vi "Modules - Communications.vi"() -> ()   [LabVIEW 2019]
uses:
  Controls/Communications - State.ctl
  Controls/eFGV States.ctl
  Controls/Communications - Data Structure.ctl
  Controls/FTDI - Communication.ctl
  Controls/Global - Channel.vi
  Controls/Global - Done.vi
  Controls/Global - Unit.vi
  Controls/Global - IP Address.vi
  Controls/Global - Device.vi
  Controls/Global - Handle.vi
  Controls/Global - Comport.vi
  Controls/Global - Hold.vi
  Controls/Global - Rendezvous.vi
  Controls/UDP - Command.ctl
  Controls/Global - ADC.vi
  Controls/Global - PID.vi
  Controls/Communication - Write Data.ctl
  Controls/Global - System.vi
  Controls/Global - Test.vi
panel:
  out "Device":string[](array[string])
  out "IP":string[](array[string])
  out "Stop":bool=TRUE
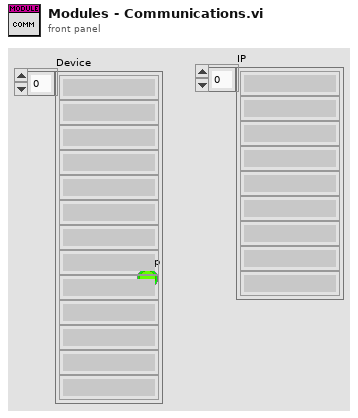
[diagram p1: front panel]
types:
  T1 = typedef "Communications - State.ctl" = enum16{"Init", "Idle", "Command", "Get IP Address", "Release Rendezvous", "Feedback", "Close"}
  T2 = typedef "FTDI - Communication.ctl" = cluster{"IP":string, "CMD":T3, "Port":string, "Datalog?":bool, "Float":dbl}
  T3 = typedef "UDP - Command.ctl" = enum16{"Stop", "Jog Up", "Jog Down", "Ramp Up", "Ramp Down", "PID Target", "PID Ramp", "Disp Run", "Read Ch Data", "Zero Channel", "Zero Disp", "Read Sensor", "Write Sensor", "Read ADC", "Write ADC", "Read PID", "Write PID", "Read Test", "Write Test", "Read System", "Write System", "Read Datalog", "Read Datalog Sensor"}
  T4 = typedef "eFGV States.ctl" = enum16{"Init", "Read", "Write", "Exit"}
  T5 = typedef "Communications - Data Structure.ctl" = cluster{"UDP CMD":T2, "UDP ref":refnum<event-registration>, "Unit?":bool, "Read Unit":bool[], "Trig?":bool, "UDP Info":cluster{"IP Address":string, "port":string, "UDP ref":refnum<k16>}[], "UDP Conn ref":refnum<k16>, "DataLogger":bool[], "VISA Ref":refnum<event-registration>, "Float":sgl, "Data":T6}
  T6 = typedef "Communication - Write Data.ctl" = cluster{"Test":cluster{"Target Load":sgl, "Target Disp":sgl, "Rate":sgl, "Speed":sgl}, "Sensor":cluster{"Name":string[], "Unit":string[], "Decimal Point":u8[], "Ch Log":u8[], "H Alarm":u8[], "L Alarm":u8[], "H Limit":sgl[], "L Limit":sgl[], "Filter":u8[], "Gain":u8[], "Calib Type":u32[]}, "PID":cluster{"SP":sgl, "PV":sgl, "kP":sgl, "kI":sgl, "kD":sgl, "FF":sgl, "Err Band":sgl, "Max":i32, "Min":i32, "Ts":u32, "Out":i32, "Mode":u8}, "ADC":cluster{"Active Ch":u8[], "Filter Type":u8, "Post Filter":u8[], "Gain":u8[], "FS":u16, "IntOC":u8, "IntFC":u8, "SysOC":u8, "Cofficient":dbl[], "K":dbl[], "Max":i32}, "System":cluster{"Out Type":u8, "Inverse":u8, "Monitor":u8, "Reserve":u8, "ACC Time":u32, "Pulse Rev":u32, "Stroke":u32, "Auto Off":u32, "Gear Ratio":sgl, "Pitch":sgl, "Max Speed":u32, "Jog Speed":u32, "Disp Coff":sgl, "Max Load":u32}, "Index":enum16{"Ch1", "Ch2", "Ch3", "Ch4", "Ch5", "Ch6", "Ch7", "Ch8", "Ch9", "Ch10", "Ch11", "Ch12", "Ch13", "Ch14", "Ch15", "Ch16"}, "Datalog":enum16{"Ch1-Ch16", "Ch17-Ch32", "Ch32-Ch48", "Ch49-Ch64", "Empty"}}
  T7 = cluster{"IP Address":string, "port":string, "UDP ref":refnum<k16>}[]
  T8 = cluster{"IP Address":string, "port":string, "UDP ref":refnum<k16>}
  T9 = typedef "UDP - Status.ctl" = u16
  T10 = typedef "UDP - Event.ctl" = u16
  T11 = cluster{"Test":cluster{"Target Load":sgl, "Target Disp":sgl, "Rate":sgl, "Speed":sgl}, "Sensor":cluster{"Name":string[], "Unit":string[], "Decimal Point":u8[], "Ch Log":u8[], "H Alarm":u8[], "L Alarm":u8[], "H Limit":sgl[], "L Limit":sgl[], "Filter":u8[], "Gain":u8[], "Calib Type":u32[]}, "PID":cluster{"SP":sgl, "PV":sgl, "kP":sgl, "kI":sgl, "kD":sgl, "FF":sgl, "Err Band":sgl, "Max":i32, "Min":i32, "Ts":u32, "Out":i32, "Mode":u8}, "ADC":cluster{"Active Ch":u8[], "Filter Type":u8, "Post Filter":u8[], "Gain":u8[], "FS":u16, "IntOC":u8, "IntFC":u8, "SysOC":u8, "Cofficient":dbl[], "K":dbl[], "Max":i32}, "Status":T9, "Event":T10, "System":cluster{"Out Type":u8, "Inverse":u8, "Monitor":u8, "Reserve":u8, "ACC Time":u32, "Pulse Rev":u32, "Stroke":u32, "Auto Off":u32, "Gear Ratio":sgl, "Pitch":sgl, "Max Speed":u32, "Jog Speed":u32, "Disp Coff":sgl, "Max Load":u32}, "Channels":cluster{"Ch1":sgl, "Ch2":sgl, "Ch3":sgl, "Ch4":sgl, "Ch5":sgl, "Ch6":sgl, "Ch7":sgl, "Ch8":sgl, "Ch9":sgl, "Ch10":sgl, "Ch11":sgl, "Ch12":sgl, "Ch13":sgl, "Ch14":sgl, "Ch15":sgl, "Ch16":sgl}}
  T12 = cluster{"Ch1":sgl, "Ch2":sgl, "Ch3":sgl, "Ch4":sgl, "Ch5":sgl, "Ch6":sgl, "Ch7":sgl, "Ch8":sgl, "Ch9":sgl, "Ch10":sgl, "Ch11":sgl, "Ch12":sgl, "Ch13":sgl, "Ch14":sgl, "Ch15":sgl, "Ch16":sgl}
  T13 = cluster{"Channels":cluster{"Ch1":sgl, "Ch2":sgl, "Ch3":sgl, "Ch4":sgl, "Ch5":sgl, "Ch6":sgl, "Ch7":sgl, "Ch8":sgl, "Ch9":sgl, "Ch10":sgl, "Ch11":sgl, "Ch12":sgl, "Ch13":sgl, "Ch14":sgl, "Ch15":sgl, "Ch16":sgl}, "Event":T10, "Status":T9}[]
  T14 = cluster{"Channels":cluster{"Ch1":sgl, "Ch2":sgl, "Ch3":sgl, "Ch4":sgl, "Ch5":sgl, "Ch6":sgl, "Ch7":sgl, "Ch8":sgl, "Ch9":sgl, "Ch10":sgl, "Ch11":sgl, "Ch12":sgl, "Ch13":sgl, "Ch14":sgl, "Ch15":sgl, "Ch16":sgl}, "Event":T10, "Status":T9}
  T15 = cluster{"Name":string[], "Unit":string[], "Decimal Point":u8[], "Ch Log":u8[], "H Alarm":u8[], "L Alarm":u8[], "H Limit":sgl[], "L Limit":sgl[], "Filter":u8[], "Gain":u8[], "Calib Type":u32[]}
  T16 = cluster{"Name":string[], "Unit":string[], "Decimal Point":u8[], "Ch Log":u8[], "H Alarm":u8[], "L Alarm":u8[], "H Limit":sgl[], "L Limit":sgl[], "Filter":u8[], "Gain":u8[], "Calib Type":u32[]}[]
  T17 = cluster{"Active Ch":u8[], "Filter Type":u8, "Post Filter":u8[], "Gain":u8[], "FS":u16, "IntOC":u8, "IntFC":u8, "SysOC":u8, "Cofficient":dbl[], "K":dbl[], "Max":i32}
  T18 = cluster{"Active Ch":u8[], "Filter Type":u8, "Post Filter":u8[], "Gain":u8[], "FS":u16, "IntOC":u8, "IntFC":u8, "SysOC":u8, "Cofficient":dbl[], "K":dbl[], "Max":i32}[]
  T19 = cluster{"SP":sgl, "PV":sgl, "kP":sgl, "kI":sgl, "kD":sgl, "FF":sgl, "Err Band":sgl, "Max":i32, "Min":i32, "Ts":u32, "Out":i32, "Mode":u8}
  T20 = cluster{"SP":sgl, "PV":sgl, "kP":sgl, "kI":sgl, "kD":sgl, "FF":sgl, "Err Band":sgl, "Max":i32, "Min":i32, "Ts":u32, "Out":i32, "Mode":u8}[]
  T21 = cluster{"Out Type":u8, "Inverse":u8, "Monitor":u8, "Reserve":u8, "ACC Time":u32, "Pulse Rev":u32, "Stroke":u32, "Auto Off":u32, "Gear Ratio":sgl, "Pitch":sgl, "Max Speed":u32, "Jog Speed":u32, "Disp Coff":sgl, "Max Load":u32}
  T22 = cluster{"Out Type":u8, "Inverse":u8, "Monitor":u8, "Reserve":u8, "ACC Time":u32, "Pulse Rev":u32, "Stroke":u32, "Auto Off":u32, "Gear Ratio":sgl, "Pitch":sgl, "Max Speed":u32, "Jog Speed":u32, "Disp Coff":sgl, "Max Load":u32}[]
  T23 = cluster{"Target Load":sgl, "Target Disp":sgl, "Rate":sgl, "Speed":sgl}
  T24 = cluster{"Target Load":sgl, "Target Disp":sgl, "Rate":sgl, "Speed":sgl}[]
  T25 = typedef "Rendezvous RefNum" = refnum<k1>
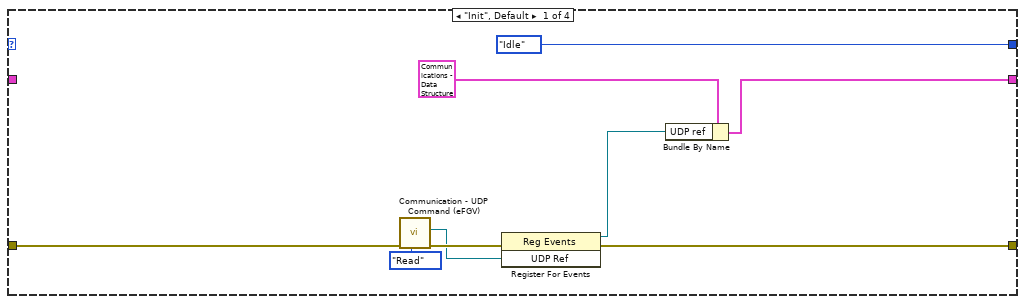
[diagram p2: hidden frame]
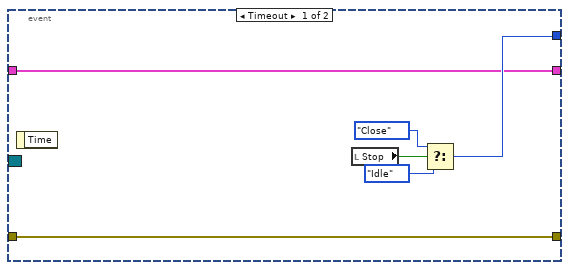
[diagram p3: hidden frame]
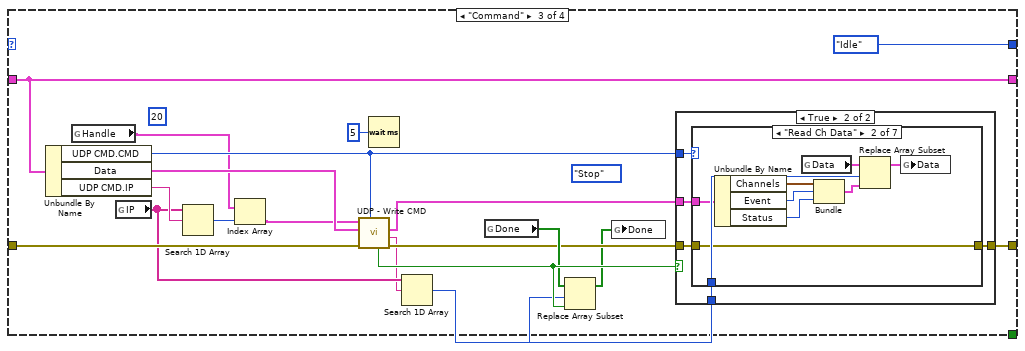
[diagram p4: hidden frame]
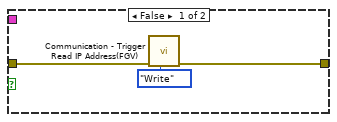
[diagram p5: hidden frame]
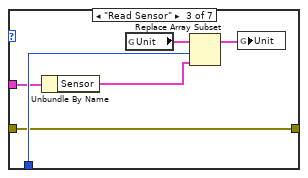
[diagram p7: hidden frame]
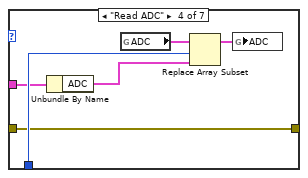
[diagram p8: hidden frame]
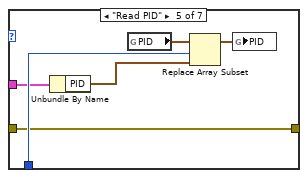
[diagram p9: hidden frame]
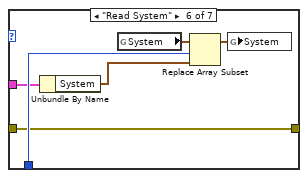
[diagram p10: hidden frame]
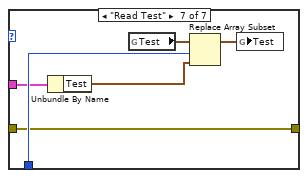
[diagram p11: hidden frame]
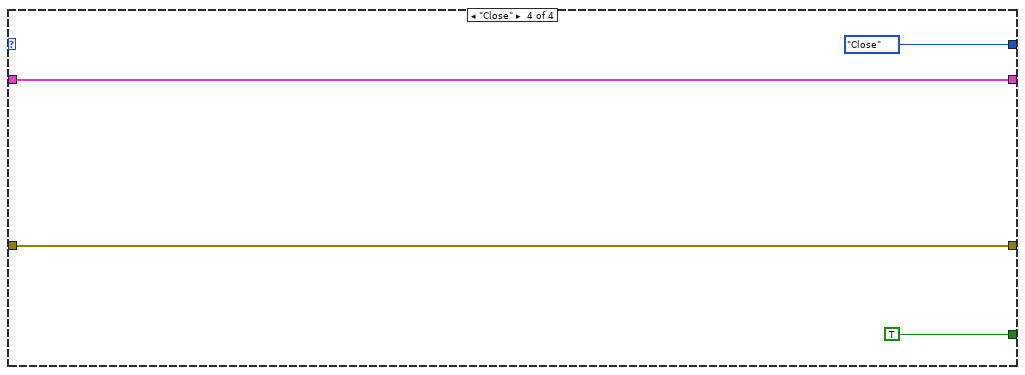
[diagram p12: hidden frame]
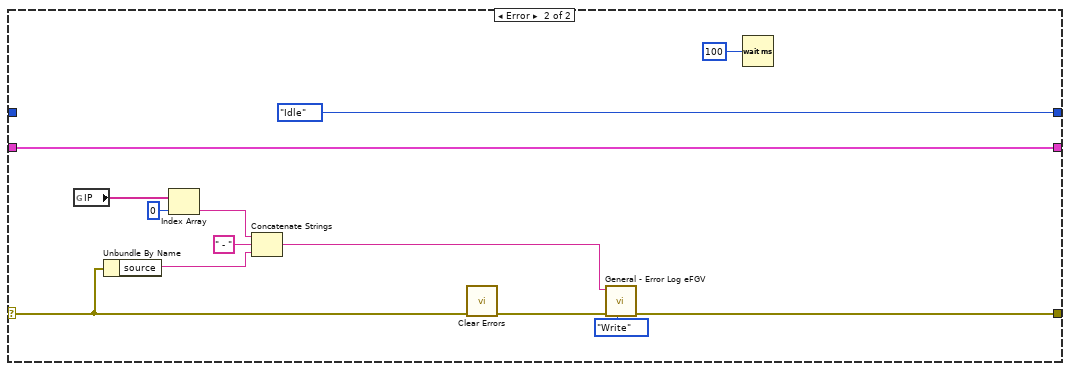
[diagram p13: hidden frame]
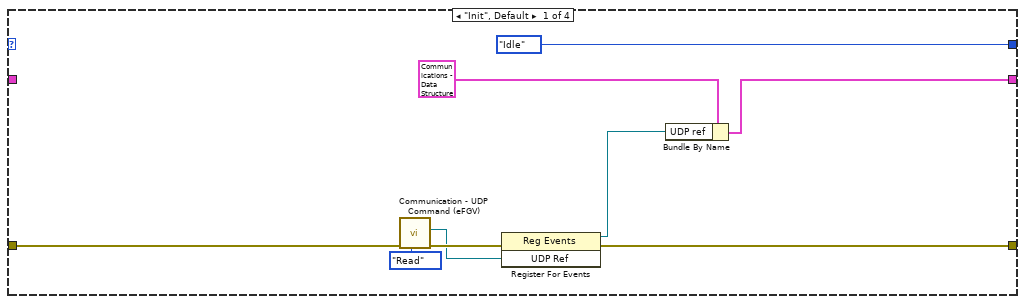
[diagram p14: hidden frame]
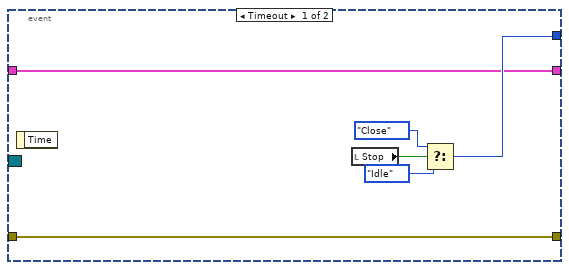
[diagram p15: hidden frame]
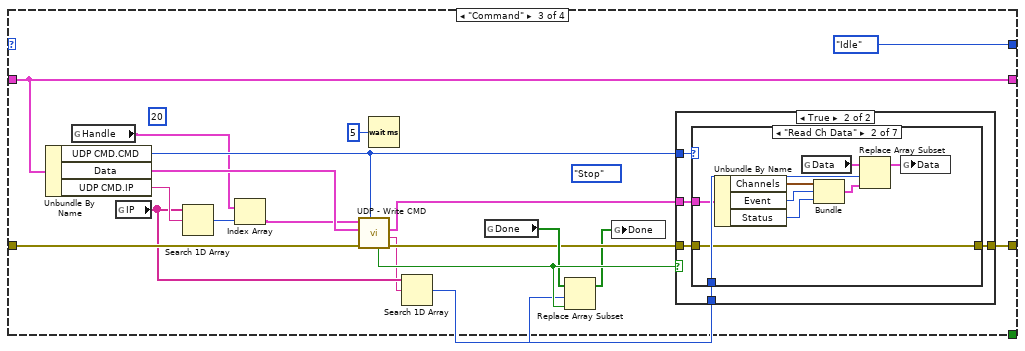
[diagram p16: hidden frame]
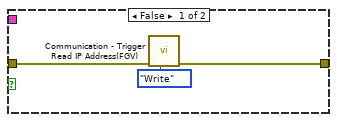
[diagram p17: hidden frame]
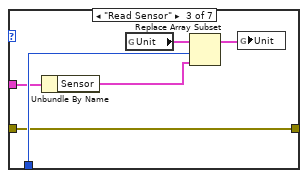
[diagram p19: hidden frame]
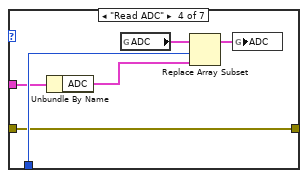
[diagram p20: hidden frame]
diagram:
  (unwired) Communications_-_State."Init"
  (unwired) Communications_-_State."Init"
  (unwired) Communications_-_State."Init"
  (unwired) Communications_-_State."Init"
  (unwired) Communications_-_State."Init"
  (unwired) Communications_-_State."Init"
  (unwired) Communications_-_State."Init"
  (unwired) Communications_-_State."Init"
  (unwired) Communications_-_State."Init"
  (unwired) Communications_-_State."Init"
  (unwired) Communications_-_State."Init"
  (unwired) Communications_-_State."Init"
  (unwired) Communications_-_State."Init"
  (unwired) Communications_-_State."Init"
  (unwired) Communications_-_State."Init"
  (unwired) Communications_-_State."Init"
  (unwired) Communications_-_State."Init"
  (unwired) Communications_-_State."Init"
  (unwired) Communications_-_State."Init"
  (unwired) Communications_-_State."Init"
  (unwired) Communications_-_State."Init"
  (unwired) Communications_-_State."Init"
  (unwired) Communications_-_State."Init"
  (unwired) Communications_-_State."Init"
  (unwired) Communications_-_State."Init"
  (unwired) Communications_-_State."Init"
  (unwired) Communications_-_State."Init"
  (unwired) Communications_-_State."Init"
  (unwired) Communications_-_State."Init"
  (unwired) Communications_-_State."Init"
  (unwired) Communications_-_State."Init"
  (unwired) Communications_-_State."Init"
  (unwired) T2 {"IP"="", "CMD"=enum."Stop", "Port"="", "Datalog?"=FALSE, "Float"=0.0}
  (unwired) Communications_-_State."Init"
  n1 = while {
    shift-right: [w73] -> _
    shift-left: errorcluster {"status"=FALSE, "code"=0, "source"=""} ("error IO") -> [w74]
    shift-right: [w71] -> _
    shift-left: Communications_-_State."Init" -> [w72]
    shift-right: [w69] -> _
    shift-left: _ -> [w68]
    stop <- w70 stop-if-true
    # "Command Processing Loop"
    n2 = case shown="No Error" w74 {
      selector: w74 -> [w80 w198]
      tunnel: [w81 w191] -> w73
      tunnel: w72 -> [w79 _]
      tunnel: [w78 Communications_-_State."Idle"] -> w71
      tunnel: [w77 _] -> w70
      tunnel: [w76 w200] -> w69
      tunnel: w68 -> [w75 w200]
      frame No Error {
        n3 = case shown="\"Idle\"" w79 {
          tunnel: [w84 w98 w132 w188] -> w81
          tunnel: w80 -> [w89 w97 w135 w188]
          tunnel: [Communications_-_State."Idle" w92 Communications_-_State."Idle" Communications_-_State."Close"] -> w78
          tunnel: [_ _ _ TRUE] -> w77
          tunnel: [w86 w96 w134 w185] -> w76
          tunnel: w75 -> [_ w95 w134 w185]
          frame "Init", Default {
            n4 = call "Communication - UDP Command (eFGV).vi"("Action"=eFGV_States."Read", "error in"=w89) -> ("error out"=w85:errorcluster, "UDP Ref"=w83:refnum<user-event>)  [unwired: 7 in, 1 out]
            n5 = register-events(error in=w85, w83) -> (reference out=w82:refnum<event-registration>, error out=w84:errorcluster)  [unwired: 1 in]
            n6 = Bundle By Name(cluster=T5 {"UDP CMD"={"IP"="", "CMD"=enum."Stop", "Port"="", "Datalog?"=FALSE, "Float"=0.0}, "UDP ref"=refnum, "Unit?"=FALSE, "Read Unit"=[], "Trig?"=FALSE, "UDP Info"=[], "UDP Conn ref"=refnum, "DataLogger"=[], "VISA Ref"=refnum, "Float"=0.0, "Data"={"Test"={"Target Load"=0.0, "Target Disp"=0.0, "Rate"=0.0, "Speed"=0.0}, "Sensor"={"Name"=[], "Unit"=[], "Decimal Point"=[], "Ch Log"=[], "H Alarm"=[], "L Alarm"=[], "H Limit"=[], "L Limit"=[], "Filter"=[], "Gain"=[], "Calib Type"=[]}, "PID"={"SP"=0.0, "PV"=0.0, "kP"=0.0, "kI"=0.0, "kD"=0.0, "FF"=0.0, "Err Band"=0.0, "Max"=0, "Min"=0, "Ts"=0, "Out"=0, "Mode"=0}, "ADC"={"Active Ch"=[], "Filter Type"=0, "Post Filter"=[], "Gain"=[], "FS"=0, "IntOC"=0, "IntFC"=0, "SysOC"=0, "Cofficient"=[], "K"=[], "Max"=0}, "System"={"Out Type"=0, "Inverse"=0, "Monitor"=0, "Reserve"=0, "ACC Time"=0, "Pulse Rev"=0, "Stroke"=0, "Auto Off"=0, "Gear Ratio"=0.0, "Pitch"=0.0, "Max Speed"=0, "Jog Speed"=0, "Disp Coff"=0.0, "Max Load"=0}, "Index"=enum."Ch1", "Datalog"=enum."Empty"}}, "UDP ref"=w82) -> (w86:T5)
          }
          frame "Idle" {
            n7 = Unbundle By Name(w95) -> ("UDP ref"=w99:refnum<event-registration>)
            n8 = event shown="[1] <FDTI ref>: User Event" {
              selector: w99 -> [_ _]
              dyn-events: _ -> [_ _]
              timeout: _ -> [_ _]
              tunnel: [w105 w107] -> w93
              tunnel: [w102 _] -> w98
              tunnel: w97 -> [w102 _]
              tunnel: [w100 w117] -> w96
              tunnel: w95 -> [w100 w116]
              event Timeout {
                n9 = event-data() -> ()  [unwired: 1 in, 1 out]
                n10 = local read "Stop"() -> (w104:bool)
                n11 = Select(t=Communications_-_State."Close", s=w104, f=Communications_-_State."Idle") -> (s? t:f=w105:T1)
              }
              event User Event {
                n12 = event-data() -> ("IP"=w110:string, "CMD"=w115:T3, "Data"=w114:T6)  [unwired: 1 in]
                n13 = global read "Global - IP Address.vi" "IP"() -> (w113:string[])
                n14 = Index Array(array=w113, index=28) -> (element=w111:string)
                n15 = Equal?(x=w111, y=w110) -> (x = y?=w109:bool)
                n16 = Bundle By Name(cluster=w116, "UDP CMD.IP"=w110, "UDP CMD.CMD"=w115, "Data"=w114) -> (w117:T5)
                n17 = Select(t=Communications_-_State."Command" ("f"), s=w109, f=Communications_-_State."Idle") -> (s? t:f=w107:T1)
              }
            }
            n18 = global read "Global - Hold.vi" "Hold"() -> (w94:bool)
            n19 = Select(t=Communications_-_State."Idle", s=w94, f=w93) -> (s? t:f=w92:T1)
          }
          frame "Command" {
            (unwired) UDP_-_Command."Stop" ("Enum")
            (unwired) 20
            n20 = Unbundle By Name(w134) -> ("UDP CMD.CMD"=w131:T3, "Data"=w133:T6, "UDP CMD.IP"=w128:string)
            n21 = global read "Global - Handle.vi" "Handle"() -> (w123:T7)
            n22 = global read "Global - IP Address.vi" "IP"() -> (w121:string[])
            n23 = Search 1D Array(1D array=w121, element=w128) -> (index of element=w119:i32)  [unwired: 1 in]
            n24 = Index Array(array=w123, index=w119) -> (element=w127:T8)
            n25 = call "UDP - Write CMD.vi"("CMD"=w131, "error in"=w135, "Data"=w133, "UDP Info"=w127) -> ("error out"=w125:errorcluster, "IP Address"=w120:string, "Data Out"=w130:T11, "Success"=w129:bool)  [unwired: 2 in, 2 out]
            n26 = Wait (ms)(milliseconds to wait=u32 5) -> ()  [unwired: 1 out]
            n27 = Search 1D Array(1D array=w121, element=w120) -> (index of element=w118:i32)  [unwired: 1 in]
            n28 = global read "Global - Done.vi" "Done"() -> (w126:bool[])
            n29 = Replace Array Subset(array=w126, new element=w129, index=w118) -> (w124:bool[])
            n30 = global write "Global - Done.vi" "Done"(w124) -> ()
            n31 = case shown="True" w129 {
              tunnel: w125 -> [w137 w143]
              tunnel: [w138 w142] -> w132
              tunnel: w131 -> [_ w144]
              tunnel: w130 -> [_ w141]
              tunnel: w118 -> [_ w140]
              frame False {
                n32 = call "Communication - Trigger Read IP Address(FGV).vi"("Action"=eFGV_States."Write", "error in"=w137) -> ("error out"=w138:errorcluster)  [unwired: 7 in, 2 out]
              }
              frame True {
                n33 = case shown="\"Read Ch Data\"" w144 {
                  tunnel: w143 -> [w145 w152 w159 w165 w171 w177 w183]
                  tunnel: [w145 w152 w159 w165 w171 w177 w183] -> w142
                  tunnel: w141 -> [_ w150 w156 w164 w170 w176 w182]
                  tunnel: w140 -> [_ w154 w160 w166 w172 w178 w184]
                  frame "Stop", Default {
                  }
                  frame "Read Ch Data" {
                    n34 = Unbundle By Name(w150) -> ("Channels"=w149:T12, "Event"=w148:T10, "Status"=w147:T9)
                    n35 = global read "Global - Channel.vi" "Data"() -> (w153:T13)
                    n36 = Bundle("Channels"=w149, "Event"=w148, "Status"=w147) -> (w146:T14)  [unwired: 1 in]
                    n37 = Replace Array Subset(array=w153, new element=w146, index=w154) -> (w151:T13)
                    n38 = global write "Global - Channel.vi" "Data"(w151) -> ()
                  }
                  frame "Read Sensor" {
                    n39 = Unbundle By Name(w156) -> ("Sensor"=w155:T15)
                    n40 = global read "Global - Unit.vi" "Unit"() -> (w157:T16)
                    n41 = Replace Array Subset(array=w157, new element=w155, index=w160) -> (w158:T16)
                    n42 = global write "Global - Unit.vi" "Unit"(w158) -> ()
                  }
                  frame "Read ADC" {
                    n43 = Unbundle By Name(w164) -> ("ADC"=w161:T17)
                    n44 = global read "Global - ADC.vi" "ADC"() -> (w163:T18)
                    n45 = Replace Array Subset(array=w163, new element=w161, index=w166) -> (w162:T18)
                    n46 = global write "Global - ADC.vi" "ADC"(w162) -> ()
                  }
                  frame "Read PID" {
                    n47 = Unbundle By Name(w170) -> ("PID"=w167:T19)
                    n48 = global read "Global - PID.vi" "PID"() -> (w169:T20)
                    n49 = Replace Array Subset(array=w169, new element=w167, index=w172) -> (w168:T20)
                    n50 = global write "Global - PID.vi" "PID"(w168) -> ()
                  }
                  frame "Read System" {
                    n51 = Unbundle By Name(w176) -> ("System"=w174:T21)
                    n52 = global read "Global - System.vi" "System"() -> (w175:T22)
                    n53 = Replace Array Subset(array=w175, new element=w174, index=w178) -> (w173:T22)
                    n54 = global write "Global - System.vi" "System"(w173) -> ()
                  }
                  frame "Read Test" {
                    n55 = Unbundle By Name(w182) -> ("Test"=w179:T23)
                    n56 = global read "Global - Test.vi" "Test"() -> (w180:T24)
                    n57 = Replace Array Subset(array=w180, new element=w179, index=w184) -> (w181:T24)
                    n58 = global write "Global - Test.vi" "Test"(w181) -> ()
                  }
                }
              }
            }
          }
          frame "Close" {
          }
        }
      }
      frame Error {
        n59 = global read "Global - IP Address.vi" "IP"() -> (w197:string[])
        n60 = Unbundle By Name(w198) -> ("source"=w193:string)
        n61 = Index Array(array=w197, index=0) -> (element=w195:string)
        n62 = Concatenate Strings(w195, " - " ("string"), w193) -> (w189:string)
        n63 = call <vilib>:"Clear Errors.vi"("error in (no error)"=w198) -> ("error out"=w192:errorcluster)  [unwired: 5 in, 1 out]
        n64 = call "General - Error Log eFGV.vi"("eFGV States"=eFGV_States."Write", "error in (no error)"=w192, "Error In"=w189) -> ("error out"=w191:errorcluster)  [unwired: 6 in, 2 out]
        n65 = Wait (ms)(milliseconds to wait=u32 100) -> ()  [unwired: 1 out]
      }
    }
  }
  n66 = while {
    shift-right: [w207] -> _
    shift-left: errorcluster {"status"=FALSE, "code"=0, "source"=""} ("error IO") -> [w208]
    shift-right: [w205] -> _
    shift-left: Communications_-_State."Init" -> [w206]
    shift-right: [w203] -> _
    shift-left: _ -> [w202]
    stop <- w204 stop-if-true
    # "Command Processing Loop"
    n67 = case shown="No Error" w208 {
      selector: w208 -> [w214 w332]
      tunnel: [w215 w325] -> w207
      tunnel: w206 -> [w213 _]
      tunnel: [w212 Communications_-_State."Idle"] -> w205
      tunnel: [w211 _] -> w204
      tunnel: [w210 w334] -> w203
      tunnel: w202 -> [w209 w334]
      frame No Error {
        n68 = case shown="\"Idle\"" w213 {
          tunnel: [w218 w232 w266 w322] -> w215
          tunnel: w214 -> [w223 w231 w269 w322]
          tunnel: [Communications_-_State."Idle" w226 Communications_-_State."Idle" Communications_-_State."Close"] -> w212
          tunnel: [_ _ _ TRUE] -> w211
          tunnel: [w220 w230 w268 w319] -> w210
          tunnel: w209 -> [_ w229 w268 w319]
          frame "Init", Default {
            n69 = call "Communication - UDP Command (eFGV).vi"("Action"=eFGV_States."Read", "error in"=w223) -> ("error out"=w219:errorcluster, "UDP Ref"=w217:refnum<user-event>)  [unwired: 7 in, 1 out]
            n70 = register-events(error in=w219, w217) -> (reference out=w216:refnum<event-registration>, error out=w218:errorcluster)  [unwired: 1 in]
            n71 = Bundle By Name(cluster=T5 {"UDP CMD"={"IP"="", "CMD"=enum."Stop", "Port"="", "Datalog?"=FALSE, "Float"=0.0}, "UDP ref"=refnum, "Unit?"=FALSE, "Read Unit"=[], "Trig?"=FALSE, "UDP Info"=[], "UDP Conn ref"=refnum, "DataLogger"=[], "VISA Ref"=refnum, "Float"=0.0, "Data"={"Test"={"Target Load"=0.0, "Target Disp"=0.0, "Rate"=0.0, "Speed"=0.0}, "Sensor"={"Name"=[], "Unit"=[], "Decimal Point"=[], "Ch Log"=[], "H Alarm"=[], "L Alarm"=[], "H Limit"=[], "L Limit"=[], "Filter"=[], "Gain"=[], "Calib Type"=[]}, "PID"={"SP"=0.0, "PV"=0.0, "kP"=0.0, "kI"=0.0, "kD"=0.0, "FF"=0.0, "Err Band"=0.0, "Max"=0, "Min"=0, "Ts"=0, "Out"=0, "Mode"=0}, "ADC"={"Active Ch"=[], "Filter Type"=0, "Post Filter"=[], "Gain"=[], "FS"=0, "IntOC"=0, "IntFC"=0, "SysOC"=0, "Cofficient"=[], "K"=[], "Max"=0}, "System"={"Out Type"=0, "Inverse"=0, "Monitor"=0, "Reserve"=0, "ACC Time"=0, "Pulse Rev"=0, "Stroke"=0, "Auto Off"=0, "Gear Ratio"=0.0, "Pitch"=0.0, "Max Speed"=0, "Jog Speed"=0, "Disp Coff"=0.0, "Max Load"=0}, "Index"=enum."Ch1", "Datalog"=enum."Empty"}}, "UDP ref"=w216) -> (w220:T5)
          }
          frame "Idle" {
            n72 = Unbundle By Name(w229) -> ("UDP ref"=w233:refnum<event-registration>)
            n73 = event shown="[1] <FDTI ref>: User Event" {
              selector: w233 -> [_ _]
              dyn-events: _ -> [_ _]
              timeout: _ -> [_ _]
              tunnel: [w239 w241] -> w227
              tunnel: [w236 _] -> w232
              tunnel: w231 -> [w236 _]
              tunnel: [w234 w251] -> w230
              tunnel: w229 -> [w234 w250]
              event Timeout {
                n74 = event-data() -> ()  [unwired: 1 in, 1 out]
                n75 = local read "Stop"() -> (w238:bool)
                n76 = Select(t=Communications_-_State."Close", s=w238, f=Communications_-_State."Idle") -> (s? t:f=w239:T1)
              }
              event User Event {
                n77 = event-data() -> ("IP"=w244:string, "CMD"=w249:T3, "Data"=w248:T6)  [unwired: 1 in]
                n78 = global read "Global - IP Address.vi" "IP"() -> (w247:string[])
                n79 = Index Array(array=w247, index=30) -> (element=w245:string)
                n80 = Equal?(x=w245, y=w244) -> (x = y?=w243:bool)
                n81 = Bundle By Name(cluster=w250, "UDP CMD.IP"=w244, "UDP CMD.CMD"=w249, "Data"=w248) -> (w251:T5)
                n82 = Select(t=Communications_-_State."Command" ("f"), s=w243, f=Communications_-_State."Idle") -> (s? t:f=w241:T1)
              }
            }
            n83 = global read "Global - Hold.vi" "Hold"() -> (w228:bool)
            n84 = Select(t=Communications_-_State."Idle", s=w228, f=w227) -> (s? t:f=w226:T1)
          }
          frame "Command" {
            (unwired) UDP_-_Command."Stop" ("Enum")
            (unwired) 20
            n85 = Unbundle By Name(w268) -> ("UDP CMD.CMD"=w265:T3, "Data"=w267:T6, "UDP CMD.IP"=w262:string)
            n86 = global read "Global - Handle.vi" "Handle"() -> (w257:T7)
            n87 = global read "Global - IP Address.vi" "IP"() -> (w255:string[])
            n88 = Search 1D Array(1D array=w255, element=w262) -> (index of element=w253:i32)  [unwired: 1 in]
            n89 = Index Array(array=w257, index=w253) -> (element=w261:T8)
            n90 = call "UDP - Write CMD.vi"("CMD"=w265, "error in"=w269, "Data"=w267, "UDP Info"=w261) -> ("error out"=w259:errorcluster, "IP Address"=w254:string, "Data Out"=w264:T11, "Success"=w263:bool)  [unwired: 2 in, 2 out]
            n91 = Wait (ms)(milliseconds to wait=u32 5) -> ()  [unwired: 1 out]
            n92 = Search 1D Array(1D array=w255, element=w254) -> (index of element=w252:i32)  [unwired: 1 in]
            n93 = global read "Global - Done.vi" "Done"() -> (w260:bool[])
            n94 = Replace Array Subset(array=w260, new element=w263, index=w252) -> (w258:bool[])
            n95 = global write "Global - Done.vi" "Done"(w258) -> ()
            n96 = case shown="True" w263 {
              tunnel: w259 -> [w271 w277]
              tunnel: [w272 w276] -> w266
              tunnel: w265 -> [_ w278]
              tunnel: w264 -> [_ w275]
              tunnel: w252 -> [_ w274]
              frame False {
                n97 = call "Communication - Trigger Read IP Address(FGV).vi"("Action"=eFGV_States."Write", "error in"=w271) -> ("error out"=w272:errorcluster)  [unwired: 7 in, 2 out]
              }
              frame True {
                n98 = case shown="\"Read Ch Data\"" w278 {
                  tunnel: w277 -> [w279 w286 w293 w299 w305 w311 w317]
                  tunnel: [w279 w286 w293 w299 w305 w311 w317] -> w276
                  tunnel: w275 -> [_ w284 w290 w298 w304 w310 w316]
                  tunnel: w274 -> [_ w288 w294 w300 w306 w312 w318]
                  frame "Stop", Default {
                  }
                  frame "Read Ch Data" {
                    n99 = Unbundle By Name(w284) -> ("Channels"=w283:T12, "Event"=w282:T10, "Status"=w281:T9)
                    n100 = global read "Global - Channel.vi" "Data"() -> (w287:T13)
                    n101 = Bundle("Channels"=w283, "Event"=w282, "Status"=w281) -> (w280:T14)  [unwired: 1 in]
                    n102 = Replace Array Subset(array=w287, new element=w280, index=w288) -> (w285:T13)
                    n103 = global write "Global - Channel.vi" "Data"(w285) -> ()
                  }
                  frame "Read Sensor" {
                    n104 = Unbundle By Name(w290) -> ("Sensor"=w289:T15)
                    n105 = global read "Global - Unit.vi" "Unit"() -> (w291:T16)
                    n106 = Replace Array Subset(array=w291, new element=w289, index=w294) -> (w292:T16)
                    n107 = global write "Global - Unit.vi" "Unit"(w292) -> ()
                  }
                  frame "Read ADC" {
                    n108 = Unbundle By Name(w298) -> ("ADC"=w295:T17)
                    n109 = global read "Global - ADC.vi" "ADC"() -> (w297:T18)
                    n110 = Replace Array Subset(array=w297, new element=w295, index=w300) -> (w296:T18)
                    n111 = global write "Global - ADC.vi" "ADC"(w296) -> ()
                  }
                  frame "Read PID" {
                    n112 = Unbundle By Name(w304) -> ("PID"=w301:T19)
                    n113 = global read "Global - PID.vi" "PID"() -> (w303:T20)
                    n114 = Replace Array Subset(array=w303, new element=w301, index=w306) -> (w302:T20)
                    n115 = global write "Global - PID.vi" "PID"(w302) -> ()
                  }
                  frame "Read System" {
                    n116 = Unbundle By Name(w310) -> ("System"=w308:T21)
                    n117 = global read "Global - System.vi" "System"() -> (w309:T22)
                    n118 = Replace Array Subset(array=w309, new element=w308, index=w312) -> (w307:T22)
                    n119 = global write "Global - System.vi" "System"(w307) -> ()
                  }
                  frame "Read Test" {
                    n120 = Unbundle By Name(w316) -> ("Test"=w313:T23)
                    n121 = global read "Global - Test.vi" "Test"() -> (w314:T24)
                    n122 = Replace Array Subset(array=w314, new element=w313, index=w318) -> (w315:T24)
                    n123 = global write "Global - Test.vi" "Test"(w315) -> ()
                  }
                }
              }
            }
          }
          frame "Close" {
          }
        }
      }
      frame Error {
        n124 = global read "Global - IP Address.vi" "IP"() -> (w331:string[])
        n125 = Unbundle By Name(w332) -> ("source"=w327:string)
        n126 = Index Array(array=w331, index=0) -> (element=w329:string)
        n127 = Concatenate Strings(w329, " - " ("string"), w327) -> (w323:string)
        n128 = call <vilib>:"Clear Errors.vi"("error in (no error)"=w332) -> ("error out"=w326:errorcluster)  [unwired: 5 in, 1 out]
        n129 = call "General - Error Log eFGV.vi"("eFGV States"=eFGV_States."Write", "error in (no error)"=w326, "Error In"=w323) -> ("error out"=w325:errorcluster)  [unwired: 6 in, 2 out]
        n130 = Wait (ms)(milliseconds to wait=u32 100) -> ()  [unwired: 1 out]
      }
    }
  }
  n131 = while {
    shift-right: [w341] -> _
    shift-left: errorcluster {"status"=FALSE, "code"=0, "source"=""} ("error IO") -> [w342]
    shift-right: [w339] -> _
    shift-left: Communications_-_State."Init" -> [w340]
    shift-right: [w337] -> _
    shift-left: _ -> [w336]
    stop <- w338 stop-if-true
    # "Command Processing Loop"
    n132 = case shown="No Error" w342 {
      selector: w342 -> [w348 w466]
      tunnel: [w349 w459] -> w341
      tunnel: w340 -> [w347 _]
      tunnel: [w346 Communications_-_State."Idle"] -> w339
      tunnel: [w345 _] -> w338
      tunnel: [w344 w468] -> w337
      tunnel: w336 -> [w343 w468]
      frame No Error {
        n133 = case shown="\"Idle\"" w347 {
          tunnel: [w352 w366 w400 w456] -> w349
          tunnel: w348 -> [w357 w365 w403 w456]
          tunnel: [Communications_-_State."Idle" w360 Communications_-_State."Idle" Communications_-_State."Close"] -> w346
          tunnel: [_ _ _ TRUE] -> w345
          tunnel: [w354 w364 w402 w453] -> w344
          tunnel: w343 -> [_ w363 w402 w453]
          frame "Init", Default {
            n134 = call "Communication - UDP Command (eFGV).vi"("Action"=eFGV_States."Read", "error in"=w357) -> ("error out"=w353:errorcluster, "UDP Ref"=w351:refnum<user-event>)  [unwired: 7 in, 1 out]
            n135 = register-events(error in=w353, w351) -> (reference out=w350:refnum<event-registration>, error out=w352:errorcluster)  [unwired: 1 in]
            n136 = Bundle By Name(cluster=T5 {"UDP CMD"={"IP"="", "CMD"=enum."Stop", "Port"="", "Datalog?"=FALSE, "Float"=0.0}, "UDP ref"=refnum, "Unit?"=FALSE, "Read Unit"=[], "Trig?"=FALSE, "UDP Info"=[], "UDP Conn ref"=refnum, "DataLogger"=[], "VISA Ref"=refnum, "Float"=0.0, "Data"={"Test"={"Target Load"=0.0, "Target Disp"=0.0, "Rate"=0.0, "Speed"=0.0}, "Sensor"={"Name"=[], "Unit"=[], "Decimal Point"=[], "Ch Log"=[], "H Alarm"=[], "L Alarm"=[], "H Limit"=[], "L Limit"=[], "Filter"=[], "Gain"=[], "Calib Type"=[]}, "PID"={"SP"=0.0, "PV"=0.0, "kP"=0.0, "kI"=0.0, "kD"=0.0, "FF"=0.0, "Err Band"=0.0, "Max"=0, "Min"=0, "Ts"=0, "Out"=0, "Mode"=0}, "ADC"={"Active Ch"=[], "Filter Type"=0, "Post Filter"=[], "Gain"=[], "FS"=0, "IntOC"=0, "IntFC"=0, "SysOC"=0, "Cofficient"=[], "K"=[], "Max"=0}, "System"={"Out Type"=0, "Inverse"=0, "Monitor"=0, "Reserve"=0, "ACC Time"=0, "Pulse Rev"=0, "Stroke"=0, "Auto Off"=0, "Gear Ratio"=0.0, "Pitch"=0.0, "Max Speed"=0, "Jog Speed"=0, "Disp Coff"=0.0, "Max Load"=0}, "Index"=enum."Ch1", "Datalog"=enum."Empty"}}, "UDP ref"=w350) -> (w354:T5)
          }
          frame "Idle" {
            n137 = Unbundle By Name(w363) -> ("UDP ref"=w367:refnum<event-registration>)
            n138 = event shown="[1] <FDTI ref>: User Event" {
              selector: w367 -> [_ _]
              dyn-events: _ -> [_ _]
              timeout: _ -> [_ _]
              tunnel: [w373 w375] -> w361
              tunnel: [w370 _] -> w366
              tunnel: w365 -> [w370 _]
              tunnel: [w368 w385] -> w364
              tunnel: w363 -> [w368 w384]
              event Timeout {
                n139 = event-data() -> ()  [unwired: 1 in, 1 out]
                n140 = local read "Stop"() -> (w372:bool)
                n141 = Select(t=Communications_-_State."Close", s=w372, f=Communications_-_State."Idle") -> (s? t:f=w373:T1)
              }
              event User Event {
                n142 = event-data() -> ("IP"=w378:string, "CMD"=w383:T3, "Data"=w382:T6)  [unwired: 1 in]
                n143 = global read "Global - IP Address.vi" "IP"() -> (w381:string[])
                n144 = Index Array(array=w381, index=24) -> (element=w379:string)
                n145 = Equal?(x=w379, y=w378) -> (x = y?=w377:bool)
                n146 = Bundle By Name(cluster=w384, "UDP CMD.IP"=w378, "UDP CMD.CMD"=w383, "Data"=w382) -> (w385:T5)
                n147 = Select(t=Communications_-_State."Command" ("f"), s=w377, f=Communications_-_State."Idle") -> (s? t:f=w375:T1)
              }
            }
            n148 = global read "Global - Hold.vi" "Hold"() -> (w362:bool)
            n149 = Select(t=Communications_-_State."Idle", s=w362, f=w361) -> (s? t:f=w360:T1)
          }
          frame "Command" {
            (unwired) UDP_-_Command."Stop" ("Enum")
            (unwired) 20
            n150 = Unbundle By Name(w402) -> ("UDP CMD.CMD"=w399:T3, "Data"=w401:T6, "UDP CMD.IP"=w396:string)
            n151 = global read "Global - Handle.vi" "Handle"() -> (w391:T7)
            n152 = global read "Global - IP Address.vi" "IP"() -> (w389:string[])
            n153 = Search 1D Array(1D array=w389, element=w396) -> (index of element=w387:i32)  [unwired: 1 in]
            n154 = Index Array(array=w391, index=w387) -> (element=w395:T8)
            n155 = call "UDP - Write CMD.vi"("CMD"=w399, "error in"=w403, "Data"=w401, "UDP Info"=w395) -> ("error out"=w393:errorcluster, "IP Address"=w388:string, "Data Out"=w398:T11, "Success"=w397:bool)  [unwired: 2 in, 2 out]
            n156 = Wait (ms)(milliseconds to wait=u32 5) -> ()  [unwired: 1 out]
            n157 = Search 1D Array(1D array=w389, element=w388) -> (index of element=w386:i32)  [unwired: 1 in]
            n158 = global read "Global - Done.vi" "Done"() -> (w394:bool[])
            n159 = Replace Array Subset(array=w394, new element=w397, index=w386) -> (w392:bool[])
            n160 = global write "Global - Done.vi" "Done"(w392) -> ()
            n161 = case shown="True" w397 {
              tunnel: w393 -> [w405 w411]
              tunnel: [w406 w410] -> w400
              tunnel: w399 -> [_ w412]
              tunnel: w398 -> [_ w409]
              tunnel: w386 -> [_ w408]
              frame False {
                n162 = call "Communication - Trigger Read IP Address(FGV).vi"("Action"=eFGV_States."Write", "error in"=w405) -> ("error out"=w406:errorcluster)  [unwired: 7 in, 2 out]
              }
              frame True {
                n163 = case shown="\"Read Ch Data\"" w412 {
                  tunnel: w411 -> [w413 w420 w427 w433 w439 w445 w451]
                  tunnel: [w413 w420 w427 w433 w439 w445 w451] -> w410
                  tunnel: w409 -> [_ w418 w424 w432 w438 w444 w450]
                  tunnel: w408 -> [_ w422 w428 w434 w440 w446 w452]
                  frame "Stop", Default {
                  }
                  frame "Read Ch Data" {
                    n164 = Unbundle By Name(w418) -> ("Channels"=w417:T12, "Event"=w416:T10, "Status"=w415:T9)
                    n165 = global read "Global - Channel.vi" "Data"() -> (w421:T13)
                    n166 = Bundle("Channels"=w417, "Event"=w416, "Status"=w415) -> (w414:T14)  [unwired: 1 in]
                    n167 = Replace Array Subset(array=w421, new element=w414, index=w422) -> (w419:T13)
                    n168 = global write "Global - Channel.vi" "Data"(w419) -> ()
                  }
                  frame "Read Sensor" {
                    n169 = Unbundle By Name(w424) -> ("Sensor"=w423:T15)
                    n170 = global read "Global - Unit.vi" "Unit"() -> (w425:T16)
                    n171 = Replace Array Subset(array=w425, new element=w423, index=w428) -> (w426:T16)
                    n172 = global write "Global - Unit.vi" "Unit"(w426) -> ()
                  }
                  frame "Read ADC" {
                    n173 = Unbundle By Name(w432) -> ("ADC"=w429:T17)
                    n174 = global read "Global - ADC.vi" "ADC"() -> (w431:T18)
                    n175 = Replace Array Subset(array=w431, new element=w429, index=w434) -> (w430:T18)
                    n176 = global write "Global - ADC.vi" "ADC"(w430) -> ()
                  }
                  frame "Read PID" {
                    n177 = Unbundle By Name(w438) -> ("PID"=w435:T19)
                    n178 = global read "Global - PID.vi" "PID"() -> (w437:T20)
                    n179 = Replace Array Subset(array=w437, new element=w435, index=w440) -> (w436:T20)
                    n180 = global write "Global - PID.vi" "PID"(w436) -> ()
                  }
                  frame "Read System" {
                    n181 = Unbundle By Name(w444) -> ("System"=w442:T21)
                    n182 = global read "Global - System.vi" "System"() -> (w443:T22)
                    n183 = Replace Array Subset(array=w443, new element=w442, index=w446) -> (w441:T22)
                    n184 = global write "Global - System.vi" "System"(w441) -> ()
                  }
                  frame "Read Test" {
                    n185 = Unbundle By Name(w450) -> ("Test"=w447:T23)
                    n186 = global read "Global - Test.vi" "Test"() -> (w448:T24)
                    n187 = Replace Array Subset(array=w448, new element=w447, index=w452) -> (w449:T24)
                    n188 = global write "Global - Test.vi" "Test"(w449) -> ()
                  }
                }
              }
            }
          }
          frame "Close" {
          }
        }
      }
      frame Error {
        n189 = global read "Global - IP Address.vi" "IP"() -> (w465:string[])
        n190 = Unbundle By Name(w466) -> ("source"=w461:string)
        n191 = Index Array(array=w465, index=0) -> (element=w463:string)
        n192 = Concatenate Strings(w463, " - " ("string"), w461) -> (w457:string)
        n193 = call <vilib>:"Clear Errors.vi"("error in (no error)"=w466) -> ("error out"=w460:errorcluster)  [unwired: 5 in, 1 out]
        n194 = call "General - Error Log eFGV.vi"("eFGV States"=eFGV_States."Write", "error in (no error)"=w460, "Error In"=w457) -> ("error out"=w459:errorcluster)  [unwired: 6 in, 2 out]
        n195 = Wait (ms)(milliseconds to wait=u32 100) -> ()  [unwired: 1 out]
      }
    }
  }
  n196 = while {
    shift-right: [w475] -> _
    shift-left: errorcluster {"status"=FALSE, "code"=0, "source"=""} ("error IO") -> [w476]
    shift-right: [w473] -> _
    shift-left: Communications_-_State."Init" -> [w474]
    shift-right: [w471] -> _
    shift-left: _ -> [w470]
    stop <- w472 stop-if-true
    # "Command Processing Loop"
    n197 = case shown="No Error" w476 {
      selector: w476 -> [w482 w600]
      tunnel: [w483 w593] -> w475
      tunnel: w474 -> [w481 _]
      tunnel: [w480 Communications_-_State."Idle"] -> w473
      tunnel: [w479 _] -> w472
      tunnel: [w478 w602] -> w471
      tunnel: w470 -> [w477 w602]
      frame No Error {
        n198 = case shown="\"Idle\"" w481 {
          tunnel: [w486 w500 w534 w590] -> w483
          tunnel: w482 -> [w491 w499 w537 w590]
          tunnel: [Communications_-_State."Idle" w494 Communications_-_State."Idle" Communications_-_State."Close"] -> w480
          tunnel: [_ _ _ TRUE] -> w479
          tunnel: [w488 w498 w536 w587] -> w478
          tunnel: w477 -> [_ w497 w536 w587]
          frame "Init", Default {
            n199 = call "Communication - UDP Command (eFGV).vi"("Action"=eFGV_States."Read", "error in"=w491) -> ("error out"=w487:errorcluster, "UDP Ref"=w485:refnum<user-event>)  [unwired: 7 in, 1 out]
            n200 = register-events(error in=w487, w485) -> (reference out=w484:refnum<event-registration>, error out=w486:errorcluster)  [unwired: 1 in]
            n201 = Bundle By Name(cluster=T5 {"UDP CMD"={"IP"="", "CMD"=enum."Stop", "Port"="", "Datalog?"=FALSE, "Float"=0.0}, "UDP ref"=refnum, "Unit?"=FALSE, "Read Unit"=[], "Trig?"=FALSE, "UDP Info"=[], "UDP Conn ref"=refnum, "DataLogger"=[], "VISA Ref"=refnum, "Float"=0.0, "Data"={"Test"={"Target Load"=0.0, "Target Disp"=0.0, "Rate"=0.0, "Speed"=0.0}, "Sensor"={"Name"=[], "Unit"=[], "Decimal Point"=[], "Ch Log"=[], "H Alarm"=[], "L Alarm"=[], "H Limit"=[], "L Limit"=[], "Filter"=[], "Gain"=[], "Calib Type"=[]}, "PID"={"SP"=0.0, "PV"=0.0, "kP"=0.0, "kI"=0.0, "kD"=0.0, "FF"=0.0, "Err Band"=0.0, "Max"=0, "Min"=0, "Ts"=0, "Out"=0, "Mode"=0}, "ADC"={"Active Ch"=[], "Filter Type"=0, "Post Filter"=[], "Gain"=[], "FS"=0, "IntOC"=0, "IntFC"=0, "SysOC"=0, "Cofficient"=[], "K"=[], "Max"=0}, "System"={"Out Type"=0, "Inverse"=0, "Monitor"=0, "Reserve"=0, "ACC Time"=0, "Pulse Rev"=0, "Stroke"=0, "Auto Off"=0, "Gear Ratio"=0.0, "Pitch"=0.0, "Max Speed"=0, "Jog Speed"=0, "Disp Coff"=0.0, "Max Load"=0}, "Index"=enum."Ch1", "Datalog"=enum."Empty"}}, "UDP ref"=w484) -> (w488:T5)
          }
          frame "Idle" {
            n202 = Unbundle By Name(w497) -> ("UDP ref"=w501:refnum<event-registration>)
            n203 = event shown="[1] <FDTI ref>: User Event" {
              selector: w501 -> [_ _]
              dyn-events: _ -> [_ _]
              timeout: _ -> [_ _]
              tunnel: [w507 w509] -> w495
              tunnel: [w504 _] -> w500
              tunnel: w499 -> [w504 _]
              tunnel: [w502 w519] -> w498
              tunnel: w497 -> [w502 w518]
              event Timeout {
                n204 = event-data() -> ()  [unwired: 1 in, 1 out]
                n205 = local read "Stop"() -> (w506:bool)
                n206 = Select(t=Communications_-_State."Close", s=w506, f=Communications_-_State."Idle") -> (s? t:f=w507:T1)
              }
              event User Event {
                n207 = event-data() -> ("IP"=w512:string, "CMD"=w517:T3, "Data"=w516:T6)  [unwired: 1 in]
                n208 = global read "Global - IP Address.vi" "IP"() -> (w515:string[])
                n209 = Index Array(array=w515, index=26) -> (element=w513:string)
                n210 = Equal?(x=w513, y=w512) -> (x = y?=w511:bool)
                n211 = Bundle By Name(cluster=w518, "UDP CMD.IP"=w512, "UDP CMD.CMD"=w517, "Data"=w516) -> (w519:T5)
                n212 = Select(t=Communications_-_State."Command" ("f"), s=w511, f=Communications_-_State."Idle") -> (s? t:f=w509:T1)
              }
            }
            n213 = global read "Global - Hold.vi" "Hold"() -> (w496:bool)
            n214 = Select(t=Communications_-_State."Idle", s=w496, f=w495) -> (s? t:f=w494:T1)
          }
          frame "Command" {
            (unwired) UDP_-_Command."Stop" ("Enum")
            (unwired) 20
            n215 = Unbundle By Name(w536) -> ("UDP CMD.CMD"=w533:T3, "Data"=w535:T6, "UDP CMD.IP"=w530:string)
            n216 = global read "Global - Handle.vi" "Handle"() -> (w525:T7)
            n217 = global read "Global - IP Address.vi" "IP"() -> (w523:string[])
            n218 = Search 1D Array(1D array=w523, element=w530) -> (index of element=w521:i32)  [unwired: 1 in]
            n219 = Index Array(array=w525, index=w521) -> (element=w529:T8)
            n220 = call "UDP - Write CMD.vi"("CMD"=w533, "error in"=w537, "Data"=w535, "UDP Info"=w529) -> ("error out"=w527:errorcluster, "IP Address"=w522:string, "Data Out"=w532:T11, "Success"=w531:bool)  [unwired: 2 in, 2 out]
            n221 = Wait (ms)(milliseconds to wait=u32 5) -> ()  [unwired: 1 out]
            n222 = Search 1D Array(1D array=w523, element=w522) -> (index of element=w520:i32)  [unwired: 1 in]
            n223 = global read "Global - Done.vi" "Done"() -> (w528:bool[])
            n224 = Replace Array Subset(array=w528, new element=w531, index=w520) -> (w526:bool[])
            n225 = global write "Global - Done.vi" "Done"(w526) -> ()
            n226 = case shown="True" w531 {
              tunnel: w527 -> [w539 w545]
              tunnel: [w540 w544] -> w534
              tunnel: w533 -> [_ w546]
              tunnel: w532 -> [_ w543]
              tunnel: w520 -> [_ w542]
              frame False {
                n227 = call "Communication - Trigger Read IP Address(FGV).vi"("Action"=eFGV_States."Write", "error in"=w539) -> ("error out"=w540:errorcluster)  [unwired: 7 in, 2 out]
              }
              frame True {
                n228 = case shown="\"Read Ch Data\"" w546 {
                  tunnel: w545 -> [w547 w554 w561 w567 w573 w579 w585]
                  tunnel: [w547 w554 w561 w567 w573 w579 w585] -> w544
                  tunnel: w543 -> [_ w552 w558 w566 w572 w578 w584]
                  tunnel: w542 -> [_ w556 w562 w568 w574 w580 w586]
                  frame "Stop", Default {
                  }
                  frame "Read Ch Data" {
                    n229 = Unbundle By Name(w552) -> ("Channels"=w551:T12, "Event"=w550:T10, "Status"=w549:T9)
                    n230 = global read "Global - Channel.vi" "Data"() -> (w555:T13)
                    n231 = Bundle("Channels"=w551, "Event"=w550, "Status"=w549) -> (w548:T14)  [unwired: 1 in]
                    n232 = Replace Array Subset(array=w555, new element=w548, index=w556) -> (w553:T13)
                    n233 = global write "Global - Channel.vi" "Data"(w553) -> ()
                  }
                  frame "Read Sensor" {
                    n234 = Unbundle By Name(w558) -> ("Sensor"=w557:T15)
                    n235 = global read "Global - Unit.vi" "Unit"() -> (w559:T16)
                    n236 = Replace Array Subset(array=w559, new element=w557, index=w562) -> (w560:T16)
                    n237 = global write "Global - Unit.vi" "Unit"(w560) -> ()
                  }
                  frame "Read ADC" {
                    n238 = Unbundle By Name(w566) -> ("ADC"=w563:T17)
                    n239 = global read "Global - ADC.vi" "ADC"() -> (w565:T18)
                    n240 = Replace Array Subset(array=w565, new element=w563, index=w568) -> (w564:T18)
                    n241 = global write "Global - ADC.vi" "ADC"(w564) -> ()
                  }
                  frame "Read PID" {
                    n242 = Unbundle By Name(w572) -> ("PID"=w569:T19)
                    n243 = global read "Global - PID.vi" "PID"() -> (w571:T20)
                    n244 = Replace Array Subset(array=w571, new element=w569, index=w574) -> (w570:T20)
                    n245 = global write "Global - PID.vi" "PID"(w570) -> ()
                  }
                  frame "Read System" {
                    n246 = Unbundle By Name(w578) -> ("System"=w576:T21)
                    n247 = global read "Global - System.vi" "System"() -> (w577:T22)
                    n248 = Replace Array Subset(array=w577, new element=w576, index=w580) -> (w575:T22)
                    n249 = global write "Global - System.vi" "System"(w575) -> ()
                  }
                  frame "Read Test" {
                    n250 = Unbundle By Name(w584) -> ("Test"=w581:T23)
                    n251 = global read "Global - Test.vi" "Test"() -> (w582:T24)
                    n252 = Replace Array Subset(array=w582, new element=w581, index=w586) -> (w583:T24)
                    n253 = global write "Global - Test.vi" "Test"(w583) -> ()
                  }
                }
              }
            }
          }
          frame "Close" {
          }
        }
      }
      frame Error {
        n254 = global read "Global - IP Address.vi" "IP"() -> (w599:string[])
        n255 = Unbundle By Name(w600) -> ("source"=w595:string)
        n256 = Index Array(array=w599, index=0) -> (element=w597:string)
        n257 = Concatenate Strings(w597, " - " ("string"), w595) -> (w591:string)
        n258 = call <vilib>:"Clear Errors.vi"("error in (no error)"=w600) -> ("error out"=w594:errorcluster)  [unwired: 5 in, 1 out]
        n259 = call "General - Error Log eFGV.vi"("eFGV States"=eFGV_States."Write", "error in (no error)"=w594, "Error In"=w591) -> ("error out"=w593:errorcluster)  [unwired: 6 in, 2 out]
        n260 = Wait (ms)(milliseconds to wait=u32 100) -> ()  [unwired: 1 out]
      }
    }
  }
  n261 = while {
    shift-right: [w609] -> _
    shift-left: errorcluster {"status"=FALSE, "code"=0, "source"=""} ("error IO") -> [w610]
    shift-right: [w607] -> _
    shift-left: Communications_-_State."Init" -> [w608]
    shift-right: [w605] -> _
    shift-left: _ -> [w604]
    stop <- w606 stop-if-true
    # "Command Processing Loop"
    n262 = case shown="No Error" w610 {
      selector: w610 -> [w616 w734]
      tunnel: [w617 w727] -> w609
      tunnel: w608 -> [w615 _]
      tunnel: [w614 Communications_-_State."Idle"] -> w607
      tunnel: [w613 _] -> w606
      tunnel: [w612 w736] -> w605
      tunnel: w604 -> [w611 w736]
      frame No Error {
        n263 = case shown="\"Idle\"" w615 {
          tunnel: [w620 w634 w668 w724] -> w617
          tunnel: w616 -> [w625 w633 w671 w724]
          tunnel: [Communications_-_State."Idle" w628 Communications_-_State."Idle" Communications_-_State."Close"] -> w614
          tunnel: [_ _ _ TRUE] -> w613
          tunnel: [w622 w632 w670 w721] -> w612
          tunnel: w611 -> [_ w631 w670 w721]
          frame "Init", Default {
            n264 = call "Communication - UDP Command (eFGV).vi"("Action"=eFGV_States."Read", "error in"=w625) -> ("error out"=w621:errorcluster, "UDP Ref"=w619:refnum<user-event>)  [unwired: 7 in, 1 out]
            n265 = register-events(error in=w621, w619) -> (reference out=w618:refnum<event-registration>, error out=w620:errorcluster)  [unwired: 1 in]
            n266 = Bundle By Name(cluster=T5 {"UDP CMD"={"IP"="", "CMD"=enum."Stop", "Port"="", "Datalog?"=FALSE, "Float"=0.0}, "UDP ref"=refnum, "Unit?"=FALSE, "Read Unit"=[], "Trig?"=FALSE, "UDP Info"=[], "UDP Conn ref"=refnum, "DataLogger"=[], "VISA Ref"=refnum, "Float"=0.0, "Data"={"Test"={"Target Load"=0.0, "Target Disp"=0.0, "Rate"=0.0, "Speed"=0.0}, "Sensor"={"Name"=[], "Unit"=[], "Decimal Point"=[], "Ch Log"=[], "H Alarm"=[], "L Alarm"=[], "H Limit"=[], "L Limit"=[], "Filter"=[], "Gain"=[], "Calib Type"=[]}, "PID"={"SP"=0.0, "PV"=0.0, "kP"=0.0, "kI"=0.0, "kD"=0.0, "FF"=0.0, "Err Band"=0.0, "Max"=0, "Min"=0, "Ts"=0, "Out"=0, "Mode"=0}, "ADC"={"Active Ch"=[], "Filter Type"=0, "Post Filter"=[], "Gain"=[], "FS"=0, "IntOC"=0, "IntFC"=0, "SysOC"=0, "Cofficient"=[], "K"=[], "Max"=0}, "System"={"Out Type"=0, "Inverse"=0, "Monitor"=0, "Reserve"=0, "ACC Time"=0, "Pulse Rev"=0, "Stroke"=0, "Auto Off"=0, "Gear Ratio"=0.0, "Pitch"=0.0, "Max Speed"=0, "Jog Speed"=0, "Disp Coff"=0.0, "Max Load"=0}, "Index"=enum."Ch1", "Datalog"=enum."Empty"}}, "UDP ref"=w618) -> (w622:T5)
          }
          frame "Idle" {
            n267 = Unbundle By Name(w631) -> ("UDP ref"=w635:refnum<event-registration>)
            n268 = event shown="[1] <FDTI ref>: User Event" {
              selector: w635 -> [_ _]
              dyn-events: _ -> [_ _]
              timeout: _ -> [_ _]
              tunnel: [w641 w643] -> w629
              tunnel: [w638 _] -> w634
              tunnel: w633 -> [w638 _]
              tunnel: [w636 w653] -> w632
              tunnel: w631 -> [w636 w652]
              event Timeout {
                n269 = event-data() -> ()  [unwired: 1 in, 1 out]
                n270 = local read "Stop"() -> (w640:bool)
                n271 = Select(t=Communications_-_State."Close", s=w640, f=Communications_-_State."Idle") -> (s? t:f=w641:T1)
              }
              event User Event {
                n272 = event-data() -> ("IP"=w646:string, "CMD"=w651:T3, "Data"=w650:T6)  [unwired: 1 in]
                n273 = global read "Global - IP Address.vi" "IP"() -> (w649:string[])
                n274 = Index Array(array=w649, index=12) -> (element=w647:string)
                n275 = Equal?(x=w647, y=w646) -> (x = y?=w645:bool)
                n276 = Bundle By Name(cluster=w652, "UDP CMD.IP"=w646, "UDP CMD.CMD"=w651, "Data"=w650) -> (w653:T5)
                n277 = Select(t=Communications_-_State."Command" ("f"), s=w645, f=Communications_-_State."Idle") -> (s? t:f=w643:T1)
              }
            }
            n278 = global read "Global - Hold.vi" "Hold"() -> (w630:bool)
            n279 = Select(t=Communications_-_State."Idle", s=w630, f=w629) -> (s? t:f=w628:T1)
          }
          frame "Command" {
            (unwired) UDP_-_Command."Stop" ("Enum")
            (unwired) 20
            n280 = Unbundle By Name(w670) -> ("UDP CMD.CMD"=w667:T3, "Data"=w669:T6, "UDP CMD.IP"=w664:string)
            n281 = global read "Global - Handle.vi" "Handle"() -> (w659:T7)
            n282 = global read "Global - IP Address.vi" "IP"() -> (w657:string[])
            n283 = Search 1D Array(1D array=w657, element=w664) -> (index of element=w655:i32)  [unwired: 1 in]
            n284 = Index Array(array=w659, index=w655) -> (element=w663:T8)
            n285 = call "UDP - Write CMD.vi"("CMD"=w667, "error in"=w671, "Data"=w669, "UDP Info"=w663) -> ("error out"=w661:errorcluster, "IP Address"=w656:string, "Data Out"=w666:T11, "Success"=w665:bool)  [unwired: 2 in, 2 out]
            n286 = Wait (ms)(milliseconds to wait=u32 5) -> ()  [unwired: 1 out]
            n287 = Search 1D Array(1D array=w657, element=w656) -> (index of element=w654:i32)  [unwired: 1 in]
            n288 = global read "Global - Done.vi" "Done"() -> (w662:bool[])
            n289 = Replace Array Subset(array=w662, new element=w665, index=w654) -> (w660:bool[])
            n290 = global write "Global - Done.vi" "Done"(w660) -> ()
            n291 = case shown="True" w665 {
              tunnel: w661 -> [w673 w679]
              tunnel: [w674 w678] -> w668
              tunnel: w667 -> [_ w680]
              tunnel: w666 -> [_ w677]
              tunnel: w654 -> [_ w676]
              frame False {
                n292 = call "Communication - Trigger Read IP Address(FGV).vi"("Action"=eFGV_States."Write", "error in"=w673) -> ("error out"=w674:errorcluster)  [unwired: 7 in, 2 out]
              }
              frame True {
                n293 = case shown="\"Read Ch Data\"" w680 {
                  tunnel: w679 -> [w681 w688 w695 w701 w707 w713 w719]
                  tunnel: [w681 w688 w695 w701 w707 w713 w719] -> w678
                  tunnel: w677 -> [_ w686 w692 w700 w706 w712 w718]
                  tunnel: w676 -> [_ w690 w696 w702 w708 w714 w720]
                  frame "Stop", Default {
                  }
                  frame "Read Ch Data" {
                    n294 = Unbundle By Name(w686) -> ("Channels"=w685:T12, "Event"=w684:T10, "Status"=w683:T9)
                    n295 = global read "Global - Channel.vi" "Data"() -> (w689:T13)
                    n296 = Bundle("Channels"=w685, "Event"=w684, "Status"=w683) -> (w682:T14)  [unwired: 1 in]
                    n297 = Replace Array Subset(array=w689, new element=w682, index=w690) -> (w687:T13)
                    n298 = global write "Global - Channel.vi" "Data"(w687) -> ()
                  }
                  frame "Read Sensor" {
                    n299 = Unbundle By Name(w692) -> ("Sensor"=w691:T15)
                    n300 = global read "Global - Unit.vi" "Unit"() -> (w693:T16)
                    n301 = Replace Array Subset(array=w693, new element=w691, index=w696) -> (w694:T16)
                    n302 = global write "Global - Unit.vi" "Unit"(w694) -> ()
                  }
                  frame "Read ADC" {
                    n303 = Unbundle By Name(w700) -> ("ADC"=w697:T17)
                    n304 = global read "Global - ADC.vi" "ADC"() -> (w699:T18)
                    n305 = Replace Array Subset(array=w699, new element=w697, index=w702) -> (w698:T18)
                    n306 = global write "Global - ADC.vi" "ADC"(w698) -> ()
                  }
                  frame "Read PID" {
                    n307 = Unbundle By Name(w706) -> ("PID"=w703:T19)
                    n308 = global read "Global - PID.vi" "PID"() -> (w705:T20)
                    n309 = Replace Array Subset(array=w705, new element=w703, index=w708) -> (w704:T20)
                    n310 = global write "Global - PID.vi" "PID"(w704) -> ()
                  }
                  frame "Read System" {
                    n311 = Unbundle By Name(w712) -> ("System"=w710:T21)
                    n312 = global read "Global - System.vi" "System"() -> (w711:T22)
                    n313 = Replace Array Subset(array=w711, new element=w710, index=w714) -> (w709:T22)
                    n314 = global write "Global - System.vi" "System"(w709) -> ()
                  }
                  frame "Read Test" {
                    n315 = Unbundle By Name(w718) -> ("Test"=w715:T23)
                    n316 = global read "Global - Test.vi" "Test"() -> (w716:T24)
                    n317 = Replace Array Subset(array=w716, new element=w715, index=w720) -> (w717:T24)
                    n318 = global write "Global - Test.vi" "Test"(w717) -> ()
                  }
                }
              }
            }
          }
          frame "Close" {
          }
        }
      }
      frame Error {
        n319 = global read "Global - IP Address.vi" "IP"() -> (w733:string[])
        n320 = Unbundle By Name(w734) -> ("source"=w729:string)
        n321 = Index Array(array=w733, index=0) -> (element=w731:string)
        n322 = Concatenate Strings(w731, " - " ("string"), w729) -> (w725:string)
        n323 = call <vilib>:"Clear Errors.vi"("error in (no error)"=w734) -> ("error out"=w728:errorcluster)  [unwired: 5 in, 1 out]
        n324 = call "General - Error Log eFGV.vi"("eFGV States"=eFGV_States."Write", "error in (no error)"=w728, "Error In"=w725) -> ("error out"=w727:errorcluster)  [unwired: 6 in, 2 out]
        n325 = Wait (ms)(milliseconds to wait=u32 100) -> ()  [unwired: 1 out]
      }
    }
  }
  n326 = while {
    shift-right: [w743] -> _
    shift-left: errorcluster {"status"=FALSE, "code"=0, "source"=""} ("error IO") -> [w744]
    shift-right: [w741] -> _
    shift-left: Communications_-_State."Init" -> [w742]
    shift-right: [w739] -> _
    shift-left: _ -> [w738]
    stop <- w740 stop-if-true
    # "Command Processing Loop"
    n327 = case shown="No Error" w744 {
      selector: w744 -> [w750 w868]
      tunnel: [w751 w861] -> w743
      tunnel: w742 -> [w749 _]
      tunnel: [w748 Communications_-_State."Idle"] -> w741
      tunnel: [w747 _] -> w740
      tunnel: [w746 w870] -> w739
      tunnel: w738 -> [w745 w870]
      frame No Error {
        n328 = case shown="\"Idle\"" w749 {
          tunnel: [w754 w768 w802 w858] -> w751
          tunnel: w750 -> [w759 w767 w805 w858]
          tunnel: [Communications_-_State."Idle" w762 Communications_-_State."Idle" Communications_-_State."Close"] -> w748
          tunnel: [_ _ _ TRUE] -> w747
          tunnel: [w756 w766 w804 w855] -> w746
          tunnel: w745 -> [_ w765 w804 w855]
          frame "Init", Default {
            n329 = call "Communication - UDP Command (eFGV).vi"("Action"=eFGV_States."Read", "error in"=w759) -> ("error out"=w755:errorcluster, "UDP Ref"=w753:refnum<user-event>)  [unwired: 7 in, 1 out]
            n330 = register-events(error in=w755, w753) -> (reference out=w752:refnum<event-registration>, error out=w754:errorcluster)  [unwired: 1 in]
            n331 = Bundle By Name(cluster=T5 {"UDP CMD"={"IP"="", "CMD"=enum."Stop", "Port"="", "Datalog?"=FALSE, "Float"=0.0}, "UDP ref"=refnum, "Unit?"=FALSE, "Read Unit"=[], "Trig?"=FALSE, "UDP Info"=[], "UDP Conn ref"=refnum, "DataLogger"=[], "VISA Ref"=refnum, "Float"=0.0, "Data"={"Test"={"Target Load"=0.0, "Target Disp"=0.0, "Rate"=0.0, "Speed"=0.0}, "Sensor"={"Name"=[], "Unit"=[], "Decimal Point"=[], "Ch Log"=[], "H Alarm"=[], "L Alarm"=[], "H Limit"=[], "L Limit"=[], "Filter"=[], "Gain"=[], "Calib Type"=[]}, "PID"={"SP"=0.0, "PV"=0.0, "kP"=0.0, "kI"=0.0, "kD"=0.0, "FF"=0.0, "Err Band"=0.0, "Max"=0, "Min"=0, "Ts"=0, "Out"=0, "Mode"=0}, "ADC"={"Active Ch"=[], "Filter Type"=0, "Post Filter"=[], "Gain"=[], "FS"=0, "IntOC"=0, "IntFC"=0, "SysOC"=0, "Cofficient"=[], "K"=[], "Max"=0}, "System"={"Out Type"=0, "Inverse"=0, "Monitor"=0, "Reserve"=0, "ACC Time"=0, "Pulse Rev"=0, "Stroke"=0, "Auto Off"=0, "Gear Ratio"=0.0, "Pitch"=0.0, "Max Speed"=0, "Jog Speed"=0, "Disp Coff"=0.0, "Max Load"=0}, "Index"=enum."Ch1", "Datalog"=enum."Empty"}}, "UDP ref"=w752) -> (w756:T5)
          }
          frame "Idle" {
            n332 = Unbundle By Name(w765) -> ("UDP ref"=w769:refnum<event-registration>)
            n333 = event shown="[1] <FDTI ref>: User Event" {
              selector: w769 -> [_ _]
              dyn-events: _ -> [_ _]
              timeout: _ -> [_ _]
              tunnel: [w775 w777] -> w763
              tunnel: [w772 _] -> w768
              tunnel: w767 -> [w772 _]
              tunnel: [w770 w787] -> w766
              tunnel: w765 -> [w770 w786]
              event Timeout {
                n334 = event-data() -> ()  [unwired: 1 in, 1 out]
                n335 = local read "Stop"() -> (w774:bool)
                n336 = Select(t=Communications_-_State."Close", s=w774, f=Communications_-_State."Idle") -> (s? t:f=w775:T1)
              }
              event User Event {
                n337 = event-data() -> ("IP"=w780:string, "CMD"=w785:T3, "Data"=w784:T6)  [unwired: 1 in]
                n338 = global read "Global - IP Address.vi" "IP"() -> (w783:string[])
                n339 = Index Array(array=w783, index=14) -> (element=w781:string)
                n340 = Equal?(x=w781, y=w780) -> (x = y?=w779:bool)
                n341 = Bundle By Name(cluster=w786, "UDP CMD.IP"=w780, "UDP CMD.CMD"=w785, "Data"=w784) -> (w787:T5)
                n342 = Select(t=Communications_-_State."Command" ("f"), s=w779, f=Communications_-_State."Idle") -> (s? t:f=w777:T1)
              }
            }
            n343 = global read "Global - Hold.vi" "Hold"() -> (w764:bool)
            n344 = Select(t=Communications_-_State."Idle", s=w764, f=w763) -> (s? t:f=w762:T1)
          }
          frame "Command" {
            (unwired) UDP_-_Command."Stop" ("Enum")
            (unwired) 20
            n345 = Unbundle By Name(w804) -> ("UDP CMD.CMD"=w801:T3, "Data"=w803:T6, "UDP CMD.IP"=w798:string)
            n346 = global read "Global - Handle.vi" "Handle"() -> (w793:T7)
            n347 = global read "Global - IP Address.vi" "IP"() -> (w791:string[])
            n348 = Search 1D Array(1D array=w791, element=w798) -> (index of element=w789:i32)  [unwired: 1 in]
            n349 = Index Array(array=w793, index=w789) -> (element=w797:T8)
            n350 = call "UDP - Write CMD.vi"("CMD"=w801, "error in"=w805, "Data"=w803, "UDP Info"=w797) -> ("error out"=w795:errorcluster, "IP Address"=w790:string, "Data Out"=w800:T11, "Success"=w799:bool)  [unwired: 2 in, 2 out]
            n351 = Wait (ms)(milliseconds to wait=u32 5) -> ()  [unwired: 1 out]
            n352 = Search 1D Array(1D array=w791, element=w790) -> (index of element=w788:i32)  [unwired: 1 in]
            n353 = global read "Global - Done.vi" "Done"() -> (w796:bool[])
            n354 = Replace Array Subset(array=w796, new element=w799, index=w788) -> (w794:bool[])
            n355 = global write "Global - Done.vi" "Done"(w794) -> ()
            n356 = case shown="True" w799 {
              tunnel: w795 -> [w807 w813]
              tunnel: [w808 w812] -> w802
              tunnel: w801 -> [_ w814]
              tunnel: w800 -> [_ w811]
              tunnel: w788 -> [_ w810]
              frame False {
                n357 = call "Communication - Trigger Read IP Address(FGV).vi"("Action"=eFGV_States."Write", "error in"=w807) -> ("error out"=w808:errorcluster)  [unwired: 7 in, 2 out]
              }
              frame True {
                n358 = case shown="\"Read Ch Data\"" w814 {
                  tunnel: w813 -> [w815 w822 w829 w835 w841 w847 w853]
                  tunnel: [w815 w822 w829 w835 w841 w847 w853] -> w812
                  tunnel: w811 -> [_ w820 w826 w834 w840 w846 w852]
                  tunnel: w810 -> [_ w824 w830 w836 w842 w848 w854]
                  frame "Stop", Default {
                  }
                  frame "Read Ch Data" {
                    n359 = Unbundle By Name(w820) -> ("Channels"=w819:T12, "Event"=w818:T10, "Status"=w817:T9)
                    n360 = global read "Global - Channel.vi" "Data"() -> (w823:T13)
                    n361 = Bundle("Channels"=w819, "Event"=w818, "Status"=w817) -> (w816:T14)  [unwired: 1 in]
                    n362 = Replace Array Subset(array=w823, new element=w816, index=w824) -> (w821:T13)
                    n363 = global write "Global - Channel.vi" "Data"(w821) -> ()
                  }
                  frame "Read Sensor" {
                    n364 = Unbundle By Name(w826) -> ("Sensor"=w825:T15)
                    n365 = global read "Global - Unit.vi" "Unit"() -> (w827:T16)
                    n366 = Replace Array Subset(array=w827, new element=w825, index=w830) -> (w828:T16)
                    n367 = global write "Global - Unit.vi" "Unit"(w828) -> ()
                  }
                  frame "Read ADC" {
                    n368 = Unbundle By Name(w834) -> ("ADC"=w831:T17)
                    n369 = global read "Global - ADC.vi" "ADC"() -> (w833:T18)
                    n370 = Replace Array Subset(array=w833, new element=w831, index=w836) -> (w832:T18)
                    n371 = global write "Global - ADC.vi" "ADC"(w832) -> ()
                  }
                  frame "Read PID" {
                    n372 = Unbundle By Name(w840) -> ("PID"=w837:T19)
                    n373 = global read "Global - PID.vi" "PID"() -> (w839:T20)
                    n374 = Replace Array Subset(array=w839, new element=w837, index=w842) -> (w838:T20)
                    n375 = global write "Global - PID.vi" "PID"(w838) -> ()
                  }
                  frame "Read System" {
                    n376 = Unbundle By Name(w846) -> ("System"=w844:T21)
                    n377 = global read "Global - System.vi" "System"() -> (w845:T22)
                    n378 = Replace Array Subset(array=w845, new element=w844, index=w848) -> (w843:T22)
                    n379 = global write "Global - System.vi" "System"(w843) -> ()
                  }
                  frame "Read Test" {
                    n380 = Unbundle By Name(w852) -> ("Test"=w849:T23)
                    n381 = global read "Global - Test.vi" "Test"() -> (w850:T24)
                    n382 = Replace Array Subset(array=w850, new element=w849, index=w854) -> (w851:T24)
                    n383 = global write "Global - Test.vi" "Test"(w851) -> ()
                  }
                }
              }
            }
          }
          frame "Close" {
          }
        }
      }
      frame Error {
        n384 = global read "Global - IP Address.vi" "IP"() -> (w867:string[])
        n385 = Unbundle By Name(w868) -> ("source"=w863:string)
        n386 = Index Array(array=w867, index=0) -> (element=w865:string)
        n387 = Concatenate Strings(w865, " - " ("string"), w863) -> (w859:string)
        n388 = call <vilib>:"Clear Errors.vi"("error in (no error)"=w868) -> ("error out"=w862:errorcluster)  [unwired: 5 in, 1 out]
        n389 = call "General - Error Log eFGV.vi"("eFGV States"=eFGV_States."Write", "error in (no error)"=w862, "Error In"=w859) -> ("error out"=w861:errorcluster)  [unwired: 6 in, 2 out]
        n390 = Wait (ms)(milliseconds to wait=u32 100) -> ()  [unwired: 1 out]
      }
    }
  }
  n391 = while {
    shift-right: [w877] -> _
    shift-left: errorcluster {"status"=FALSE, "code"=0, "source"=""} ("error IO") -> [w878]
    shift-right: [w875] -> _
    shift-left: Communications_-_State."Init" -> [w876]
    shift-right: [w873] -> _
    shift-left: _ -> [w872]
    stop <- w874 stop-if-true
    # "Command Processing Loop"
    n392 = case shown="No Error" w878 {
      selector: w878 -> [w884 w1002]
      tunnel: [w885 w995] -> w877
      tunnel: w876 -> [w883 _]
      tunnel: [w882 Communications_-_State."Idle"] -> w875
      tunnel: [w881 _] -> w874
      tunnel: [w880 w1004] -> w873
      tunnel: w872 -> [w879 w1004]
      frame No Error {
        n393 = case shown="\"Idle\"" w883 {
          tunnel: [w888 w902 w936 w992] -> w885
          tunnel: w884 -> [w893 w901 w939 w992]
          tunnel: [Communications_-_State."Idle" w896 Communications_-_State."Idle" Communications_-_State."Close"] -> w882
          tunnel: [_ _ _ TRUE] -> w881
          tunnel: [w890 w900 w938 w989] -> w880
          tunnel: w879 -> [_ w899 w938 w989]
          frame "Init", Default {
            n394 = call "Communication - UDP Command (eFGV).vi"("Action"=eFGV_States."Read", "error in"=w893) -> ("error out"=w889:errorcluster, "UDP Ref"=w887:refnum<user-event>)  [unwired: 7 in, 1 out]
            n395 = register-events(error in=w889, w887) -> (reference out=w886:refnum<event-registration>, error out=w888:errorcluster)  [unwired: 1 in]
            n396 = Bundle By Name(cluster=T5 {"UDP CMD"={"IP"="", "CMD"=enum."Stop", "Port"="", "Datalog?"=FALSE, "Float"=0.0}, "UDP ref"=refnum, "Unit?"=FALSE, "Read Unit"=[], "Trig?"=FALSE, "UDP Info"=[], "UDP Conn ref"=refnum, "DataLogger"=[], "VISA Ref"=refnum, "Float"=0.0, "Data"={"Test"={"Target Load"=0.0, "Target Disp"=0.0, "Rate"=0.0, "Speed"=0.0}, "Sensor"={"Name"=[], "Unit"=[], "Decimal Point"=[], "Ch Log"=[], "H Alarm"=[], "L Alarm"=[], "H Limit"=[], "L Limit"=[], "Filter"=[], "Gain"=[], "Calib Type"=[]}, "PID"={"SP"=0.0, "PV"=0.0, "kP"=0.0, "kI"=0.0, "kD"=0.0, "FF"=0.0, "Err Band"=0.0, "Max"=0, "Min"=0, "Ts"=0, "Out"=0, "Mode"=0}, "ADC"={"Active Ch"=[], "Filter Type"=0, "Post Filter"=[], "Gain"=[], "FS"=0, "IntOC"=0, "IntFC"=0, "SysOC"=0, "Cofficient"=[], "K"=[], "Max"=0}, "System"={"Out Type"=0, "Inverse"=0, "Monitor"=0, "Reserve"=0, "ACC Time"=0, "Pulse Rev"=0, "Stroke"=0, "Auto Off"=0, "Gear Ratio"=0.0, "Pitch"=0.0, "Max Speed"=0, "Jog Speed"=0, "Disp Coff"=0.0, "Max Load"=0}, "Index"=enum."Ch1", "Datalog"=enum."Empty"}}, "UDP ref"=w886) -> (w890:T5)
          }
          frame "Idle" {
            n397 = Unbundle By Name(w899) -> ("UDP ref"=w903:refnum<event-registration>)
            n398 = event shown="[1] <FDTI ref>: User Event" {
              selector: w903 -> [_ _]
              dyn-events: _ -> [_ _]
              timeout: _ -> [_ _]
              tunnel: [w909 w911] -> w897
              tunnel: [w906 _] -> w902
              tunnel: w901 -> [w906 _]
              tunnel: [w904 w921] -> w900
              tunnel: w899 -> [w904 w920]
              event Timeout {
                n399 = event-data() -> ()  [unwired: 1 in, 1 out]
                n400 = local read "Stop"() -> (w908:bool)
                n401 = Select(t=Communications_-_State."Close", s=w908, f=Communications_-_State."Idle") -> (s? t:f=w909:T1)
              }
              event User Event {
                n402 = event-data() -> ("IP"=w914:string, "CMD"=w919:T3, "Data"=w918:T6)  [unwired: 1 in]
                n403 = global read "Global - IP Address.vi" "IP"() -> (w917:string[])
                n404 = Index Array(array=w917, index=20) -> (element=w915:string)
                n405 = Equal?(x=w915, y=w914) -> (x = y?=w913:bool)
                n406 = Bundle By Name(cluster=w920, "UDP CMD.IP"=w914, "UDP CMD.CMD"=w919, "Data"=w918) -> (w921:T5)
                n407 = Select(t=Communications_-_State."Command" ("f"), s=w913, f=Communications_-_State."Idle") -> (s? t:f=w911:T1)
              }
            }
            n408 = global read "Global - Hold.vi" "Hold"() -> (w898:bool)
            n409 = Select(t=Communications_-_State."Idle", s=w898, f=w897) -> (s? t:f=w896:T1)
          }
          frame "Command" {
            (unwired) UDP_-_Command."Stop" ("Enum")
            (unwired) 20
            n410 = Unbundle By Name(w938) -> ("UDP CMD.CMD"=w935:T3, "Data"=w937:T6, "UDP CMD.IP"=w932:string)
            n411 = global read "Global - Handle.vi" "Handle"() -> (w927:T7)
            n412 = global read "Global - IP Address.vi" "IP"() -> (w925:string[])
            n413 = Search 1D Array(1D array=w925, element=w932) -> (index of element=w923:i32)  [unwired: 1 in]
            n414 = Index Array(array=w927, index=w923) -> (element=w931:T8)
            n415 = call "UDP - Write CMD.vi"("CMD"=w935, "error in"=w939, "Data"=w937, "UDP Info"=w931) -> ("error out"=w929:errorcluster, "IP Address"=w924:string, "Data Out"=w934:T11, "Success"=w933:bool)  [unwired: 2 in, 2 out]
            n416 = Wait (ms)(milliseconds to wait=u32 5) -> ()  [unwired: 1 out]
            n417 = Search 1D Array(1D array=w925, element=w924) -> (index of element=w922:i32)  [unwired: 1 in]
            n418 = global read "Global - Done.vi" "Done"() -> (w930:bool[])
            n419 = Replace Array Subset(array=w930, new element=w933, index=w922) -> (w928:bool[])
            n420 = global write "Global - Done.vi" "Done"(w928) -> ()
            n421 = case shown="True" w933 {
              tunnel: w929 -> [w941 w947]
              tunnel: [w942 w946] -> w936
              tunnel: w935 -> [_ w948]
              tunnel: w934 -> [_ w945]
              tunnel: w922 -> [_ w944]
              frame False {
                n422 = call "Communication - Trigger Read IP Address(FGV).vi"("Action"=eFGV_States."Write", "error in"=w941) -> ("error out"=w942:errorcluster)  [unwired: 7 in, 2 out]
              }
              frame True {
                n423 = case shown="\"Read Ch Data\"" w948 {
                  tunnel: w947 -> [w949 w956 w963 w969 w975 w981 w987]
                  tunnel: [w949 w956 w963 w969 w975 w981 w987] -> w946
                  tunnel: w945 -> [_ w954 w960 w968 w974 w980 w986]
                  tunnel: w944 -> [_ w958 w964 w970 w976 w982 w988]
                  frame "Stop", Default {
                  }
                  frame "Read Ch Data" {
                    n424 = Unbundle By Name(w954) -> ("Channels"=w953:T12, "Event"=w952:T10, "Status"=w951:T9)
                    n425 = global read "Global - Channel.vi" "Data"() -> (w957:T13)
                    n426 = Bundle("Channels"=w953, "Event"=w952, "Status"=w951) -> (w950:T14)  [unwired: 1 in]
                    n427 = Replace Array Subset(array=w957, new element=w950, index=w958) -> (w955:T13)
                    n428 = global write "Global - Channel.vi" "Data"(w955) -> ()
                  }
                  frame "Read Sensor" {
                    n429 = Unbundle By Name(w960) -> ("Sensor"=w959:T15)
                    n430 = global read "Global - Unit.vi" "Unit"() -> (w961:T16)
                    n431 = Replace Array Subset(array=w961, new element=w959, index=w964) -> (w962:T16)
                    n432 = global write "Global - Unit.vi" "Unit"(w962) -> ()
                  }
                  frame "Read ADC" {
                    n433 = Unbundle By Name(w968) -> ("ADC"=w965:T17)
                    n434 = global read "Global - ADC.vi" "ADC"() -> (w967:T18)
                    n435 = Replace Array Subset(array=w967, new element=w965, index=w970) -> (w966:T18)
                    n436 = global write "Global - ADC.vi" "ADC"(w966) -> ()
                  }
                  frame "Read PID" {
                    n437 = Unbundle By Name(w974) -> ("PID"=w971:T19)
                    n438 = global read "Global - PID.vi" "PID"() -> (w973:T20)
                    n439 = Replace Array Subset(array=w973, new element=w971, index=w976) -> (w972:T20)
                    n440 = global write "Global - PID.vi" "PID"(w972) -> ()
                  }
                  frame "Read System" {
                    n441 = Unbundle By Name(w980) -> ("System"=w978:T21)
                    n442 = global read "Global - System.vi" "System"() -> (w979:T22)
                    n443 = Replace Array Subset(array=w979, new element=w978, index=w982) -> (w977:T22)
                    n444 = global write "Global - System.vi" "System"(w977) -> ()
                  }
                  frame "Read Test" {
                    n445 = Unbundle By Name(w986) -> ("Test"=w983:T23)
                    n446 = global read "Global - Test.vi" "Test"() -> (w984:T24)
                    n447 = Replace Array Subset(array=w984, new element=w983, index=w988) -> (w985:T24)
                    n448 = global write "Global - Test.vi" "Test"(w985) -> ()
                  }
                }
              }
            }
          }
          frame "Close" {
          }
        }
      }
      frame Error {
        n449 = global read "Global - IP Address.vi" "IP"() -> (w1001:string[])
        n450 = Unbundle By Name(w1002) -> ("source"=w997:string)
        n451 = Index Array(array=w1001, index=0) -> (element=w999:string)
        n452 = Concatenate Strings(w999, " - " ("string"), w997) -> (w993:string)
        n453 = call <vilib>:"Clear Errors.vi"("error in (no error)"=w1002) -> ("error out"=w996:errorcluster)  [unwired: 5 in, 1 out]
        n454 = call "General - Error Log eFGV.vi"("eFGV States"=eFGV_States."Write", "error in (no error)"=w996, "Error In"=w993) -> ("error out"=w995:errorcluster)  [unwired: 6 in, 2 out]
        n455 = Wait (ms)(milliseconds to wait=u32 100) -> ()  [unwired: 1 out]
      }
    }
  }
  n456 = while {
    shift-right: [w1011] -> _
    shift-left: errorcluster {"status"=FALSE, "code"=0, "source"=""} ("error IO") -> [w1012]
    shift-right: [w1009] -> _
    shift-left: Communications_-_State."Init" -> [w1010]
    shift-right: [w1007] -> _
    shift-left: _ -> [w1006]
    stop <- w1008 stop-if-true
    # "Command Processing Loop"
    n457 = case shown="No Error" w1012 {
      selector: w1012 -> [w1018 w1136]
      tunnel: [w1019 w1129] -> w1011
      tunnel: w1010 -> [w1017 _]
      tunnel: [w1016 Communications_-_State."Idle"] -> w1009
      tunnel: [w1015 _] -> w1008
      tunnel: [w1014 w1138] -> w1007
      tunnel: w1006 -> [w1013 w1138]
      frame No Error {
        n458 = case shown="\"Idle\"" w1017 {
          tunnel: [w1022 w1036 w1070 w1126] -> w1019
          tunnel: w1018 -> [w1027 w1035 w1073 w1126]
          tunnel: [Communications_-_State."Idle" w1030 Communications_-_State."Idle" Communications_-_State."Close"] -> w1016
          tunnel: [_ _ _ TRUE] -> w1015
          tunnel: [w1024 w1034 w1072 w1123] -> w1014
          tunnel: w1013 -> [_ w1033 w1072 w1123]
          frame "Init", Default {
            n459 = call "Communication - UDP Command (eFGV).vi"("Action"=eFGV_States."Read", "error in"=w1027) -> ("error out"=w1023:errorcluster, "UDP Ref"=w1021:refnum<user-event>)  [unwired: 7 in, 1 out]
            n460 = register-events(error in=w1023, w1021) -> (reference out=w1020:refnum<event-registration>, error out=w1022:errorcluster)  [unwired: 1 in]
            n461 = Bundle By Name(cluster=T5 {"UDP CMD"={"IP"="", "CMD"=enum."Stop", "Port"="", "Datalog?"=FALSE, "Float"=0.0}, "UDP ref"=refnum, "Unit?"=FALSE, "Read Unit"=[], "Trig?"=FALSE, "UDP Info"=[], "UDP Conn ref"=refnum, "DataLogger"=[], "VISA Ref"=refnum, "Float"=0.0, "Data"={"Test"={"Target Load"=0.0, "Target Disp"=0.0, "Rate"=0.0, "Speed"=0.0}, "Sensor"={"Name"=[], "Unit"=[], "Decimal Point"=[], "Ch Log"=[], "H Alarm"=[], "L Alarm"=[], "H Limit"=[], "L Limit"=[], "Filter"=[], "Gain"=[], "Calib Type"=[]}, "PID"={"SP"=0.0, "PV"=0.0, "kP"=0.0, "kI"=0.0, "kD"=0.0, "FF"=0.0, "Err Band"=0.0, "Max"=0, "Min"=0, "Ts"=0, "Out"=0, "Mode"=0}, "ADC"={"Active Ch"=[], "Filter Type"=0, "Post Filter"=[], "Gain"=[], "FS"=0, "IntOC"=0, "IntFC"=0, "SysOC"=0, "Cofficient"=[], "K"=[], "Max"=0}, "System"={"Out Type"=0, "Inverse"=0, "Monitor"=0, "Reserve"=0, "ACC Time"=0, "Pulse Rev"=0, "Stroke"=0, "Auto Off"=0, "Gear Ratio"=0.0, "Pitch"=0.0, "Max Speed"=0, "Jog Speed"=0, "Disp Coff"=0.0, "Max Load"=0}, "Index"=enum."Ch1", "Datalog"=enum."Empty"}}, "UDP ref"=w1020) -> (w1024:T5)
          }
          frame "Idle" {
            n462 = Unbundle By Name(w1033) -> ("UDP ref"=w1037:refnum<event-registration>)
            n463 = event shown="[1] <FDTI ref>: User Event" {
              selector: w1037 -> [_ _]
              dyn-events: _ -> [_ _]
              timeout: _ -> [_ _]
              tunnel: [w1043 w1045] -> w1031
              tunnel: [w1040 _] -> w1036
              tunnel: w1035 -> [w1040 _]
              tunnel: [w1038 w1055] -> w1034
              tunnel: w1033 -> [w1038 w1054]
              event Timeout {
                n464 = event-data() -> ()  [unwired: 1 in, 1 out]
                n465 = local read "Stop"() -> (w1042:bool)
                n466 = Select(t=Communications_-_State."Close", s=w1042, f=Communications_-_State."Idle") -> (s? t:f=w1043:T1)
              }
              event User Event {
                n467 = event-data() -> ("IP"=w1048:string, "CMD"=w1053:T3, "Data"=w1052:T6)  [unwired: 1 in]
                n468 = global read "Global - IP Address.vi" "IP"() -> (w1051:string[])
                n469 = Index Array(array=w1051, index=22) -> (element=w1049:string)
                n470 = Equal?(x=w1049, y=w1048) -> (x = y?=w1047:bool)
                n471 = Bundle By Name(cluster=w1054, "UDP CMD.IP"=w1048, "UDP CMD.CMD"=w1053, "Data"=w1052) -> (w1055:T5)
                n472 = Select(t=Communications_-_State."Command" ("f"), s=w1047, f=Communications_-_State."Idle") -> (s? t:f=w1045:T1)
              }
            }
            n473 = global read "Global - Hold.vi" "Hold"() -> (w1032:bool)
            n474 = Select(t=Communications_-_State."Idle", s=w1032, f=w1031) -> (s? t:f=w1030:T1)
          }
          frame "Command" {
            (unwired) UDP_-_Command."Stop" ("Enum")
            (unwired) 20
            n475 = Unbundle By Name(w1072) -> ("UDP CMD.CMD"=w1069:T3, "Data"=w1071:T6, "UDP CMD.IP"=w1066:string)
            n476 = global read "Global - Handle.vi" "Handle"() -> (w1061:T7)
            n477 = global read "Global - IP Address.vi" "IP"() -> (w1059:string[])
            n478 = Search 1D Array(1D array=w1059, element=w1066) -> (index of element=w1057:i32)  [unwired: 1 in]
            n479 = Index Array(array=w1061, index=w1057) -> (element=w1065:T8)
            n480 = call "UDP - Write CMD.vi"("CMD"=w1069, "error in"=w1073, "Data"=w1071, "UDP Info"=w1065) -> ("error out"=w1063:errorcluster, "IP Address"=w1058:string, "Data Out"=w1068:T11, "Success"=w1067:bool)  [unwired: 2 in, 2 out]
            n481 = Wait (ms)(milliseconds to wait=u32 5) -> ()  [unwired: 1 out]
            n482 = Search 1D Array(1D array=w1059, element=w1058) -> (index of element=w1056:i32)  [unwired: 1 in]
            n483 = global read "Global - Done.vi" "Done"() -> (w1064:bool[])
            n484 = Replace Array Subset(array=w1064, new element=w1067, index=w1056) -> (w1062:bool[])
            n485 = global write "Global - Done.vi" "Done"(w1062) -> ()
            n486 = case shown="True" w1067 {
              tunnel: w1063 -> [w1075 w1081]
              tunnel: [w1076 w1080] -> w1070
              tunnel: w1069 -> [_ w1082]
              tunnel: w1068 -> [_ w1079]
              tunnel: w1056 -> [_ w1078]
              frame False {
                n487 = call "Communication - Trigger Read IP Address(FGV).vi"("Action"=eFGV_States."Write", "error in"=w1075) -> ("error out"=w1076:errorcluster)  [unwired: 7 in, 2 out]
              }
              frame True {
                n488 = case shown="\"Read Ch Data\"" w1082 {
                  tunnel: w1081 -> [w1083 w1090 w1097 w1103 w1109 w1115 w1121]
                  tunnel: [w1083 w1090 w1097 w1103 w1109 w1115 w1121] -> w1080
                  tunnel: w1079 -> [_ w1088 w1094 w1102 w1108 w1114 w1120]
                  tunnel: w1078 -> [_ w1092 w1098 w1104 w1110 w1116 w1122]
                  frame "Stop", Default {
                  }
                  frame "Read Ch Data" {
                    n489 = Unbundle By Name(w1088) -> ("Channels"=w1087:T12, "Event"=w1086:T10, "Status"=w1085:T9)
                    n490 = global read "Global - Channel.vi" "Data"() -> (w1091:T13)
                    n491 = Bundle("Channels"=w1087, "Event"=w1086, "Status"=w1085) -> (w1084:T14)  [unwired: 1 in]
                    n492 = Replace Array Subset(array=w1091, new element=w1084, index=w1092) -> (w1089:T13)
                    n493 = global write "Global - Channel.vi" "Data"(w1089) -> ()
                  }
                  frame "Read Sensor" {
                    n494 = Unbundle By Name(w1094) -> ("Sensor"=w1093:T15)
                    n495 = global read "Global - Unit.vi" "Unit"() -> (w1095:T16)
                    n496 = Replace Array Subset(array=w1095, new element=w1093, index=w1098) -> (w1096:T16)
                    n497 = global write "Global - Unit.vi" "Unit"(w1096) -> ()
                  }
                  frame "Read ADC" {
                    n498 = Unbundle By Name(w1102) -> ("ADC"=w1099:T17)
                    n499 = global read "Global - ADC.vi" "ADC"() -> (w1101:T18)
                    n500 = Replace Array Subset(array=w1101, new element=w1099, index=w1104) -> (w1100:T18)
                    n501 = global write "Global - ADC.vi" "ADC"(w1100) -> ()
                  }
                  frame "Read PID" {
                    n502 = Unbundle By Name(w1108) -> ("PID"=w1105:T19)
                    n503 = global read "Global - PID.vi" "PID"() -> (w1107:T20)
                    n504 = Replace Array Subset(array=w1107, new element=w1105, index=w1110) -> (w1106:T20)
                    n505 = global write "Global - PID.vi" "PID"(w1106) -> ()
                  }
                  frame "Read System" {
                    n506 = Unbundle By Name(w1114) -> ("System"=w1112:T21)
                    n507 = global read "Global - System.vi" "System"() -> (w1113:T22)
                    n508 = Replace Array Subset(array=w1113, new element=w1112, index=w1116) -> (w1111:T22)
                    n509 = global write "Global - System.vi" "System"(w1111) -> ()
                  }
                  frame "Read Test" {
                    n510 = Unbundle By Name(w1120) -> ("Test"=w1117:T23)
                    n511 = global read "Global - Test.vi" "Test"() -> (w1118:T24)
                    n512 = Replace Array Subset(array=w1118, new element=w1117, index=w1122) -> (w1119:T24)
                    n513 = global write "Global - Test.vi" "Test"(w1119) -> ()
                  }
                }
              }
            }
          }
          frame "Close" {
          }
        }
      }
      frame Error {
        n514 = global read "Global - IP Address.vi" "IP"() -> (w1135:string[])
        n515 = Unbundle By Name(w1136) -> ("source"=w1131:string)
        n516 = Index Array(array=w1135, index=0) -> (element=w1133:string)
        n517 = Concatenate Strings(w1133, " - " ("string"), w1131) -> (w1127:string)
        n518 = call <vilib>:"Clear Errors.vi"("error in (no error)"=w1136) -> ("error out"=w1130:errorcluster)  [unwired: 5 in, 1 out]
        n519 = call "General - Error Log eFGV.vi"("eFGV States"=eFGV_States."Write", "error in (no error)"=w1130, "Error In"=w1127) -> ("error out"=w1129:errorcluster)  [unwired: 6 in, 2 out]
        n520 = Wait (ms)(milliseconds to wait=u32 100) -> ()  [unwired: 1 out]
      }
    }
  }
  n521 = while {
    shift-right: [w1145] -> _
    shift-left: errorcluster {"status"=FALSE, "code"=0, "source"=""} ("error IO") -> [w1146]
    shift-right: [w1143] -> _
    shift-left: Communications_-_State."Init" -> [w1144]
    shift-right: [w1141] -> _
    shift-left: _ -> [w1140]
    stop <- w1142 stop-if-true
    # "Command Processing Loop"
    n522 = case shown="No Error" w1146 {
      selector: w1146 -> [w1152 w1270]
      tunnel: [w1153 w1263] -> w1145
      tunnel: w1144 -> [w1151 _]
      tunnel: [w1150 Communications_-_State."Idle"] -> w1143
      tunnel: [w1149 _] -> w1142
      tunnel: [w1148 w1272] -> w1141
      tunnel: w1140 -> [w1147 w1272]
      frame No Error {
        n523 = case shown="\"Idle\"" w1151 {
          tunnel: [w1156 w1170 w1204 w1260] -> w1153
          tunnel: w1152 -> [w1161 w1169 w1207 w1260]
          tunnel: [Communications_-_State."Idle" w1164 Communications_-_State."Idle" Communications_-_State."Close"] -> w1150
          tunnel: [_ _ _ TRUE] -> w1149
          tunnel: [w1158 w1168 w1206 w1257] -> w1148
          tunnel: w1147 -> [_ w1167 w1206 w1257]
          frame "Init", Default {
            n524 = call "Communication - UDP Command (eFGV).vi"("Action"=eFGV_States."Read", "error in"=w1161) -> ("error out"=w1157:errorcluster, "UDP Ref"=w1155:refnum<user-event>)  [unwired: 7 in, 1 out]
            n525 = register-events(error in=w1157, w1155) -> (reference out=w1154:refnum<event-registration>, error out=w1156:errorcluster)  [unwired: 1 in]
            n526 = Bundle By Name(cluster=T5 {"UDP CMD"={"IP"="", "CMD"=enum."Stop", "Port"="", "Datalog?"=FALSE, "Float"=0.0}, "UDP ref"=refnum, "Unit?"=FALSE, "Read Unit"=[], "Trig?"=FALSE, "UDP Info"=[], "UDP Conn ref"=refnum, "DataLogger"=[], "VISA Ref"=refnum, "Float"=0.0, "Data"={"Test"={"Target Load"=0.0, "Target Disp"=0.0, "Rate"=0.0, "Speed"=0.0}, "Sensor"={"Name"=[], "Unit"=[], "Decimal Point"=[], "Ch Log"=[], "H Alarm"=[], "L Alarm"=[], "H Limit"=[], "L Limit"=[], "Filter"=[], "Gain"=[], "Calib Type"=[]}, "PID"={"SP"=0.0, "PV"=0.0, "kP"=0.0, "kI"=0.0, "kD"=0.0, "FF"=0.0, "Err Band"=0.0, "Max"=0, "Min"=0, "Ts"=0, "Out"=0, "Mode"=0}, "ADC"={"Active Ch"=[], "Filter Type"=0, "Post Filter"=[], "Gain"=[], "FS"=0, "IntOC"=0, "IntFC"=0, "SysOC"=0, "Cofficient"=[], "K"=[], "Max"=0}, "System"={"Out Type"=0, "Inverse"=0, "Monitor"=0, "Reserve"=0, "ACC Time"=0, "Pulse Rev"=0, "Stroke"=0, "Auto Off"=0, "Gear Ratio"=0.0, "Pitch"=0.0, "Max Speed"=0, "Jog Speed"=0, "Disp Coff"=0.0, "Max Load"=0}, "Index"=enum."Ch1", "Datalog"=enum."Empty"}}, "UDP ref"=w1154) -> (w1158:T5)
          }
          frame "Idle" {
            n527 = Unbundle By Name(w1167) -> ("UDP ref"=w1171:refnum<event-registration>)
            n528 = event shown="[1] <FDTI ref>: User Event" {
              selector: w1171 -> [_ _]
              dyn-events: _ -> [_ _]
              timeout: _ -> [_ _]
              tunnel: [w1177 w1179] -> w1165
              tunnel: [w1174 _] -> w1170
              tunnel: w1169 -> [w1174 _]
              tunnel: [w1172 w1189] -> w1168
              tunnel: w1167 -> [w1172 w1188]
              event Timeout {
                n529 = event-data() -> ()  [unwired: 1 in, 1 out]
                n530 = local read "Stop"() -> (w1176:bool)
                n531 = Select(t=Communications_-_State."Close", s=w1176, f=Communications_-_State."Idle") -> (s? t:f=w1177:T1)
              }
              event User Event {
                n532 = event-data() -> ("IP"=w1182:string, "CMD"=w1187:T3, "Data"=w1186:T6)  [unwired: 1 in]
                n533 = global read "Global - IP Address.vi" "IP"() -> (w1185:string[])
                n534 = Index Array(array=w1185, index=8) -> (element=w1183:string)
                n535 = Equal?(x=w1183, y=w1182) -> (x = y?=w1181:bool)
                n536 = Bundle By Name(cluster=w1188, "UDP CMD.IP"=w1182, "UDP CMD.CMD"=w1187, "Data"=w1186) -> (w1189:T5)
                n537 = Select(t=Communications_-_State."Command" ("f"), s=w1181, f=Communications_-_State."Idle") -> (s? t:f=w1179:T1)
              }
            }
            n538 = global read "Global - Hold.vi" "Hold"() -> (w1166:bool)
            n539 = Select(t=Communications_-_State."Idle", s=w1166, f=w1165) -> (s? t:f=w1164:T1)
          }
          frame "Command" {
            (unwired) UDP_-_Command."Stop" ("Enum")
            (unwired) 20
            n540 = Unbundle By Name(w1206) -> ("UDP CMD.CMD"=w1203:T3, "Data"=w1205:T6, "UDP CMD.IP"=w1200:string)
            n541 = global read "Global - Handle.vi" "Handle"() -> (w1195:T7)
            n542 = global read "Global - IP Address.vi" "IP"() -> (w1193:string[])
            n543 = Search 1D Array(1D array=w1193, element=w1200) -> (index of element=w1191:i32)  [unwired: 1 in]
            n544 = Index Array(array=w1195, index=w1191) -> (element=w1199:T8)
            n545 = call "UDP - Write CMD.vi"("CMD"=w1203, "error in"=w1207, "Data"=w1205, "UDP Info"=w1199) -> ("error out"=w1197:errorcluster, "IP Address"=w1192:string, "Data Out"=w1202:T11, "Success"=w1201:bool)  [unwired: 2 in, 2 out]
            n546 = Wait (ms)(milliseconds to wait=u32 5) -> ()  [unwired: 1 out]
            n547 = Search 1D Array(1D array=w1193, element=w1192) -> (index of element=w1190:i32)  [unwired: 1 in]
            n548 = global read "Global - Done.vi" "Done"() -> (w1198:bool[])
            n549 = Replace Array Subset(array=w1198, new element=w1201, index=w1190) -> (w1196:bool[])
            n550 = global write "Global - Done.vi" "Done"(w1196) -> ()
            n551 = case shown="True" w1201 {
              tunnel: w1197 -> [w1209 w1215]
              tunnel: [w1210 w1214] -> w1204
              tunnel: w1203 -> [_ w1216]
              tunnel: w1202 -> [_ w1213]
              tunnel: w1190 -> [_ w1212]
              frame False {
                n552 = call "Communication - Trigger Read IP Address(FGV).vi"("Action"=eFGV_States."Write", "error in"=w1209) -> ("error out"=w1210:errorcluster)  [unwired: 7 in, 2 out]
              }
              frame True {
                n553 = case shown="\"Read Ch Data\"" w1216 {
                  tunnel: w1215 -> [w1217 w1224 w1231 w1237 w1243 w1249 w1255]
                  tunnel: [w1217 w1224 w1231 w1237 w1243 w1249 w1255] -> w1214
                  tunnel: w1213 -> [_ w1222 w1228 w1236 w1242 w1248 w1254]
                  tunnel: w1212 -> [_ w1226 w1232 w1238 w1244 w1250 w1256]
                  frame "Stop", Default {
                  }
                  frame "Read Ch Data" {
                    n554 = Unbundle By Name(w1222) -> ("Channels"=w1221:T12, "Event"=w1220:T10, "Status"=w1219:T9)
                    n555 = global read "Global - Channel.vi" "Data"() -> (w1225:T13)
                    n556 = Bundle("Channels"=w1221, "Event"=w1220, "Status"=w1219) -> (w1218:T14)  [unwired: 1 in]
                    n557 = Replace Array Subset(array=w1225, new element=w1218, index=w1226) -> (w1223:T13)
                    n558 = global write "Global - Channel.vi" "Data"(w1223) -> ()
                  }
                  frame "Read Sensor" {
                    n559 = Unbundle By Name(w1228) -> ("Sensor"=w1227:T15)
                    n560 = global read "Global - Unit.vi" "Unit"() -> (w1229:T16)
                    n561 = Replace Array Subset(array=w1229, new element=w1227, index=w1232) -> (w1230:T16)
                    n562 = global write "Global - Unit.vi" "Unit"(w1230) -> ()
                  }
                  frame "Read ADC" {
                    n563 = Unbundle By Name(w1236) -> ("ADC"=w1233:T17)
                    n564 = global read "Global - ADC.vi" "ADC"() -> (w1235:T18)
                    n565 = Replace Array Subset(array=w1235, new element=w1233, index=w1238) -> (w1234:T18)
                    n566 = global write "Global - ADC.vi" "ADC"(w1234) -> ()
                  }
                  frame "Read PID" {
                    n567 = Unbundle By Name(w1242) -> ("PID"=w1239:T19)
                    n568 = global read "Global - PID.vi" "PID"() -> (w1241:T20)
                    n569 = Replace Array Subset(array=w1241, new element=w1239, index=w1244) -> (w1240:T20)
                    n570 = global write "Global - PID.vi" "PID"(w1240) -> ()
                  }
                  frame "Read System" {
                    n571 = Unbundle By Name(w1248) -> ("System"=w1246:T21)
                    n572 = global read "Global - System.vi" "System"() -> (w1247:T22)
                    n573 = Replace Array Subset(array=w1247, new element=w1246, index=w1250) -> (w1245:T22)
                    n574 = global write "Global - System.vi" "System"(w1245) -> ()
                  }
                  frame "Read Test" {
                    n575 = Unbundle By Name(w1254) -> ("Test"=w1251:T23)
                    n576 = global read "Global - Test.vi" "Test"() -> (w1252:T24)
                    n577 = Replace Array Subset(array=w1252, new element=w1251, index=w1256) -> (w1253:T24)
                    n578 = global write "Global - Test.vi" "Test"(w1253) -> ()
                  }
                }
              }
            }
          }
          frame "Close" {
          }
        }
      }
      frame Error {
        n579 = global read "Global - IP Address.vi" "IP"() -> (w1269:string[])
        n580 = Unbundle By Name(w1270) -> ("source"=w1265:string)
        n581 = Index Array(array=w1269, index=0) -> (element=w1267:string)
        n582 = Concatenate Strings(w1267, " - " ("string"), w1265) -> (w1261:string)
        n583 = call <vilib>:"Clear Errors.vi"("error in (no error)"=w1270) -> ("error out"=w1264:errorcluster)  [unwired: 5 in, 1 out]
        n584 = call "General - Error Log eFGV.vi"("eFGV States"=eFGV_States."Write", "error in (no error)"=w1264, "Error In"=w1261) -> ("error out"=w1263:errorcluster)  [unwired: 6 in, 2 out]
        n585 = Wait (ms)(milliseconds to wait=u32 100) -> ()  [unwired: 1 out]
      }
    }
  }
  n586 = while {
    shift-right: [w1279] -> _
    shift-left: errorcluster {"status"=FALSE, "code"=0, "source"=""} ("error IO") -> [w1280]
    shift-right: [w1277] -> _
    shift-left: Communications_-_State."Init" -> [w1278]
    shift-right: [w1275] -> _
    shift-left: _ -> [w1274]
    stop <- w1276 stop-if-true
    # "Command Processing Loop"
    n587 = case shown="No Error" w1280 {
      selector: w1280 -> [w1286 w1404]
      tunnel: [w1287 w1397] -> w1279
      tunnel: w1278 -> [w1285 _]
      tunnel: [w1284 Communications_-_State."Idle"] -> w1277
      tunnel: [w1283 _] -> w1276
      tunnel: [w1282 w1406] -> w1275
      tunnel: w1274 -> [w1281 w1406]
      frame No Error {
        n588 = case shown="\"Idle\"" w1285 {
          tunnel: [w1290 w1304 w1338 w1394] -> w1287
          tunnel: w1286 -> [w1295 w1303 w1341 w1394]
          tunnel: [Communications_-_State."Idle" w1298 Communications_-_State."Idle" Communications_-_State."Close"] -> w1284
          tunnel: [_ _ _ TRUE] -> w1283
          tunnel: [w1292 w1302 w1340 w1391] -> w1282
          tunnel: w1281 -> [_ w1301 w1340 w1391]
          frame "Init", Default {
            n589 = call "Communication - UDP Command (eFGV).vi"("Action"=eFGV_States."Read", "error in"=w1295) -> ("error out"=w1291:errorcluster, "UDP Ref"=w1289:refnum<user-event>)  [unwired: 7 in, 1 out]
            n590 = register-events(error in=w1291, w1289) -> (reference out=w1288:refnum<event-registration>, error out=w1290:errorcluster)  [unwired: 1 in]
            n591 = Bundle By Name(cluster=T5 {"UDP CMD"={"IP"="", "CMD"=enum."Stop", "Port"="", "Datalog?"=FALSE, "Float"=0.0}, "UDP ref"=refnum, "Unit?"=FALSE, "Read Unit"=[], "Trig?"=FALSE, "UDP Info"=[], "UDP Conn ref"=refnum, "DataLogger"=[], "VISA Ref"=refnum, "Float"=0.0, "Data"={"Test"={"Target Load"=0.0, "Target Disp"=0.0, "Rate"=0.0, "Speed"=0.0}, "Sensor"={"Name"=[], "Unit"=[], "Decimal Point"=[], "Ch Log"=[], "H Alarm"=[], "L Alarm"=[], "H Limit"=[], "L Limit"=[], "Filter"=[], "Gain"=[], "Calib Type"=[]}, "PID"={"SP"=0.0, "PV"=0.0, "kP"=0.0, "kI"=0.0, "kD"=0.0, "FF"=0.0, "Err Band"=0.0, "Max"=0, "Min"=0, "Ts"=0, "Out"=0, "Mode"=0}, "ADC"={"Active Ch"=[], "Filter Type"=0, "Post Filter"=[], "Gain"=[], "FS"=0, "IntOC"=0, "IntFC"=0, "SysOC"=0, "Cofficient"=[], "K"=[], "Max"=0}, "System"={"Out Type"=0, "Inverse"=0, "Monitor"=0, "Reserve"=0, "ACC Time"=0, "Pulse Rev"=0, "Stroke"=0, "Auto Off"=0, "Gear Ratio"=0.0, "Pitch"=0.0, "Max Speed"=0, "Jog Speed"=0, "Disp Coff"=0.0, "Max Load"=0}, "Index"=enum."Ch1", "Datalog"=enum."Empty"}}, "UDP ref"=w1288) -> (w1292:T5)
          }
          frame "Idle" {
            n592 = Unbundle By Name(w1301) -> ("UDP ref"=w1305:refnum<event-registration>)
            n593 = event shown="[1] <FDTI ref>: User Event" {
              selector: w1305 -> [_ _]
              dyn-events: _ -> [_ _]
              timeout: _ -> [_ _]
              tunnel: [w1311 w1313] -> w1299
              tunnel: [w1308 _] -> w1304
              tunnel: w1303 -> [w1308 _]
              tunnel: [w1306 w1323] -> w1302
              tunnel: w1301 -> [w1306 w1322]
              event Timeout {
                n594 = event-data() -> ()  [unwired: 1 in, 1 out]
                n595 = local read "Stop"() -> (w1310:bool)
                n596 = Select(t=Communications_-_State."Close", s=w1310, f=Communications_-_State."Idle") -> (s? t:f=w1311:T1)
              }
              event User Event {
                n597 = event-data() -> ("IP"=w1316:string, "CMD"=w1321:T3, "Data"=w1320:T6)  [unwired: 1 in]
                n598 = global read "Global - IP Address.vi" "IP"() -> (w1319:string[])
                n599 = Index Array(array=w1319, index=10) -> (element=w1317:string)
                n600 = Equal?(x=w1317, y=w1316) -> (x = y?=w1315:bool)
                n601 = Bundle By Name(cluster=w1322, "UDP CMD.IP"=w1316, "UDP CMD.CMD"=w1321, "Data"=w1320) -> (w1323:T5)
                n602 = Select(t=Communications_-_State."Command" ("f"), s=w1315, f=Communications_-_State."Idle") -> (s? t:f=w1313:T1)
              }
            }
            n603 = global read "Global - Hold.vi" "Hold"() -> (w1300:bool)
            n604 = Select(t=Communications_-_State."Idle", s=w1300, f=w1299) -> (s? t:f=w1298:T1)
          }
          frame "Command" {
            (unwired) UDP_-_Command."Stop" ("Enum")
            (unwired) 20
            n605 = Unbundle By Name(w1340) -> ("UDP CMD.CMD"=w1337:T3, "Data"=w1339:T6, "UDP CMD.IP"=w1334:string)
            n606 = global read "Global - Handle.vi" "Handle"() -> (w1329:T7)
            n607 = global read "Global - IP Address.vi" "IP"() -> (w1327:string[])
            n608 = Search 1D Array(1D array=w1327, element=w1334) -> (index of element=w1325:i32)  [unwired: 1 in]
            n609 = Index Array(array=w1329, index=w1325) -> (element=w1333:T8)
            n610 = call "UDP - Write CMD.vi"("CMD"=w1337, "error in"=w1341, "Data"=w1339, "UDP Info"=w1333) -> ("error out"=w1331:errorcluster, "IP Address"=w1326:string, "Data Out"=w1336:T11, "Success"=w1335:bool)  [unwired: 2 in, 2 out]
            n611 = Wait (ms)(milliseconds to wait=u32 5) -> ()  [unwired: 1 out]
            n612 = Search 1D Array(1D array=w1327, element=w1326) -> (index of element=w1324:i32)  [unwired: 1 in]
            n613 = global read "Global - Done.vi" "Done"() -> (w1332:bool[])
            n614 = Replace Array Subset(array=w1332, new element=w1335, index=w1324) -> (w1330:bool[])
            n615 = global write "Global - Done.vi" "Done"(w1330) -> ()
            n616 = case shown="True" w1335 {
              tunnel: w1331 -> [w1343 w1349]
              tunnel: [w1344 w1348] -> w1338
              tunnel: w1337 -> [_ w1350]
              tunnel: w1336 -> [_ w1347]
              tunnel: w1324 -> [_ w1346]
              frame False {
                n617 = call "Communication - Trigger Read IP Address(FGV).vi"("Action"=eFGV_States."Write", "error in"=w1343) -> ("error out"=w1344:errorcluster)  [unwired: 7 in, 2 out]
              }
              frame True {
                n618 = case shown="\"Read Ch Data\"" w1350 {
                  tunnel: w1349 -> [w1351 w1358 w1365 w1371 w1377 w1383 w1389]
                  tunnel: [w1351 w1358 w1365 w1371 w1377 w1383 w1389] -> w1348
                  tunnel: w1347 -> [_ w1356 w1362 w1370 w1376 w1382 w1388]
                  tunnel: w1346 -> [_ w1360 w1366 w1372 w1378 w1384 w1390]
                  frame "Stop", Default {
                  }
                  frame "Read Ch Data" {
                    n619 = Unbundle By Name(w1356) -> ("Channels"=w1355:T12, "Event"=w1354:T10, "Status"=w1353:T9)
                    n620 = global read "Global - Channel.vi" "Data"() -> (w1359:T13)
                    n621 = Bundle("Channels"=w1355, "Event"=w1354, "Status"=w1353) -> (w1352:T14)  [unwired: 1 in]
                    n622 = Replace Array Subset(array=w1359, new element=w1352, index=w1360) -> (w1357:T13)
                    n623 = global write "Global - Channel.vi" "Data"(w1357) -> ()
                  }
                  frame "Read Sensor" {
                    n624 = Unbundle By Name(w1362) -> ("Sensor"=w1361:T15)
                    n625 = global read "Global - Unit.vi" "Unit"() -> (w1363:T16)
                    n626 = Replace Array Subset(array=w1363, new element=w1361, index=w1366) -> (w1364:T16)
                    n627 = global write "Global - Unit.vi" "Unit"(w1364) -> ()
                  }
                  frame "Read ADC" {
                    n628 = Unbundle By Name(w1370) -> ("ADC"=w1367:T17)
                    n629 = global read "Global - ADC.vi" "ADC"() -> (w1369:T18)
                    n630 = Replace Array Subset(array=w1369, new element=w1367, index=w1372) -> (w1368:T18)
                    n631 = global write "Global - ADC.vi" "ADC"(w1368) -> ()
                  }
                  frame "Read PID" {
                    n632 = Unbundle By Name(w1376) -> ("PID"=w1373:T19)
                    n633 = global read "Global - PID.vi" "PID"() -> (w1375:T20)
                    n634 = Replace Array Subset(array=w1375, new element=w1373, index=w1378) -> (w1374:T20)
                    n635 = global write "Global - PID.vi" "PID"(w1374) -> ()
                  }
                  frame "Read System" {
                    n636 = Unbundle By Name(w1382) -> ("System"=w1380:T21)
                    n637 = global read "Global - System.vi" "System"() -> (w1381:T22)
                    n638 = Replace Array Subset(array=w1381, new element=w1380, index=w1384) -> (w1379:T22)
                    n639 = global write "Global - System.vi" "System"(w1379) -> ()
                  }
                  frame "Read Test" {
                    n640 = Unbundle By Name(w1388) -> ("Test"=w1385:T23)
                    n641 = global read "Global - Test.vi" "Test"() -> (w1386:T24)
                    n642 = Replace Array Subset(array=w1386, new element=w1385, index=w1390) -> (w1387:T24)
                    n643 = global write "Global - Test.vi" "Test"(w1387) -> ()
                  }
                }
              }
            }
          }
          frame "Close" {
          }
        }
      }
      frame Error {
        n644 = global read "Global - IP Address.vi" "IP"() -> (w1403:string[])
        n645 = Unbundle By Name(w1404) -> ("source"=w1399:string)
        n646 = Index Array(array=w1403, index=0) -> (element=w1401:string)
        n647 = Concatenate Strings(w1401, " - " ("string"), w1399) -> (w1395:string)
        n648 = call <vilib>:"Clear Errors.vi"("error in (no error)"=w1404) -> ("error out"=w1398:errorcluster)  [unwired: 5 in, 1 out]
        n649 = call "General - Error Log eFGV.vi"("eFGV States"=eFGV_States."Write", "error in (no error)"=w1398, "Error In"=w1395) -> ("error out"=w1397:errorcluster)  [unwired: 6 in, 2 out]
        n650 = Wait (ms)(milliseconds to wait=u32 100) -> ()  [unwired: 1 out]
      }
    }
  }
  n651 = while {
    shift-right: [w1413] -> _
    shift-left: errorcluster {"status"=FALSE, "code"=0, "source"=""} ("error IO") -> [w1414]
    shift-right: [w1411] -> _
    shift-left: Communications_-_State."Init" -> [w1412]
    shift-right: [w1409] -> _
    shift-left: _ -> [w1408]
    stop <- w1410 stop-if-true
    # "Command Processing Loop"
    n652 = case shown="No Error" w1414 {
      selector: w1414 -> [w1420 w1538]
      tunnel: [w1421 w1531] -> w1413
      tunnel: w1412 -> [w1419 _]
      tunnel: [w1418 Communications_-_State."Idle"] -> w1411
      tunnel: [w1417 _] -> w1410
      tunnel: [w1416 w1540] -> w1409
      tunnel: w1408 -> [w1415 w1540]
      frame No Error {
        n653 = case shown="\"Idle\"" w1419 {
          tunnel: [w1424 w1438 w1472 w1528] -> w1421
          tunnel: w1420 -> [w1429 w1437 w1475 w1528]
          tunnel: [Communications_-_State."Idle" w1432 Communications_-_State."Idle" Communications_-_State."Close"] -> w1418
          tunnel: [_ _ _ TRUE] -> w1417
          tunnel: [w1426 w1436 w1474 w1525] -> w1416
          tunnel: w1415 -> [_ w1435 w1474 w1525]
          frame "Init", Default {
            n654 = call "Communication - UDP Command (eFGV).vi"("Action"=eFGV_States."Read", "error in"=w1429) -> ("error out"=w1425:errorcluster, "UDP Ref"=w1423:refnum<user-event>)  [unwired: 7 in, 1 out]
            n655 = register-events(error in=w1425, w1423) -> (reference out=w1422:refnum<event-registration>, error out=w1424:errorcluster)  [unwired: 1 in]
            n656 = Bundle By Name(cluster=T5 {"UDP CMD"={"IP"="", "CMD"=enum."Stop", "Port"="", "Datalog?"=FALSE, "Float"=0.0}, "UDP ref"=refnum, "Unit?"=FALSE, "Read Unit"=[], "Trig?"=FALSE, "UDP Info"=[], "UDP Conn ref"=refnum, "DataLogger"=[], "VISA Ref"=refnum, "Float"=0.0, "Data"={"Test"={"Target Load"=0.0, "Target Disp"=0.0, "Rate"=0.0, "Speed"=0.0}, "Sensor"={"Name"=[], "Unit"=[], "Decimal Point"=[], "Ch Log"=[], "H Alarm"=[], "L Alarm"=[], "H Limit"=[], "L Limit"=[], "Filter"=[], "Gain"=[], "Calib Type"=[]}, "PID"={"SP"=0.0, "PV"=0.0, "kP"=0.0, "kI"=0.0, "kD"=0.0, "FF"=0.0, "Err Band"=0.0, "Max"=0, "Min"=0, "Ts"=0, "Out"=0, "Mode"=0}, "ADC"={"Active Ch"=[], "Filter Type"=0, "Post Filter"=[], "Gain"=[], "FS"=0, "IntOC"=0, "IntFC"=0, "SysOC"=0, "Cofficient"=[], "K"=[], "Max"=0}, "System"={"Out Type"=0, "Inverse"=0, "Monitor"=0, "Reserve"=0, "ACC Time"=0, "Pulse Rev"=0, "Stroke"=0, "Auto Off"=0, "Gear Ratio"=0.0, "Pitch"=0.0, "Max Speed"=0, "Jog Speed"=0, "Disp Coff"=0.0, "Max Load"=0}, "Index"=enum."Ch1", "Datalog"=enum."Empty"}}, "UDP ref"=w1422) -> (w1426:T5)
          }
          frame "Idle" {
            n657 = Unbundle By Name(w1435) -> ("UDP ref"=w1439:refnum<event-registration>)
            n658 = event shown="[1] <FDTI ref>: User Event" {
              selector: w1439 -> [_ _]
              dyn-events: _ -> [_ _]
              timeout: _ -> [_ _]
              tunnel: [w1445 w1447] -> w1433
              tunnel: [w1442 _] -> w1438
              tunnel: w1437 -> [w1442 _]
              tunnel: [w1440 w1457] -> w1436
              tunnel: w1435 -> [w1440 w1456]
              event Timeout {
                n659 = event-data() -> ()  [unwired: 1 in, 1 out]
                n660 = local read "Stop"() -> (w1444:bool)
                n661 = Select(t=Communications_-_State."Close", s=w1444, f=Communications_-_State."Idle") -> (s? t:f=w1445:T1)
              }
              event User Event {
                n662 = event-data() -> ("IP"=w1450:string, "CMD"=w1455:T3, "Data"=w1454:T6)  [unwired: 1 in]
                n663 = global read "Global - IP Address.vi" "IP"() -> (w1453:string[])
                n664 = Index Array(array=w1453, index=16) -> (element=w1451:string)
                n665 = Equal?(x=w1451, y=w1450) -> (x = y?=w1449:bool)
                n666 = Bundle By Name(cluster=w1456, "UDP CMD.IP"=w1450, "UDP CMD.CMD"=w1455, "Data"=w1454) -> (w1457:T5)
                n667 = Select(t=Communications_-_State."Command" ("f"), s=w1449, f=Communications_-_State."Idle") -> (s? t:f=w1447:T1)
              }
            }
            n668 = global read "Global - Hold.vi" "Hold"() -> (w1434:bool)
            n669 = Select(t=Communications_-_State."Idle", s=w1434, f=w1433) -> (s? t:f=w1432:T1)
          }
          frame "Command" {
            (unwired) UDP_-_Command."Stop" ("Enum")
            (unwired) 20
            n670 = Unbundle By Name(w1474) -> ("UDP CMD.CMD"=w1471:T3, "Data"=w1473:T6, "UDP CMD.IP"=w1468:string)
            n671 = global read "Global - Handle.vi" "Handle"() -> (w1463:T7)
            n672 = global read "Global - IP Address.vi" "IP"() -> (w1461:string[])
            n673 = Search 1D Array(1D array=w1461, element=w1468) -> (index of element=w1459:i32)  [unwired: 1 in]
            n674 = Index Array(array=w1463, index=w1459) -> (element=w1467:T8)
            n675 = call "UDP - Write CMD.vi"("CMD"=w1471, "error in"=w1475, "Data"=w1473, "UDP Info"=w1467) -> ("error out"=w1465:errorcluster, "IP Address"=w1460:string, "Data Out"=w1470:T11, "Success"=w1469:bool)  [unwired: 2 in, 2 out]
            n676 = Wait (ms)(milliseconds to wait=u32 5) -> ()  [unwired: 1 out]
            n677 = Search 1D Array(1D array=w1461, element=w1460) -> (index of element=w1458:i32)  [unwired: 1 in]
            n678 = global read "Global - Done.vi" "Done"() -> (w1466:bool[])
            n679 = Replace Array Subset(array=w1466, new element=w1469, index=w1458) -> (w1464:bool[])
            n680 = global write "Global - Done.vi" "Done"(w1464) -> ()
            n681 = case shown="True" w1469 {
              tunnel: w1465 -> [w1477 w1483]
              tunnel: [w1478 w1482] -> w1472
              tunnel: w1471 -> [_ w1484]
              tunnel: w1470 -> [_ w1481]
              tunnel: w1458 -> [_ w1480]
              frame False {
                n682 = call "Communication - Trigger Read IP Address(FGV).vi"("Action"=eFGV_States."Write", "error in"=w1477) -> ("error out"=w1478:errorcluster)  [unwired: 7 in, 2 out]
              }
              frame True {
                n683 = case shown="\"Read Ch Data\"" w1484 {
                  tunnel: w1483 -> [w1485 w1492 w1499 w1505 w1511 w1517 w1523]
                  tunnel: [w1485 w1492 w1499 w1505 w1511 w1517 w1523] -> w1482
                  tunnel: w1481 -> [_ w1490 w1496 w1504 w1510 w1516 w1522]
                  tunnel: w1480 -> [_ w1494 w1500 w1506 w1512 w1518 w1524]
                  frame "Stop", Default {
                  }
                  frame "Read Ch Data" {
                    n684 = Unbundle By Name(w1490) -> ("Channels"=w1489:T12, "Event"=w1488:T10, "Status"=w1487:T9)
                    n685 = global read "Global - Channel.vi" "Data"() -> (w1493:T13)
                    n686 = Bundle("Channels"=w1489, "Event"=w1488, "Status"=w1487) -> (w1486:T14)  [unwired: 1 in]
                    n687 = Replace Array Subset(array=w1493, new element=w1486, index=w1494) -> (w1491:T13)
                    n688 = global write "Global - Channel.vi" "Data"(w1491) -> ()
                  }
                  frame "Read Sensor" {
                    n689 = Unbundle By Name(w1496) -> ("Sensor"=w1495:T15)
                    n690 = global read "Global - Unit.vi" "Unit"() -> (w1497:T16)
                    n691 = Replace Array Subset(array=w1497, new element=w1495, index=w1500) -> (w1498:T16)
                    n692 = global write "Global - Unit.vi" "Unit"(w1498) -> ()
                  }
                  frame "Read ADC" {
                    n693 = Unbundle By Name(w1504) -> ("ADC"=w1501:T17)
                    n694 = global read "Global - ADC.vi" "ADC"() -> (w1503:T18)
                    n695 = Replace Array Subset(array=w1503, new element=w1501, index=w1506) -> (w1502:T18)
                    n696 = global write "Global - ADC.vi" "ADC"(w1502) -> ()
                  }
                  frame "Read PID" {
                    n697 = Unbundle By Name(w1510) -> ("PID"=w1507:T19)
                    n698 = global read "Global - PID.vi" "PID"() -> (w1509:T20)
                    n699 = Replace Array Subset(array=w1509, new element=w1507, index=w1512) -> (w1508:T20)
                    n700 = global write "Global - PID.vi" "PID"(w1508) -> ()
                  }
                  frame "Read System" {
                    n701 = Unbundle By Name(w1516) -> ("System"=w1514:T21)
                    n702 = global read "Global - System.vi" "System"() -> (w1515:T22)
                    n703 = Replace Array Subset(array=w1515, new element=w1514, index=w1518) -> (w1513:T22)
                    n704 = global write "Global - System.vi" "System"(w1513) -> ()
                  }
                  frame "Read Test" {
                    n705 = Unbundle By Name(w1522) -> ("Test"=w1519:T23)
                    n706 = global read "Global - Test.vi" "Test"() -> (w1520:T24)
                    n707 = Replace Array Subset(array=w1520, new element=w1519, index=w1524) -> (w1521:T24)
                    n708 = global write "Global - Test.vi" "Test"(w1521) -> ()
                  }
                }
              }
            }
          }
          frame "Close" {
          }
        }
      }
      frame Error {
        n709 = global read "Global - IP Address.vi" "IP"() -> (w1537:string[])
        n710 = Unbundle By Name(w1538) -> ("source"=w1533:string)
        n711 = Index Array(array=w1537, index=0) -> (element=w1535:string)
        n712 = Concatenate Strings(w1535, " - " ("string"), w1533) -> (w1529:string)
        n713 = call <vilib>:"Clear Errors.vi"("error in (no error)"=w1538) -> ("error out"=w1532:errorcluster)  [unwired: 5 in, 1 out]
        n714 = call "General - Error Log eFGV.vi"("eFGV States"=eFGV_States."Write", "error in (no error)"=w1532, "Error In"=w1529) -> ("error out"=w1531:errorcluster)  [unwired: 6 in, 2 out]
        n715 = Wait (ms)(milliseconds to wait=u32 100) -> ()  [unwired: 1 out]
      }
    }
  }
  n716 = while {
    shift-right: [w1547] -> _
    shift-left: errorcluster {"status"=FALSE, "code"=0, "source"=""} ("error IO") -> [w1548]
    shift-right: [w1545] -> _
    shift-left: Communications_-_State."Init" -> [w1546]
    shift-right: [w1543] -> _
    shift-left: _ -> [w1542]
    stop <- w1544 stop-if-true
    # "Command Processing Loop"
    n717 = case shown="No Error" w1548 {
      selector: w1548 -> [w1554 w1672]
      tunnel: [w1555 w1665] -> w1547
      tunnel: w1546 -> [w1553 _]
      tunnel: [w1552 Communications_-_State."Idle"] -> w1545
      tunnel: [w1551 _] -> w1544
      tunnel: [w1550 w1674] -> w1543
      tunnel: w1542 -> [w1549 w1674]
      frame No Error {
        n718 = case shown="\"Idle\"" w1553 {
          tunnel: [w1558 w1572 w1606 w1662] -> w1555
          tunnel: w1554 -> [w1563 w1571 w1609 w1662]
          tunnel: [Communications_-_State."Idle" w1566 Communications_-_State."Idle" Communications_-_State."Close"] -> w1552
          tunnel: [_ _ _ TRUE] -> w1551
          tunnel: [w1560 w1570 w1608 w1659] -> w1550
          tunnel: w1549 -> [_ w1569 w1608 w1659]
          frame "Init", Default {
            n719 = call "Communication - UDP Command (eFGV).vi"("Action"=eFGV_States."Read", "error in"=w1563) -> ("error out"=w1559:errorcluster, "UDP Ref"=w1557:refnum<user-event>)  [unwired: 7 in, 1 out]
            n720 = register-events(error in=w1559, w1557) -> (reference out=w1556:refnum<event-registration>, error out=w1558:errorcluster)  [unwired: 1 in]
            n721 = Bundle By Name(cluster=T5 {"UDP CMD"={"IP"="", "CMD"=enum."Stop", "Port"="", "Datalog?"=FALSE, "Float"=0.0}, "UDP ref"=refnum, "Unit?"=FALSE, "Read Unit"=[], "Trig?"=FALSE, "UDP Info"=[], "UDP Conn ref"=refnum, "DataLogger"=[], "VISA Ref"=refnum, "Float"=0.0, "Data"={"Test"={"Target Load"=0.0, "Target Disp"=0.0, "Rate"=0.0, "Speed"=0.0}, "Sensor"={"Name"=[], "Unit"=[], "Decimal Point"=[], "Ch Log"=[], "H Alarm"=[], "L Alarm"=[], "H Limit"=[], "L Limit"=[], "Filter"=[], "Gain"=[], "Calib Type"=[]}, "PID"={"SP"=0.0, "PV"=0.0, "kP"=0.0, "kI"=0.0, "kD"=0.0, "FF"=0.0, "Err Band"=0.0, "Max"=0, "Min"=0, "Ts"=0, "Out"=0, "Mode"=0}, "ADC"={"Active Ch"=[], "Filter Type"=0, "Post Filter"=[], "Gain"=[], "FS"=0, "IntOC"=0, "IntFC"=0, "SysOC"=0, "Cofficient"=[], "K"=[], "Max"=0}, "System"={"Out Type"=0, "Inverse"=0, "Monitor"=0, "Reserve"=0, "ACC Time"=0, "Pulse Rev"=0, "Stroke"=0, "Auto Off"=0, "Gear Ratio"=0.0, "Pitch"=0.0, "Max Speed"=0, "Jog Speed"=0, "Disp Coff"=0.0, "Max Load"=0}, "Index"=enum."Ch1", "Datalog"=enum."Empty"}}, "UDP ref"=w1556) -> (w1560:T5)
          }
          frame "Idle" {
            n722 = Unbundle By Name(w1569) -> ("UDP ref"=w1573:refnum<event-registration>)
            n723 = event shown="[1] <FDTI ref>: User Event" {
              selector: w1573 -> [_ _]
              dyn-events: _ -> [_ _]
              timeout: _ -> [_ _]
              tunnel: [w1579 w1581] -> w1567
              tunnel: [w1576 _] -> w1572
              tunnel: w1571 -> [w1576 _]
              tunnel: [w1574 w1591] -> w1570
              tunnel: w1569 -> [w1574 w1590]
              event Timeout {
                n724 = event-data() -> ()  [unwired: 1 in, 1 out]
                n725 = local read "Stop"() -> (w1578:bool)
                n726 = Select(t=Communications_-_State."Close", s=w1578, f=Communications_-_State."Idle") -> (s? t:f=w1579:T1)
              }
              event User Event {
                n727 = event-data() -> ("IP"=w1584:string, "CMD"=w1589:T3, "Data"=w1588:T6)  [unwired: 1 in]
                n728 = global read "Global - IP Address.vi" "IP"() -> (w1587:string[])
                n729 = Index Array(array=w1587, index=18) -> (element=w1585:string)
                n730 = Equal?(x=w1585, y=w1584) -> (x = y?=w1583:bool)
                n731 = Bundle By Name(cluster=w1590, "UDP CMD.IP"=w1584, "UDP CMD.CMD"=w1589, "Data"=w1588) -> (w1591:T5)
                n732 = Select(t=Communications_-_State."Command" ("f"), s=w1583, f=Communications_-_State."Idle") -> (s? t:f=w1581:T1)
              }
            }
            n733 = global read "Global - Hold.vi" "Hold"() -> (w1568:bool)
            n734 = Select(t=Communications_-_State."Idle", s=w1568, f=w1567) -> (s? t:f=w1566:T1)
          }
          frame "Command" {
            (unwired) UDP_-_Command."Stop" ("Enum")
            (unwired) 20
            n735 = Unbundle By Name(w1608) -> ("UDP CMD.CMD"=w1605:T3, "Data"=w1607:T6, "UDP CMD.IP"=w1602:string)
            n736 = global read "Global - Handle.vi" "Handle"() -> (w1597:T7)
            n737 = global read "Global - IP Address.vi" "IP"() -> (w1595:string[])
            n738 = Search 1D Array(1D array=w1595, element=w1602) -> (index of element=w1593:i32)  [unwired: 1 in]
            n739 = Index Array(array=w1597, index=w1593) -> (element=w1601:T8)
            n740 = call "UDP - Write CMD.vi"("CMD"=w1605, "error in"=w1609, "Data"=w1607, "UDP Info"=w1601) -> ("error out"=w1599:errorcluster, "IP Address"=w1594:string, "Data Out"=w1604:T11, "Success"=w1603:bool)  [unwired: 2 in, 2 out]
            n741 = Wait (ms)(milliseconds to wait=u32 5) -> ()  [unwired: 1 out]
            n742 = Search 1D Array(1D array=w1595, element=w1594) -> (index of element=w1592:i32)  [unwired: 1 in]
            n743 = global read "Global - Done.vi" "Done"() -> (w1600:bool[])
            n744 = Replace Array Subset(array=w1600, new element=w1603, index=w1592) -> (w1598:bool[])
            n745 = global write "Global - Done.vi" "Done"(w1598) -> ()
            n746 = case shown="True" w1603 {
              tunnel: w1599 -> [w1611 w1617]
              tunnel: [w1612 w1616] -> w1606
              tunnel: w1605 -> [_ w1618]
              tunnel: w1604 -> [_ w1615]
              tunnel: w1592 -> [_ w1614]
              frame False {
                n747 = call "Communication - Trigger Read IP Address(FGV).vi"("Action"=eFGV_States."Write", "error in"=w1611) -> ("error out"=w1612:errorcluster)  [unwired: 7 in, 2 out]
              }
              frame True {
                n748 = case shown="\"Read Ch Data\"" w1618 {
                  tunnel: w1617 -> [w1619 w1626 w1633 w1639 w1645 w1651 w1657]
                  tunnel: [w1619 w1626 w1633 w1639 w1645 w1651 w1657] -> w1616
                  tunnel: w1615 -> [_ w1624 w1630 w1638 w1644 w1650 w1656]
                  tunnel: w1614 -> [_ w1628 w1634 w1640 w1646 w1652 w1658]
                  frame "Stop", Default {
                  }
                  frame "Read Ch Data" {
                    n749 = Unbundle By Name(w1624) -> ("Channels"=w1623:T12, "Event"=w1622:T10, "Status"=w1621:T9)
                    n750 = global read "Global - Channel.vi" "Data"() -> (w1627:T13)
                    n751 = Bundle("Channels"=w1623, "Event"=w1622, "Status"=w1621) -> (w1620:T14)  [unwired: 1 in]
                    n752 = Replace Array Subset(array=w1627, new element=w1620, index=w1628) -> (w1625:T13)
                    n753 = global write "Global - Channel.vi" "Data"(w1625) -> ()
                  }
                  frame "Read Sensor" {
                    n754 = Unbundle By Name(w1630) -> ("Sensor"=w1629:T15)
                    n755 = global read "Global - Unit.vi" "Unit"() -> (w1631:T16)
                    n756 = Replace Array Subset(array=w1631, new element=w1629, index=w1634) -> (w1632:T16)
                    n757 = global write "Global - Unit.vi" "Unit"(w1632) -> ()
                  }
                  frame "Read ADC" {
                    n758 = Unbundle By Name(w1638) -> ("ADC"=w1635:T17)
                    n759 = global read "Global - ADC.vi" "ADC"() -> (w1637:T18)
                    n760 = Replace Array Subset(array=w1637, new element=w1635, index=w1640) -> (w1636:T18)
                    n761 = global write "Global - ADC.vi" "ADC"(w1636) -> ()
                  }
                  frame "Read PID" {
                    n762 = Unbundle By Name(w1644) -> ("PID"=w1641:T19)
                    n763 = global read "Global - PID.vi" "PID"() -> (w1643:T20)
                    n764 = Replace Array Subset(array=w1643, new element=w1641, index=w1646) -> (w1642:T20)
                    n765 = global write "Global - PID.vi" "PID"(w1642) -> ()
                  }
                  frame "Read System" {
                    n766 = Unbundle By Name(w1650) -> ("System"=w1648:T21)
                    n767 = global read "Global - System.vi" "System"() -> (w1649:T22)
                    n768 = Replace Array Subset(array=w1649, new element=w1648, index=w1652) -> (w1647:T22)
                    n769 = global write "Global - System.vi" "System"(w1647) -> ()
                  }
                  frame "Read Test" {
                    n770 = Unbundle By Name(w1656) -> ("Test"=w1653:T23)
                    n771 = global read "Global - Test.vi" "Test"() -> (w1654:T24)
                    n772 = Replace Array Subset(array=w1654, new element=w1653, index=w1658) -> (w1655:T24)
                    n773 = global write "Global - Test.vi" "Test"(w1655) -> ()
                  }
                }
              }
            }
          }
          frame "Close" {
          }
        }
      }
      frame Error {
        n774 = global read "Global - IP Address.vi" "IP"() -> (w1671:string[])
        n775 = Unbundle By Name(w1672) -> ("source"=w1667:string)
        n776 = Index Array(array=w1671, index=0) -> (element=w1669:string)
        n777 = Concatenate Strings(w1669, " - " ("string"), w1667) -> (w1663:string)
        n778 = call <vilib>:"Clear Errors.vi"("error in (no error)"=w1672) -> ("error out"=w1666:errorcluster)  [unwired: 5 in, 1 out]
        n779 = call "General - Error Log eFGV.vi"("eFGV States"=eFGV_States."Write", "error in (no error)"=w1666, "Error In"=w1663) -> ("error out"=w1665:errorcluster)  [unwired: 6 in, 2 out]
        n780 = Wait (ms)(milliseconds to wait=u32 100) -> ()  [unwired: 1 out]
      }
    }
  }
  n781 = while {
    shift-right: [w1681] -> _
    shift-left: errorcluster {"status"=FALSE, "code"=0, "source"=""} ("error IO") -> [w1682]
    shift-right: [w1679] -> _
    shift-left: Communications_-_State."Init" -> [w1680]
    shift-right: [w1677] -> _
    shift-left: _ -> [w1676]
    stop <- w1678 stop-if-true
    # "Command Processing Loop"
    n782 = case shown="No Error" w1682 {
      selector: w1682 -> [w1688 w1806]
      tunnel: [w1689 w1799] -> w1681
      tunnel: w1680 -> [w1687 _]
      tunnel: [w1686 Communications_-_State."Idle"] -> w1679
      tunnel: [w1685 _] -> w1678
      tunnel: [w1684 w1808] -> w1677
      tunnel: w1676 -> [w1683 w1808]
      frame No Error {
        n783 = case shown="\"Idle\"" w1687 {
          tunnel: [w1692 w1706 w1740 w1796] -> w1689
          tunnel: w1688 -> [w1697 w1705 w1743 w1796]
          tunnel: [Communications_-_State."Idle" w1700 Communications_-_State."Idle" Communications_-_State."Close"] -> w1686
          tunnel: [_ _ _ TRUE] -> w1685
          tunnel: [w1694 w1704 w1742 w1793] -> w1684
          tunnel: w1683 -> [_ w1703 w1742 w1793]
          frame "Init", Default {
            n784 = call "Communication - UDP Command (eFGV).vi"("Action"=eFGV_States."Read", "error in"=w1697) -> ("error out"=w1693:errorcluster, "UDP Ref"=w1691:refnum<user-event>)  [unwired: 7 in, 1 out]
            n785 = register-events(error in=w1693, w1691) -> (reference out=w1690:refnum<event-registration>, error out=w1692:errorcluster)  [unwired: 1 in]
            n786 = Bundle By Name(cluster=T5 {"UDP CMD"={"IP"="", "CMD"=enum."Stop", "Port"="", "Datalog?"=FALSE, "Float"=0.0}, "UDP ref"=refnum, "Unit?"=FALSE, "Read Unit"=[], "Trig?"=FALSE, "UDP Info"=[], "UDP Conn ref"=refnum, "DataLogger"=[], "VISA Ref"=refnum, "Float"=0.0, "Data"={"Test"={"Target Load"=0.0, "Target Disp"=0.0, "Rate"=0.0, "Speed"=0.0}, "Sensor"={"Name"=[], "Unit"=[], "Decimal Point"=[], "Ch Log"=[], "H Alarm"=[], "L Alarm"=[], "H Limit"=[], "L Limit"=[], "Filter"=[], "Gain"=[], "Calib Type"=[]}, "PID"={"SP"=0.0, "PV"=0.0, "kP"=0.0, "kI"=0.0, "kD"=0.0, "FF"=0.0, "Err Band"=0.0, "Max"=0, "Min"=0, "Ts"=0, "Out"=0, "Mode"=0}, "ADC"={"Active Ch"=[], "Filter Type"=0, "Post Filter"=[], "Gain"=[], "FS"=0, "IntOC"=0, "IntFC"=0, "SysOC"=0, "Cofficient"=[], "K"=[], "Max"=0}, "System"={"Out Type"=0, "Inverse"=0, "Monitor"=0, "Reserve"=0, "ACC Time"=0, "Pulse Rev"=0, "Stroke"=0, "Auto Off"=0, "Gear Ratio"=0.0, "Pitch"=0.0, "Max Speed"=0, "Jog Speed"=0, "Disp Coff"=0.0, "Max Load"=0}, "Index"=enum."Ch1", "Datalog"=enum."Empty"}}, "UDP ref"=w1690) -> (w1694:T5)
          }
          frame "Idle" {
            n787 = Unbundle By Name(w1703) -> ("UDP ref"=w1707:refnum<event-registration>)
            n788 = event shown="[1] <FDTI ref>: User Event" {
              selector: w1707 -> [_ _]
              dyn-events: _ -> [_ _]
              timeout: _ -> [_ _]
              tunnel: [w1713 w1715] -> w1701
              tunnel: [w1710 _] -> w1706
              tunnel: w1705 -> [w1710 _]
              tunnel: [w1708 w1725] -> w1704
              tunnel: w1703 -> [w1708 w1724]
              event Timeout {
                n789 = event-data() -> ()  [unwired: 1 in, 1 out]
                n790 = local read "Stop"() -> (w1712:bool)
                n791 = Select(t=Communications_-_State."Close", s=w1712, f=Communications_-_State."Idle") -> (s? t:f=w1713:T1)
              }
              event User Event {
                n792 = event-data() -> ("IP"=w1718:string, "CMD"=w1723:T3, "Data"=w1722:T6)  [unwired: 1 in]
                n793 = global read "Global - IP Address.vi" "IP"() -> (w1721:string[])
                n794 = Index Array(array=w1721, index=4) -> (element=w1719:string)
                n795 = Equal?(x=w1719, y=w1718) -> (x = y?=w1717:bool)
                n796 = Bundle By Name(cluster=w1724, "UDP CMD.IP"=w1718, "UDP CMD.CMD"=w1723, "Data"=w1722) -> (w1725:T5)
                n797 = Select(t=Communications_-_State."Command" ("f"), s=w1717, f=Communications_-_State."Idle") -> (s? t:f=w1715:T1)
              }
            }
            n798 = global read "Global - Hold.vi" "Hold"() -> (w1702:bool)
            n799 = Select(t=Communications_-_State."Idle", s=w1702, f=w1701) -> (s? t:f=w1700:T1)
          }
          frame "Command" {
            (unwired) UDP_-_Command."Stop" ("Enum")
            (unwired) 20
            n800 = Unbundle By Name(w1742) -> ("UDP CMD.CMD"=w1739:T3, "Data"=w1741:T6, "UDP CMD.IP"=w1736:string)
            n801 = global read "Global - Handle.vi" "Handle"() -> (w1731:T7)
            n802 = global read "Global - IP Address.vi" "IP"() -> (w1729:string[])
            n803 = Search 1D Array(1D array=w1729, element=w1736) -> (index of element=w1727:i32)  [unwired: 1 in]
            n804 = Index Array(array=w1731, index=w1727) -> (element=w1735:T8)
            n805 = call "UDP - Write CMD.vi"("CMD"=w1739, "error in"=w1743, "Data"=w1741, "UDP Info"=w1735) -> ("error out"=w1733:errorcluster, "IP Address"=w1728:string, "Data Out"=w1738:T11, "Success"=w1737:bool)  [unwired: 2 in, 2 out]
            n806 = Wait (ms)(milliseconds to wait=u32 5) -> ()  [unwired: 1 out]
            n807 = Search 1D Array(1D array=w1729, element=w1728) -> (index of element=w1726:i32)  [unwired: 1 in]
            n808 = global read "Global - Done.vi" "Done"() -> (w1734:bool[])
            n809 = Replace Array Subset(array=w1734, new element=w1737, index=w1726) -> (w1732:bool[])
            n810 = global write "Global - Done.vi" "Done"(w1732) -> ()
            n811 = case shown="True" w1737 {
              tunnel: w1733 -> [w1745 w1751]
              tunnel: [w1746 w1750] -> w1740
              tunnel: w1739 -> [_ w1752]
              tunnel: w1738 -> [_ w1749]
              tunnel: w1726 -> [_ w1748]
              frame False {
                n812 = call "Communication - Trigger Read IP Address(FGV).vi"("Action"=eFGV_States."Write", "error in"=w1745) -> ("error out"=w1746:errorcluster)  [unwired: 7 in, 2 out]
              }
              frame True {
                n813 = case shown="\"Read Ch Data\"" w1752 {
                  tunnel: w1751 -> [w1753 w1760 w1767 w1773 w1779 w1785 w1791]
                  tunnel: [w1753 w1760 w1767 w1773 w1779 w1785 w1791] -> w1750
                  tunnel: w1749 -> [_ w1758 w1764 w1772 w1778 w1784 w1790]
                  tunnel: w1748 -> [_ w1762 w1768 w1774 w1780 w1786 w1792]
                  frame "Stop", Default {
                  }
                  frame "Read Ch Data" {
                    n814 = Unbundle By Name(w1758) -> ("Channels"=w1757:T12, "Event"=w1756:T10, "Status"=w1755:T9)
                    n815 = global read "Global - Channel.vi" "Data"() -> (w1761:T13)
                    n816 = Bundle("Channels"=w1757, "Event"=w1756, "Status"=w1755) -> (w1754:T14)  [unwired: 1 in]
                    n817 = Replace Array Subset(array=w1761, new element=w1754, index=w1762) -> (w1759:T13)
                    n818 = global write "Global - Channel.vi" "Data"(w1759) -> ()
                  }
                  frame "Read Sensor" {
                    n819 = Unbundle By Name(w1764) -> ("Sensor"=w1763:T15)
                    n820 = global read "Global - Unit.vi" "Unit"() -> (w1765:T16)
                    n821 = Replace Array Subset(array=w1765, new element=w1763, index=w1768) -> (w1766:T16)
                    n822 = global write "Global - Unit.vi" "Unit"(w1766) -> ()
                  }
                  frame "Read ADC" {
                    n823 = Unbundle By Name(w1772) -> ("ADC"=w1769:T17)
                    n824 = global read "Global - ADC.vi" "ADC"() -> (w1771:T18)
                    n825 = Replace Array Subset(array=w1771, new element=w1769, index=w1774) -> (w1770:T18)
                    n826 = global write "Global - ADC.vi" "ADC"(w1770) -> ()
                  }
                  frame "Read PID" {
                    n827 = Unbundle By Name(w1778) -> ("PID"=w1775:T19)
                    n828 = global read "Global - PID.vi" "PID"() -> (w1777:T20)
                    n829 = Replace Array Subset(array=w1777, new element=w1775, index=w1780) -> (w1776:T20)
                    n830 = global write "Global - PID.vi" "PID"(w1776) -> ()
                  }
                  frame "Read System" {
                    n831 = Unbundle By Name(w1784) -> ("System"=w1782:T21)
                    n832 = global read "Global - System.vi" "System"() -> (w1783:T22)
                    n833 = Replace Array Subset(array=w1783, new element=w1782, index=w1786) -> (w1781:T22)
                    n834 = global write "Global - System.vi" "System"(w1781) -> ()
                  }
                  frame "Read Test" {
                    n835 = Unbundle By Name(w1790) -> ("Test"=w1787:T23)
                    n836 = global read "Global - Test.vi" "Test"() -> (w1788:T24)
                    n837 = Replace Array Subset(array=w1788, new element=w1787, index=w1792) -> (w1789:T24)
                    n838 = global write "Global - Test.vi" "Test"(w1789) -> ()
                  }
                }
              }
            }
          }
          frame "Close" {
          }
        }
      }
      frame Error {
        n839 = global read "Global - IP Address.vi" "IP"() -> (w1805:string[])
        n840 = Unbundle By Name(w1806) -> ("source"=w1801:string)
        n841 = Index Array(array=w1805, index=0) -> (element=w1803:string)
        n842 = Concatenate Strings(w1803, " - " ("string"), w1801) -> (w1797:string)
        n843 = call <vilib>:"Clear Errors.vi"("error in (no error)"=w1806) -> ("error out"=w1800:errorcluster)  [unwired: 5 in, 1 out]
        n844 = call "General - Error Log eFGV.vi"("eFGV States"=eFGV_States."Write", "error in (no error)"=w1800, "Error In"=w1797) -> ("error out"=w1799:errorcluster)  [unwired: 6 in, 2 out]
        n845 = Wait (ms)(milliseconds to wait=u32 100) -> ()  [unwired: 1 out]
      }
    }
  }
  n846 = while {
    shift-right: [w1815] -> _
    shift-left: errorcluster {"status"=FALSE, "code"=0, "source"=""} ("error IO") -> [w1816]
    shift-right: [w1813] -> _
    shift-left: Communications_-_State."Init" -> [w1814]
    shift-right: [w1811] -> _
    shift-left: _ -> [w1810]
    stop <- w1812 stop-if-true
    # "Command Processing Loop"
    n847 = case shown="No Error" w1816 {
      selector: w1816 -> [w1822 w1940]
      tunnel: [w1823 w1933] -> w1815
      tunnel: w1814 -> [w1821 _]
      tunnel: [w1820 Communications_-_State."Idle"] -> w1813
      tunnel: [w1819 _] -> w1812
      tunnel: [w1818 w1942] -> w1811
      tunnel: w1810 -> [w1817 w1942]
      frame No Error {
        n848 = case shown="\"Idle\"" w1821 {
          tunnel: [w1826 w1840 w1874 w1930] -> w1823
          tunnel: w1822 -> [w1831 w1839 w1877 w1930]
          tunnel: [Communications_-_State."Idle" w1834 Communications_-_State."Idle" Communications_-_State."Close"] -> w1820
          tunnel: [_ _ _ TRUE] -> w1819
          tunnel: [w1828 w1838 w1876 w1927] -> w1818
          tunnel: w1817 -> [_ w1837 w1876 w1927]
          frame "Init", Default {
            n849 = call "Communication - UDP Command (eFGV).vi"("Action"=eFGV_States."Read", "error in"=w1831) -> ("error out"=w1827:errorcluster, "UDP Ref"=w1825:refnum<user-event>)  [unwired: 7 in, 1 out]
            n850 = register-events(error in=w1827, w1825) -> (reference out=w1824:refnum<event-registration>, error out=w1826:errorcluster)  [unwired: 1 in]
            n851 = Bundle By Name(cluster=T5 {"UDP CMD"={"IP"="", "CMD"=enum."Stop", "Port"="", "Datalog?"=FALSE, "Float"=0.0}, "UDP ref"=refnum, "Unit?"=FALSE, "Read Unit"=[], "Trig?"=FALSE, "UDP Info"=[], "UDP Conn ref"=refnum, "DataLogger"=[], "VISA Ref"=refnum, "Float"=0.0, "Data"={"Test"={"Target Load"=0.0, "Target Disp"=0.0, "Rate"=0.0, "Speed"=0.0}, "Sensor"={"Name"=[], "Unit"=[], "Decimal Point"=[], "Ch Log"=[], "H Alarm"=[], "L Alarm"=[], "H Limit"=[], "L Limit"=[], "Filter"=[], "Gain"=[], "Calib Type"=[]}, "PID"={"SP"=0.0, "PV"=0.0, "kP"=0.0, "kI"=0.0, "kD"=0.0, "FF"=0.0, "Err Band"=0.0, "Max"=0, "Min"=0, "Ts"=0, "Out"=0, "Mode"=0}, "ADC"={"Active Ch"=[], "Filter Type"=0, "Post Filter"=[], "Gain"=[], "FS"=0, "IntOC"=0, "IntFC"=0, "SysOC"=0, "Cofficient"=[], "K"=[], "Max"=0}, "System"={"Out Type"=0, "Inverse"=0, "Monitor"=0, "Reserve"=0, "ACC Time"=0, "Pulse Rev"=0, "Stroke"=0, "Auto Off"=0, "Gear Ratio"=0.0, "Pitch"=0.0, "Max Speed"=0, "Jog Speed"=0, "Disp Coff"=0.0, "Max Load"=0}, "Index"=enum."Ch1", "Datalog"=enum."Empty"}}, "UDP ref"=w1824) -> (w1828:T5)
          }
          frame "Idle" {
            n852 = Unbundle By Name(w1837) -> ("UDP ref"=w1841:refnum<event-registration>)
            n853 = event shown="[1] <FDTI ref>: User Event" {
              selector: w1841 -> [_ _]
              dyn-events: _ -> [_ _]
              timeout: _ -> [_ _]
              tunnel: [w1847 w1849] -> w1835
              tunnel: [w1844 _] -> w1840
              tunnel: w1839 -> [w1844 _]
              tunnel: [w1842 w1859] -> w1838
              tunnel: w1837 -> [w1842 w1858]
              event Timeout {
                n854 = event-data() -> ()  [unwired: 1 in, 1 out]
                n855 = local read "Stop"() -> (w1846:bool)
                n856 = Select(t=Communications_-_State."Close", s=w1846, f=Communications_-_State."Idle") -> (s? t:f=w1847:T1)
              }
              event User Event {
                n857 = event-data() -> ("IP"=w1852:string, "CMD"=w1857:T3, "Data"=w1856:T6)  [unwired: 1 in]
                n858 = global read "Global - IP Address.vi" "IP"() -> (w1855:string[])
                n859 = Index Array(array=w1855, index=6) -> (element=w1853:string)
                n860 = Equal?(x=w1853, y=w1852) -> (x = y?=w1851:bool)
                n861 = Bundle By Name(cluster=w1858, "UDP CMD.IP"=w1852, "UDP CMD.CMD"=w1857, "Data"=w1856) -> (w1859:T5)
                n862 = Select(t=Communications_-_State."Command" ("f"), s=w1851, f=Communications_-_State."Idle") -> (s? t:f=w1849:T1)
              }
            }
            n863 = global read "Global - Hold.vi" "Hold"() -> (w1836:bool)
            n864 = Select(t=Communications_-_State."Idle", s=w1836, f=w1835) -> (s? t:f=w1834:T1)
          }
          frame "Command" {
            (unwired) UDP_-_Command."Stop" ("Enum")
            (unwired) 20
            n865 = Unbundle By Name(w1876) -> ("UDP CMD.CMD"=w1873:T3, "Data"=w1875:T6, "UDP CMD.IP"=w1870:string)
            n866 = global read "Global - Handle.vi" "Handle"() -> (w1865:T7)
            n867 = global read "Global - IP Address.vi" "IP"() -> (w1863:string[])
            n868 = Search 1D Array(1D array=w1863, element=w1870) -> (index of element=w1861:i32)  [unwired: 1 in]
            n869 = Index Array(array=w1865, index=w1861) -> (element=w1869:T8)
            n870 = call "UDP - Write CMD.vi"("CMD"=w1873, "error in"=w1877, "Data"=w1875, "UDP Info"=w1869) -> ("error out"=w1867:errorcluster, "IP Address"=w1862:string, "Data Out"=w1872:T11, "Success"=w1871:bool)  [unwired: 2 in, 2 out]
            n871 = Wait (ms)(milliseconds to wait=u32 5) -> ()  [unwired: 1 out]
            n872 = Search 1D Array(1D array=w1863, element=w1862) -> (index of element=w1860:i32)  [unwired: 1 in]
            n873 = global read "Global - Done.vi" "Done"() -> (w1868:bool[])
            n874 = Replace Array Subset(array=w1868, new element=w1871, index=w1860) -> (w1866:bool[])
            n875 = global write "Global - Done.vi" "Done"(w1866) -> ()
            n876 = case shown="True" w1871 {
              tunnel: w1867 -> [w1879 w1885]
              tunnel: [w1880 w1884] -> w1874
              tunnel: w1873 -> [_ w1886]
              tunnel: w1872 -> [_ w1883]
              tunnel: w1860 -> [_ w1882]
              frame False {
                n877 = call "Communication - Trigger Read IP Address(FGV).vi"("Action"=eFGV_States."Write", "error in"=w1879) -> ("error out"=w1880:errorcluster)  [unwired: 7 in, 2 out]
              }
              frame True {
                n878 = case shown="\"Read Ch Data\"" w1886 {
                  tunnel: w1885 -> [w1887 w1894 w1901 w1907 w1913 w1919 w1925]
                  tunnel: [w1887 w1894 w1901 w1907 w1913 w1919 w1925] -> w1884
                  tunnel: w1883 -> [_ w1892 w1898 w1906 w1912 w1918 w1924]
                  tunnel: w1882 -> [_ w1896 w1902 w1908 w1914 w1920 w1926]
                  frame "Stop", Default {
                  }
                  frame "Read Ch Data" {
                    n879 = Unbundle By Name(w1892) -> ("Channels"=w1891:T12, "Event"=w1890:T10, "Status"=w1889:T9)
                    n880 = global read "Global - Channel.vi" "Data"() -> (w1895:T13)
                    n881 = Bundle("Channels"=w1891, "Event"=w1890, "Status"=w1889) -> (w1888:T14)  [unwired: 1 in]
                    n882 = Replace Array Subset(array=w1895, new element=w1888, index=w1896) -> (w1893:T13)
                    n883 = global write "Global - Channel.vi" "Data"(w1893) -> ()
                  }
                  frame "Read Sensor" {
                    n884 = Unbundle By Name(w1898) -> ("Sensor"=w1897:T15)
                    n885 = global read "Global - Unit.vi" "Unit"() -> (w1899:T16)
                    n886 = Replace Array Subset(array=w1899, new element=w1897, index=w1902) -> (w1900:T16)
                    n887 = global write "Global - Unit.vi" "Unit"(w1900) -> ()
                  }
                  frame "Read ADC" {
                    n888 = Unbundle By Name(w1906) -> ("ADC"=w1903:T17)
                    n889 = global read "Global - ADC.vi" "ADC"() -> (w1905:T18)
                    n890 = Replace Array Subset(array=w1905, new element=w1903, index=w1908) -> (w1904:T18)
                    n891 = global write "Global - ADC.vi" "ADC"(w1904) -> ()
                  }
                  frame "Read PID" {
                    n892 = Unbundle By Name(w1912) -> ("PID"=w1909:T19)
                    n893 = global read "Global - PID.vi" "PID"() -> (w1911:T20)
                    n894 = Replace Array Subset(array=w1911, new element=w1909, index=w1914) -> (w1910:T20)
                    n895 = global write "Global - PID.vi" "PID"(w1910) -> ()
                  }
                  frame "Read System" {
                    n896 = Unbundle By Name(w1918) -> ("System"=w1916:T21)
                    n897 = global read "Global - System.vi" "System"() -> (w1917:T22)
                    n898 = Replace Array Subset(array=w1917, new element=w1916, index=w1920) -> (w1915:T22)
                    n899 = global write "Global - System.vi" "System"(w1915) -> ()
                  }
                  frame "Read Test" {
                    n900 = Unbundle By Name(w1924) -> ("Test"=w1921:T23)
                    n901 = global read "Global - Test.vi" "Test"() -> (w1922:T24)
                    n902 = Replace Array Subset(array=w1922, new element=w1921, index=w1926) -> (w1923:T24)
                    n903 = global write "Global - Test.vi" "Test"(w1923) -> ()
                  }
                }
              }
            }
          }
          frame "Close" {
          }
        }
      }
      frame Error {
        n904 = global read "Global - IP Address.vi" "IP"() -> (w1939:string[])
        n905 = Unbundle By Name(w1940) -> ("source"=w1935:string)
        n906 = Index Array(array=w1939, index=0) -> (element=w1937:string)
        n907 = Concatenate Strings(w1937, " - " ("string"), w1935) -> (w1931:string)
        n908 = call <vilib>:"Clear Errors.vi"("error in (no error)"=w1940) -> ("error out"=w1934:errorcluster)  [unwired: 5 in, 1 out]
        n909 = call "General - Error Log eFGV.vi"("eFGV States"=eFGV_States."Write", "error in (no error)"=w1934, "Error In"=w1931) -> ("error out"=w1933:errorcluster)  [unwired: 6 in, 2 out]
        n910 = Wait (ms)(milliseconds to wait=u32 100) -> ()  [unwired: 1 out]
      }
    }
  }
  n911 = while {
    shift-right: [w1949] -> _
    shift-left: errorcluster {"status"=FALSE, "code"=0, "source"=""} ("error IO") -> [w1950]
    shift-right: [w1947] -> _
    shift-left: Communications_-_State."Init" -> [w1948]
    shift-right: [w1945] -> _
    shift-left: _ -> [w1944]
    stop <- w1946 stop-if-true
    # "Command Processing Loop"
    n912 = case shown="No Error" w1950 {
      selector: w1950 -> [w1956 w2074]
      tunnel: [w1957 w2067] -> w1949
      tunnel: w1948 -> [w1955 _]
      tunnel: [w1954 Communications_-_State."Idle"] -> w1947
      tunnel: [w1953 _] -> w1946
      tunnel: [w1952 w2076] -> w1945
      tunnel: w1944 -> [w1951 w2076]
      frame No Error {
        n913 = case shown="\"Idle\"" w1955 {
          tunnel: [w1960 w1974 w2008 w2064] -> w1957
          tunnel: w1956 -> [w1965 w1973 w2011 w2064]
          tunnel: [Communications_-_State."Idle" w1968 Communications_-_State."Idle" Communications_-_State."Close"] -> w1954
          tunnel: [_ _ _ TRUE] -> w1953
          tunnel: [w1962 w1972 w2010 w2061] -> w1952
          tunnel: w1951 -> [_ w1971 w2010 w2061]
          frame "Init", Default {
            n914 = call "Communication - UDP Command (eFGV).vi"("Action"=eFGV_States."Read", "error in"=w1965) -> ("error out"=w1961:errorcluster, "UDP Ref"=w1959:refnum<user-event>)  [unwired: 7 in, 1 out]
            n915 = register-events(error in=w1961, w1959) -> (reference out=w1958:refnum<event-registration>, error out=w1960:errorcluster)  [unwired: 1 in]
            n916 = Bundle By Name(cluster=T5 {"UDP CMD"={"IP"="", "CMD"=enum."Stop", "Port"="", "Datalog?"=FALSE, "Float"=0.0}, "UDP ref"=refnum, "Unit?"=FALSE, "Read Unit"=[], "Trig?"=FALSE, "UDP Info"=[], "UDP Conn ref"=refnum, "DataLogger"=[], "VISA Ref"=refnum, "Float"=0.0, "Data"={"Test"={"Target Load"=0.0, "Target Disp"=0.0, "Rate"=0.0, "Speed"=0.0}, "Sensor"={"Name"=[], "Unit"=[], "Decimal Point"=[], "Ch Log"=[], "H Alarm"=[], "L Alarm"=[], "H Limit"=[], "L Limit"=[], "Filter"=[], "Gain"=[], "Calib Type"=[]}, "PID"={"SP"=0.0, "PV"=0.0, "kP"=0.0, "kI"=0.0, "kD"=0.0, "FF"=0.0, "Err Band"=0.0, "Max"=0, "Min"=0, "Ts"=0, "Out"=0, "Mode"=0}, "ADC"={"Active Ch"=[], "Filter Type"=0, "Post Filter"=[], "Gain"=[], "FS"=0, "IntOC"=0, "IntFC"=0, "SysOC"=0, "Cofficient"=[], "K"=[], "Max"=0}, "System"={"Out Type"=0, "Inverse"=0, "Monitor"=0, "Reserve"=0, "ACC Time"=0, "Pulse Rev"=0, "Stroke"=0, "Auto Off"=0, "Gear Ratio"=0.0, "Pitch"=0.0, "Max Speed"=0, "Jog Speed"=0, "Disp Coff"=0.0, "Max Load"=0}, "Index"=enum."Ch1", "Datalog"=enum."Empty"}}, "UDP ref"=w1958) -> (w1962:T5)
          }
          frame "Idle" {
            n917 = Unbundle By Name(w1971) -> ("UDP ref"=w1975:refnum<event-registration>)
            n918 = event shown="[1] <FDTI ref>: User Event" {
              selector: w1975 -> [_ _]
              dyn-events: _ -> [_ _]
              timeout: _ -> [_ _]
              tunnel: [w1981 w1983] -> w1969
              tunnel: [w1978 _] -> w1974
              tunnel: w1973 -> [w1978 _]
              tunnel: [w1976 w1993] -> w1972
              tunnel: w1971 -> [w1976 w1992]
              event Timeout {
                n919 = event-data() -> ()  [unwired: 1 in, 1 out]
                n920 = local read "Stop"() -> (w1980:bool)
                n921 = Select(t=Communications_-_State."Close", s=w1980, f=Communications_-_State."Idle") -> (s? t:f=w1981:T1)
              }
              event User Event {
                n922 = event-data() -> ("IP"=w1986:string, "CMD"=w1991:T3, "Data"=w1990:T6)  [unwired: 1 in]
                n923 = global read "Global - IP Address.vi" "IP"() -> (w1989:string[])
                n924 = Index Array(array=w1989, index=0) -> (element=w1987:string)
                n925 = Equal?(x=w1987, y=w1986) -> (x = y?=w1985:bool)
                n926 = Bundle By Name(cluster=w1992, "UDP CMD.IP"=w1986, "UDP CMD.CMD"=w1991, "Data"=w1990) -> (w1993:T5)
                n927 = Select(t=Communications_-_State."Command" ("f"), s=w1985, f=Communications_-_State."Idle") -> (s? t:f=w1983:T1)
              }
            }
            n928 = global read "Global - Hold.vi" "Hold"() -> (w1970:bool)
            n929 = Select(t=Communications_-_State."Idle", s=w1970, f=w1969) -> (s? t:f=w1968:T1)
          }
          frame "Command" {
            (unwired) UDP_-_Command."Stop" ("Enum")
            (unwired) 20
            n930 = Unbundle By Name(w2010) -> ("UDP CMD.CMD"=w2007:T3, "Data"=w2009:T6, "UDP CMD.IP"=w2004:string)
            n931 = global read "Global - Handle.vi" "Handle"() -> (w1999:T7)
            n932 = global read "Global - IP Address.vi" "IP"() -> (w1997:string[])
            n933 = Search 1D Array(1D array=w1997, element=w2004) -> (index of element=w1995:i32)  [unwired: 1 in]
            n934 = Index Array(array=w1999, index=w1995) -> (element=w2003:T8)
            n935 = call "UDP - Write CMD.vi"("CMD"=w2007, "error in"=w2011, "Data"=w2009, "UDP Info"=w2003) -> ("error out"=w2001:errorcluster, "IP Address"=w1996:string, "Data Out"=w2006:T11, "Success"=w2005:bool)  [unwired: 2 in, 2 out]
            n936 = Wait (ms)(milliseconds to wait=u32 5) -> ()  [unwired: 1 out]
            n937 = Search 1D Array(1D array=w1997, element=w1996) -> (index of element=w1994:i32)  [unwired: 1 in]
            n938 = global read "Global - Done.vi" "Done"() -> (w2002:bool[])
            n939 = Replace Array Subset(array=w2002, new element=w2005, index=w1994) -> (w2000:bool[])
            n940 = global write "Global - Done.vi" "Done"(w2000) -> ()
            n941 = case shown="True" w2005 {
              tunnel: w2001 -> [w2013 w2019]
              tunnel: [w2014 w2018] -> w2008
              tunnel: w2007 -> [_ w2020]
              tunnel: w2006 -> [_ w2017]
              tunnel: w1994 -> [_ w2016]
              frame False {
                n942 = call "Communication - Trigger Read IP Address(FGV).vi"("Action"=eFGV_States."Write", "error in"=w2013) -> ("error out"=w2014:errorcluster)  [unwired: 7 in, 2 out]
              }
              frame True {
                n943 = case shown="\"Read Ch Data\"" w2020 {
                  tunnel: w2019 -> [w2021 w2028 w2035 w2041 w2047 w2053 w2059]
                  tunnel: [w2021 w2028 w2035 w2041 w2047 w2053 w2059] -> w2018
                  tunnel: w2017 -> [_ w2026 w2032 w2040 w2046 w2052 w2058]
                  tunnel: w2016 -> [_ w2030 w2036 w2042 w2048 w2054 w2060]
                  frame "Stop", Default {
                  }
                  frame "Read Ch Data" {
                    n944 = Unbundle By Name(w2026) -> ("Channels"=w2025:T12, "Event"=w2024:T10, "Status"=w2023:T9)
                    n945 = global read "Global - Channel.vi" "Data"() -> (w2029:T13)
                    n946 = Bundle("Channels"=w2025, "Event"=w2024, "Status"=w2023) -> (w2022:T14)  [unwired: 1 in]
                    n947 = Replace Array Subset(array=w2029, new element=w2022, index=w2030) -> (w2027:T13)
                    n948 = global write "Global - Channel.vi" "Data"(w2027) -> ()
                  }
                  frame "Read Sensor" {
                    n949 = Unbundle By Name(w2032) -> ("Sensor"=w2031:T15)
                    n950 = global read "Global - Unit.vi" "Unit"() -> (w2033:T16)
                    n951 = Replace Array Subset(array=w2033, new element=w2031, index=w2036) -> (w2034:T16)
                    n952 = global write "Global - Unit.vi" "Unit"(w2034) -> ()
                  }
                  frame "Read ADC" {
                    n953 = Unbundle By Name(w2040) -> ("ADC"=w2037:T17)
                    n954 = global read "Global - ADC.vi" "ADC"() -> (w2039:T18)
                    n955 = Replace Array Subset(array=w2039, new element=w2037, index=w2042) -> (w2038:T18)
                    n956 = global write "Global - ADC.vi" "ADC"(w2038) -> ()
                  }
                  frame "Read PID" {
                    n957 = Unbundle By Name(w2046) -> ("PID"=w2043:T19)
                    n958 = global read "Global - PID.vi" "PID"() -> (w2045:T20)
                    n959 = Replace Array Subset(array=w2045, new element=w2043, index=w2048) -> (w2044:T20)
                    n960 = global write "Global - PID.vi" "PID"(w2044) -> ()
                  }
                  frame "Read System" {
                    n961 = Unbundle By Name(w2052) -> ("System"=w2050:T21)
                    n962 = global read "Global - System.vi" "System"() -> (w2051:T22)
                    n963 = Replace Array Subset(array=w2051, new element=w2050, index=w2054) -> (w2049:T22)
                    n964 = global write "Global - System.vi" "System"(w2049) -> ()
                  }
                  frame "Read Test" {
                    n965 = Unbundle By Name(w2058) -> ("Test"=w2055:T23)
                    n966 = global read "Global - Test.vi" "Test"() -> (w2056:T24)
                    n967 = Replace Array Subset(array=w2056, new element=w2055, index=w2060) -> (w2057:T24)
                    n968 = global write "Global - Test.vi" "Test"(w2057) -> ()
                  }
                }
              }
            }
          }
          frame "Close" {
          }
        }
      }
      frame Error {
        n969 = global read "Global - IP Address.vi" "IP"() -> (w2073:string[])
        n970 = Unbundle By Name(w2074) -> ("source"=w2069:string)
        n971 = Index Array(array=w2073, index=0) -> (element=w2071:string)
        n972 = Concatenate Strings(w2071, " - " ("string"), w2069) -> (w2065:string)
        n973 = call <vilib>:"Clear Errors.vi"("error in (no error)"=w2074) -> ("error out"=w2068:errorcluster)  [unwired: 5 in, 1 out]
        n974 = call "General - Error Log eFGV.vi"("eFGV States"=eFGV_States."Write", "error in (no error)"=w2068, "Error In"=w2065) -> ("error out"=w2067:errorcluster)  [unwired: 6 in, 2 out]
        n975 = Wait (ms)(milliseconds to wait=u32 100) -> ()  [unwired: 1 out]
      }
    }
  }
  n976 = while {
    shift-right: [w2083] -> _
    shift-left: errorcluster {"status"=FALSE, "code"=0, "source"=""} ("error IO") -> [w2084]
    shift-right: [w2081] -> _
    shift-left: Communications_-_State."Init" -> [w2082]
    shift-right: [w2079] -> _
    shift-left: _ -> [w2078]
    stop <- w2080 stop-if-true
    # "Command Processing Loop"
    n977 = case shown="No Error" w2084 {
      selector: w2084 -> [w2090 w2208]
      tunnel: [w2091 w2201] -> w2083
      tunnel: w2082 -> [w2089 _]
      tunnel: [w2088 Communications_-_State."Idle"] -> w2081
      tunnel: [w2087 _] -> w2080
      tunnel: [w2086 w2210] -> w2079
      tunnel: w2078 -> [w2085 w2210]
      frame No Error {
        n978 = case shown="\"Idle\"" w2089 {
          tunnel: [w2094 w2108 w2142 w2198] -> w2091
          tunnel: w2090 -> [w2099 w2107 w2145 w2198]
          tunnel: [Communications_-_State."Idle" w2102 Communications_-_State."Idle" Communications_-_State."Close"] -> w2088
          tunnel: [_ _ _ TRUE] -> w2087
          tunnel: [w2096 w2106 w2144 w2195] -> w2086
          tunnel: w2085 -> [_ w2105 w2144 w2195]
          frame "Init", Default {
            n979 = call "Communication - UDP Command (eFGV).vi"("Action"=eFGV_States."Read", "error in"=w2099) -> ("error out"=w2095:errorcluster, "UDP Ref"=w2093:refnum<user-event>)  [unwired: 7 in, 1 out]
            n980 = register-events(error in=w2095, w2093) -> (reference out=w2092:refnum<event-registration>, error out=w2094:errorcluster)  [unwired: 1 in]
            n981 = Bundle By Name(cluster=T5 {"UDP CMD"={"IP"="", "CMD"=enum."Stop", "Port"="", "Datalog?"=FALSE, "Float"=0.0}, "UDP ref"=refnum, "Unit?"=FALSE, "Read Unit"=[], "Trig?"=FALSE, "UDP Info"=[], "UDP Conn ref"=refnum, "DataLogger"=[], "VISA Ref"=refnum, "Float"=0.0, "Data"={"Test"={"Target Load"=0.0, "Target Disp"=0.0, "Rate"=0.0, "Speed"=0.0}, "Sensor"={"Name"=[], "Unit"=[], "Decimal Point"=[], "Ch Log"=[], "H Alarm"=[], "L Alarm"=[], "H Limit"=[], "L Limit"=[], "Filter"=[], "Gain"=[], "Calib Type"=[]}, "PID"={"SP"=0.0, "PV"=0.0, "kP"=0.0, "kI"=0.0, "kD"=0.0, "FF"=0.0, "Err Band"=0.0, "Max"=0, "Min"=0, "Ts"=0, "Out"=0, "Mode"=0}, "ADC"={"Active Ch"=[], "Filter Type"=0, "Post Filter"=[], "Gain"=[], "FS"=0, "IntOC"=0, "IntFC"=0, "SysOC"=0, "Cofficient"=[], "K"=[], "Max"=0}, "System"={"Out Type"=0, "Inverse"=0, "Monitor"=0, "Reserve"=0, "ACC Time"=0, "Pulse Rev"=0, "Stroke"=0, "Auto Off"=0, "Gear Ratio"=0.0, "Pitch"=0.0, "Max Speed"=0, "Jog Speed"=0, "Disp Coff"=0.0, "Max Load"=0}, "Index"=enum."Ch1", "Datalog"=enum."Empty"}}, "UDP ref"=w2092) -> (w2096:T5)
          }
          frame "Idle" {
            n982 = Unbundle By Name(w2105) -> ("UDP ref"=w2109:refnum<event-registration>)
            n983 = event shown="[1] <FDTI ref>: User Event" {
              selector: w2109 -> [_ _]
              dyn-events: _ -> [_ _]
              timeout: _ -> [_ _]
              tunnel: [w2115 w2117] -> w2103
              tunnel: [w2112 _] -> w2108
              tunnel: w2107 -> [w2112 _]
              tunnel: [w2110 w2127] -> w2106
              tunnel: w2105 -> [w2110 w2126]
              event Timeout {
                n984 = event-data() -> ()  [unwired: 1 in, 1 out]
                n985 = local read "Stop"() -> (w2114:bool)
                n986 = Select(t=Communications_-_State."Close", s=w2114, f=Communications_-_State."Idle") -> (s? t:f=w2115:T1)
              }
              event User Event {
                n987 = event-data() -> ("IP"=w2120:string, "CMD"=w2125:T3, "Data"=w2124:T6)  [unwired: 1 in]
                n988 = global read "Global - IP Address.vi" "IP"() -> (w2123:string[])
                n989 = Index Array(array=w2123, index=2) -> (element=w2121:string)
                n990 = Equal?(x=w2121, y=w2120) -> (x = y?=w2119:bool)
                n991 = Bundle By Name(cluster=w2126, "UDP CMD.IP"=w2120, "UDP CMD.CMD"=w2125, "Data"=w2124) -> (w2127:T5)
                n992 = Select(t=Communications_-_State."Command" ("f"), s=w2119, f=Communications_-_State."Idle") -> (s? t:f=w2117:T1)
              }
            }
            n993 = global read "Global - Hold.vi" "Hold"() -> (w2104:bool)
            n994 = Select(t=Communications_-_State."Idle", s=w2104, f=w2103) -> (s? t:f=w2102:T1)
          }
          frame "Command" {
            (unwired) UDP_-_Command."Stop" ("Enum")
            (unwired) 20
            n995 = Unbundle By Name(w2144) -> ("UDP CMD.CMD"=w2141:T3, "Data"=w2143:T6, "UDP CMD.IP"=w2138:string)
            n996 = global read "Global - Handle.vi" "Handle"() -> (w2133:T7)
            n997 = global read "Global - IP Address.vi" "IP"() -> (w2131:string[])
            n998 = Search 1D Array(1D array=w2131, element=w2138) -> (index of element=w2129:i32)  [unwired: 1 in]
            n999 = Index Array(array=w2133, index=w2129) -> (element=w2137:T8)
            n1000 = call "UDP - Write CMD.vi"("CMD"=w2141, "error in"=w2145, "Data"=w2143, "UDP Info"=w2137) -> ("error out"=w2135:errorcluster, "IP Address"=w2130:string, "Data Out"=w2140:T11, "Success"=w2139:bool)  [unwired: 2 in, 2 out]
            n1001 = Wait (ms)(milliseconds to wait=u32 5) -> ()  [unwired: 1 out]
            n1002 = Search 1D Array(1D array=w2131, element=w2130) -> (index of element=w2128:i32)  [unwired: 1 in]
            n1003 = global read "Global - Done.vi" "Done"() -> (w2136:bool[])
            n1004 = Replace Array Subset(array=w2136, new element=w2139, index=w2128) -> (w2134:bool[])
            n1005 = global write "Global - Done.vi" "Done"(w2134) -> ()
            n1006 = case shown="True" w2139 {
              tunnel: w2135 -> [w2147 w2153]
              tunnel: [w2148 w2152] -> w2142
              tunnel: w2141 -> [_ w2154]
              tunnel: w2140 -> [_ w2151]
              tunnel: w2128 -> [_ w2150]
              frame False {
                n1007 = call "Communication - Trigger Read IP Address(FGV).vi"("Action"=eFGV_States."Write", "error in"=w2147) -> ("error out"=w2148:errorcluster)  [unwired: 7 in, 2 out]
              }
              frame True {
                n1008 = case shown="\"Read Ch Data\"" w2154 {
                  tunnel: w2153 -> [w2155 w2162 w2169 w2175 w2181 w2187 w2193]
                  tunnel: [w2155 w2162 w2169 w2175 w2181 w2187 w2193] -> w2152
                  tunnel: w2151 -> [_ w2160 w2166 w2174 w2180 w2186 w2192]
                  tunnel: w2150 -> [_ w2164 w2170 w2176 w2182 w2188 w2194]
                  frame "Stop", Default {
                  }
                  frame "Read Ch Data" {
                    n1009 = Unbundle By Name(w2160) -> ("Channels"=w2159:T12, "Event"=w2158:T10, "Status"=w2157:T9)
                    n1010 = global read "Global - Channel.vi" "Data"() -> (w2163:T13)
                    n1011 = Bundle("Channels"=w2159, "Event"=w2158, "Status"=w2157) -> (w2156:T14)  [unwired: 1 in]
                    n1012 = Replace Array Subset(array=w2163, new element=w2156, index=w2164) -> (w2161:T13)
                    n1013 = global write "Global - Channel.vi" "Data"(w2161) -> ()
                  }
                  frame "Read Sensor" {
                    n1014 = Unbundle By Name(w2166) -> ("Sensor"=w2165:T15)
                    n1015 = global read "Global - Unit.vi" "Unit"() -> (w2167:T16)
                    n1016 = Replace Array Subset(array=w2167, new element=w2165, index=w2170) -> (w2168:T16)
                    n1017 = global write "Global - Unit.vi" "Unit"(w2168) -> ()
                  }
                  frame "Read ADC" {
                    n1018 = Unbundle By Name(w2174) -> ("ADC"=w2171:T17)
                    n1019 = global read "Global - ADC.vi" "ADC"() -> (w2173:T18)
                    n1020 = Replace Array Subset(array=w2173, new element=w2171, index=w2176) -> (w2172:T18)
                    n1021 = global write "Global - ADC.vi" "ADC"(w2172) -> ()
                  }
                  frame "Read PID" {
                    n1022 = Unbundle By Name(w2180) -> ("PID"=w2177:T19)
                    n1023 = global read "Global - PID.vi" "PID"() -> (w2179:T20)
                    n1024 = Replace Array Subset(array=w2179, new element=w2177, index=w2182) -> (w2178:T20)
                    n1025 = global write "Global - PID.vi" "PID"(w2178) -> ()
                  }
                  frame "Read System" {
                    n1026 = Unbundle By Name(w2186) -> ("System"=w2184:T21)
                    n1027 = global read "Global - System.vi" "System"() -> (w2185:T22)
                    n1028 = Replace Array Subset(array=w2185, new element=w2184, index=w2188) -> (w2183:T22)
                    n1029 = global write "Global - System.vi" "System"(w2183) -> ()
                  }
                  frame "Read Test" {
                    n1030 = Unbundle By Name(w2192) -> ("Test"=w2189:T23)
                    n1031 = global read "Global - Test.vi" "Test"() -> (w2190:T24)
                    n1032 = Replace Array Subset(array=w2190, new element=w2189, index=w2194) -> (w2191:T24)
                    n1033 = global write "Global - Test.vi" "Test"(w2191) -> ()
                  }
                }
              }
            }
          }
          frame "Close" {
          }
        }
      }
      frame Error {
        n1034 = global read "Global - IP Address.vi" "IP"() -> (w2207:string[])
        n1035 = Unbundle By Name(w2208) -> ("source"=w2203:string)
        n1036 = Index Array(array=w2207, index=0) -> (element=w2205:string)
        n1037 = Concatenate Strings(w2205, " - " ("string"), w2203) -> (w2199:string)
        n1038 = call <vilib>:"Clear Errors.vi"("error in (no error)"=w2208) -> ("error out"=w2202:errorcluster)  [unwired: 5 in, 1 out]
        n1039 = call "General - Error Log eFGV.vi"("eFGV States"=eFGV_States."Write", "error in (no error)"=w2202, "Error In"=w2199) -> ("error out"=w2201:errorcluster)  [unwired: 6 in, 2 out]
        n1040 = Wait (ms)(milliseconds to wait=u32 100) -> ()  [unwired: 1 out]
      }
    }
  }
  n1041 = local write "Stop"(FALSE ("Stop")) -> ()
  n1042 = while {
    shift-right: [w2219] -> _
    shift-left: errorcluster {"status"=FALSE, "code"=0, "source"=""} ("error IO") -> [w2220]
    shift-right: [w2217] -> _
    shift-left: Communications_-_State."Init" -> [w2218]
    shift-right: [w2216] -> _
    shift-left: _ -> [w2215]
    shift-right: [w2213] -> _
    shift-left: _ -> [w2212]
    stop <- w2214 stop-if-true
    # "UI Loop"
    n1043 = case shown="No Error" w2220 {
      selector: w2220 -> [w2228 w2389]
      tunnel: [w2229 w2390] -> w2219
      tunnel: w2218 -> [w2227 _]
      tunnel: [w2226 Communications_-_State."Idle"] -> w2217
      tunnel: [w2225 w2395] -> w2216
      tunnel: w2215 -> [w2224 w2395]
      tunnel: [w2223 _] -> w2214
      tunnel: [w2222 w2394] -> w2213
      tunnel: w2212 -> [w2221 w2394]
      frame No Error {
        n1044 = case shown="\"Get IP Address\"" w2227 {
          tunnel: [w2230 w2248 w2267 w2343 w2371 w2376] -> w2229
          tunnel: w2228 -> [w2234 w2247 w2278 w2346 w2370 w2375]
          tunnel: [Communications_-_State."Get IP Address" w2246 w2264 w2339 Communications_-_State."Idle" Communications_-_State."Close"] -> w2226
          tunnel: [w2237 w2244 w2281 w2347 w2373 w2380] -> w2225
          tunnel: w2224 -> [_ w2245 w2281 w2347 w2373 w2380]
          tunnel: [_ _ _ _ _ w2378] -> w2223
          tunnel: [T5 {"UDP CMD"={"IP"="", "CMD"=enum."Stop", "Port"="", "Datalog?"=FALSE, "Float"=0.0}, "UDP ref"=refnum, "Unit?"=FALSE, "Read Unit"=[], "Trig?"=FALSE, "UDP Info"=[], "UDP Conn ref"=refnum, "DataLogger"=[], "VISA Ref"=refnum, "Float"=0.0, "Data"={"Test"={"Target Load"=0.0, "Target Disp"=0.0, "Rate"=0.0, "Speed"=0.0}, "Sensor"={"Name"=[], "Unit"=[], "Decimal Point"=[], "Ch Log"=[], "H Alarm"=[], "L Alarm"=[], "H Limit"=[], "L Limit"=[], "Filter"=[], "Gain"=[], "Calib Type"=[]}, "PID"={"SP"=0.0, "PV"=0.0, "kP"=0.0, "kI"=0.0, "kD"=0.0, "FF"=0.0, "Err Band"=0.0, "Max"=0, "Min"=0, "Ts"=0, "Out"=0, "Mode"=0}, "ADC"={"Active Ch"=[], "Filter Type"=0, "Post Filter"=[], "Gain"=[], "FS"=0, "IntOC"=0, "IntFC"=0, "SysOC"=0, "Cofficient"=[], "K"=[], "Max"=0}, "System"={"Out Type"=0, "Inverse"=0, "Monitor"=0, "Reserve"=0, "ACC Time"=0, "Pulse Rev"=0, "Stroke"=0, "Auto Off"=0, "Gear Ratio"=0.0, "Pitch"=0.0, "Max Speed"=0, "Jog Speed"=0, "Disp Coff"=0.0, "Max Load"=0}, "Index"=enum."Ch1", "Datalog"=enum."Empty"}} w2243 w2268 w2338 w2367 w2377] -> w2222
          tunnel: w2221 -> [_ w2242 w2261 w2338 w2366 w2377]
          frame "Init", Default {
            w2233 = eFGV_States."Read" ("Action")
            n1045 = call "Communication - Trigger Read IP Address(FGV).vi"("Action"=w2233, "error in"=w2234) -> ("error out"=w2235:errorcluster, "Trigger ref"=w2232:refnum<user-event>)  [unwired: 7 in, 1 out]
            n1046 = call "General - Exit eFGV.vi"("eFGV States"=w2233, "error in (no error)"=w2235) -> ("error out"=w2239:errorcluster, "Exit"=w2238:refnum<user-event>)  [unwired: 7 in, 1 out]
            n1047 = register-events(error in=w2239, w2238, w2232) -> (reference out=w2237:refnum<event-registration>, error out=w2230:errorcluster)  [unwired: 1 in]
            n1048 = global write "Global - Hold.vi" "Hold"(FALSE ("Hold")) -> ()
          }
          frame "Idle" {
            n1049 = event shown="[0] Timeout" {
              selector: w2245 -> [_ _ _]
              dyn-events: [_ _ _] -> w2244
              timeout: 1000 -> [_ _ _]
              tunnel: [w2251 w2256 w2259] -> w2248
              tunnel: w2247 -> [w2251 w2256 w2259]
              tunnel: [Communications_-_State."Get IP Address" Communications_-_State."Get IP Address" Communications_-_State."Close"] -> w2246
              tunnel: [w2249 w2254 w2257] -> w2243
              tunnel: w2242 -> [w2249 w2253 w2257]
              event Timeout {
                n1050 = event-data() -> ()  [unwired: 1 in, 3 out]
              }
              event User Event {
                n1051 = event-data() -> ()  [unwired: 1 in, 1 out]
                n1052 = Bundle By Name(cluster=w2253, "Trig?"=TRUE) -> (w2254:T5)
              }
              event User Event {
                n1053 = event-data() -> ()  [unwired: 1 in, 5 out]
              }
            }
          }
          frame "Get IP Address" {
            n1054 = global read "Global - Comport.vi" "Port"() -> (w2270:string[])
            n1055 = global read "Global - IP Address.vi" "IP"() -> (w2274:string[])
            n1056 = global read "Global - Handle.vi" "Handle"() -> (w2273:T7)
            n1057 = global read "Global - Device.vi" "Device"() -> (w2272:string[])
            n1058 = call "Machine - Config File.vi"("Action"=enum16{"Write", "Read", "Read All", "Remove"}."Read All", "error in (no error)"=w2278) -> ("error out"=w2279:errorcluster, "Value Out"=w2266:cluster{"IP":string, "Key Value":string[]}[])  [unwired: 8 in]
            n1059 = Empty Array?(array=w2266) -> (empty?=w2263:bool)
            n1060 = for {
              tunnel: w2279 -> [w2299]
              tunnel: [w2300] -> w2267
              tunnel: [w2293] -> w2277 mode=indexing if=w2287
              tunnel: [w2284] -> w2276 mode=indexing if=w2287
              tunnel: w2266 -> [w2298] mode=indexing
              tunnel: [w2296] -> w2275 mode=indexing if=w2287
              tunnel: w2274 -> [w2292]
              tunnel: w2273 -> [w2286]
              tunnel: w2272 -> [w2291]
              tunnel: [w2290] -> w2271 mode=indexing if=w2287
              tunnel: w2270 -> [w2289]
              tunnel: [w2288] -> w2269 mode=indexing if=w2287
              shift-right: [w2282] -> w2260
              shift-left: w2261 -> [w2283]
              n1061 = Unbundle By Name(w2298) -> ("IP"=w2295:string, "Key Value"=w2297:string[])
              n1062 = Search 1D Array(1D array=w2292, element=w2295) -> (index of element=w2285:i32)  [unwired: 1 in]
              n1063 = Greater Or Equal To 0?(x=w2285) -> (x >= 0?=w2294:bool)
              n1064 = case shown="True" w2294 {
                tunnel: [w2305 w2325] -> w2300
                tunnel: w2299 -> [w2319 w2327]
                tunnel: w2297 -> [w2321 _]
                tunnel: [w2320 w2334] -> w2296
                tunnel: [w2307 w2326] -> w2284
                tunnel: [w2315 w2324] -> w2287
                tunnel: w2295 -> [w2313 _]
                tunnel: [w2313 w2329] -> w2293
                tunnel: w2292 -> [_ w2337]
                tunnel: w2285 -> [_ w2333]
                tunnel: w2286 -> [_ w2336]
                tunnel: w2291 -> [_ w2335]
                tunnel: [w2312 w2331] -> w2290
                tunnel: w2289 -> [_ w2332]
                tunnel: [w2315 FALSE] -> w2288
                tunnel: w2283 -> [w2302 w2323]
                tunnel: [w2301 w2323] -> w2282
                frame False {
                  n1065 = Index Array(array=w2321) -> (element #1=w2312:string, element #2=w2320:string)  [unwired: 2 in]
                  n1066 = Bundle By Name(cluster=T8 {"IP Address"="192.168.88.49", "port"="", "UDP ref"=refnum} ("UDP Info"), "IP Address"=w2313, "port"=w2312) -> (w2303:T8)
                  n1067 = call "UDP - Open Connection.vi"(7:w2302, "error in"=w2319, "UDP Info"=w2303) -> ("error out"=w2310:errorcluster, "UDP Info Out"=w2308:T8, 5:w2301:T5)  [unwired: 6 in]
                  n1068 = call "UDP - Write CMD.vi"("CMD"=UDP_-_Command."Read Sensor", "error in"=w2310, "UDP Info"=w2308) -> ("error out"=w2309:errorcluster, "UDP Info Out"=w2307:T8, "Success"=w2306:bool)  [unwired: 3 in, 3 out]
                  n1069 = Empty String/Path?(string/path=w2313) -> (empty?=w2322:bool)
                  n1070 = Empty String/Path?(string/path=w2312) -> (empty?=w2318:bool)
                  n1071 = call <vilib>:"Clear Errors.vi"("error in (no error)"=w2309, "specific error code to clear (0: all)"=56) -> ("error out"=w2305:errorcluster)  [unwired: 4 in, 1 out]
                  n1072 = Not(x=w2322) -> (.not. x?=w2317:bool)
                  n1073 = Not(x=w2318) -> (.not. x?=w2316:bool)
                  n1074 = Compound Arithmetic op=AND(w2317, w2316, w2306) -> (w2315:bool)
                }
                frame True {
                  n1075 = Index Array(array=w2335, index=w2333) -> (element=w2334:string)
                  n1076 = Index Array(array=w2337, index=w2333) -> (element=w2329:string)
                  n1077 = Index Array(array=w2336, index=w2333) -> (element=w2326:T8)
                  n1078 = Index Array(array=w2332, index=w2333) -> (element=w2331:string)
                  n1079 = call "UDP - Write CMD.vi"("CMD"=UDP_-_Command."Read Sensor", "error in"=w2327, "UDP Info"=w2326) -> ("error out"=w2325:errorcluster, "Success"=w2324:bool)  [unwired: 3 in, 4 out]
                }
              }
            }
            "IP" <- w2277
            "Device" <- w2275
            n1080 = global write "Global - Handle.vi" "Handle"(w2276) -> ()
            n1081 = global write "Global - Device.vi" "Device"(w2275) -> ()
            n1082 = global write "Global - IP Address.vi" "IP"(w2277) -> ()
            n1083 = global write "Global - Comport.vi" "Port"(w2271) -> ()
            n1084 = Bundle By Name(cluster=w2260, "Read Unit"=w2269) -> (w2268:T5)
            n1085 = Select(t=Communications_-_State."Release Rendezvous", s=w2263, f=Communications_-_State."Command") -> (s? t:f=w2264:T1)
          }
          frame "Command" {
            n1086 = Unbundle By Name(w2338) -> ("Trig?"=w2342:bool, "Read Unit"=w2344:bool[])
            n1087 = global read "Global - Handle.vi" "Handle"() -> (w2345:T7)
            n1088 = for {
              shift-right: [w2350] -> w2343
              shift-left: w2346 -> [w2352]
              tunnel: w2345 -> [w2349] mode=indexing
              tunnel: w2344 -> [w2348] mode=indexing
              i -> [w2351]
              n1089 = case shown="True" w2348 {
                tunnel: w2352 -> [w2353 w2360]
                tunnel: w2351 -> [_ w2359]
                tunnel: [w2353 w2358] -> w2350
                tunnel: w2349 -> [_ w2354]
                frame False {
                }
                frame True {
                  n1090 = call "UDP - Write CMD.vi"("CMD"=UDP_-_Command."Read Sensor", "error in"=w2360, "UDP Info"=w2354) -> ("error out"=w2358:errorcluster, "Data Out"=w2357:T11, "Success"=w2356:bool)  [unwired: 3 in, 3 out]
                  n1091 = case shown="True" w2356 {
                    tunnel: w2359 -> [_ w2365]
                    tunnel: w2357 -> [_ w2361]
                    frame False {
                    }
                    frame True {
                      n1092 = Unbundle By Name(w2361) -> ("Sensor"=w2362:T15)
                      n1093 = global read "Global - Unit.vi" "Unit"() -> (w2364:T16)
                      n1094 = Replace Array Subset(array=w2364, new element=w2362, index=w2365) -> (w2363:T16)
                      n1095 = global write "Global - Unit.vi" "Unit"(w2363) -> ()
                    }
                  }
                }
              }
            }
            n1096 = Select(t=Communications_-_State."Idle", s=w2342, f=Communications_-_State."Release Rendezvous") -> (s? t:f=w2339:T1)
          }
          frame "Release Rendezvous" {
            n1097 = global read "Global - Rendezvous.vi" "rendezvous"() -> (w2369:T25)
            n1098 = call <vilib>:"Wait at Rendezvous.vi"("error in (no error)"=w2370, "rendezvous"=w2369) -> ("error out"=w2371:errorcluster)  [unwired: 3 in, 2 out]
            n1099 = Bundle By Name(cluster=w2366, "Trig?"=TRUE) -> (w2367:T5)
          }
          frame "Close" {
            w2378 = TRUE
            n1100 = global read "Global - Handle.vi" "Handle"() -> (w2374:T7)
            n1101 = for {
              tunnel: w2374 -> [w2384] mode=indexing
              shift-right: [w2382] -> w2376
              shift-left: w2375 -> [w2383]
              n1102 = Unbundle By Name(w2384) -> ("UDP ref"=w2381:refnum<k16>)
              n1103 = UDP Close(connection ID=w2381, 8:w2383) -> (error out=w2382:errorcluster)  [unwired: 1 out]
            }
            "Stop" <- w2378
          }
        }
      }
      frame Error {
        n1104 = Unbundle By Name(w2389) -> ("source"=w2387:string)
        n1105 = Concatenate Strings("UI Loop (Comm)" ("string"), " - " ("string"), w2387) -> (w2385:string)
        n1106 = Wait (ms)(milliseconds to wait=u32 100) -> ()  [unwired: 1 out]
        n1107 = call <vilib>:"Clear Errors.vi"("error in (no error)"=w2389) -> ("error out"=w2391:errorcluster)  [unwired: 5 in, 1 out]
        n1108 = call "General - Error Log eFGV.vi"("eFGV States"=eFGV_States."Write", "error in (no error)"=w2391, "Error In"=w2385) -> ("error out"=w2390:errorcluster)  [unwired: 6 in, 2 out]
      }
    }
  }
  n1109 = while {
    shift-right: [w2402] -> _
    shift-left: errorcluster {"status"=FALSE, "code"=0, "source"=""} ("error IO") -> [w2403]
    shift-right: [w2400] -> _
    shift-left: Communications_-_State."Init" -> [w2401]
    shift-right: [w2398] -> _
    shift-left: _ -> [w2397]
    stop <- w2399 stop-if-true
    # "Command Processing Loop"
    n1110 = case shown="No Error" w2403 {
      selector: w2403 -> [w2409 w2527]
      tunnel: [w2410 w2520] -> w2402
      tunnel: w2401 -> [w2408 _]
      tunnel: [w2407 Communications_-_State."Idle"] -> w2400
      tunnel: [w2406 _] -> w2399
      tunnel: [w2405 w2529] -> w2398
      tunnel: w2397 -> [w2404 w2529]
      frame No Error {
        n1111 = case shown="\"Idle\"" w2408 {
          tunnel: [w2413 w2427 w2461 w2517] -> w2410
          tunnel: w2409 -> [w2418 w2426 w2464 w2517]
          tunnel: [Communications_-_State."Idle" w2421 Communications_-_State."Idle" Communications_-_State."Close"] -> w2407
          tunnel: [_ _ _ TRUE] -> w2406
          tunnel: [w2415 w2425 w2463 w2514] -> w2405
          tunnel: w2404 -> [_ w2424 w2463 w2514]
          frame "Init", Default {
            n1112 = call "Communication - UDP Command (eFGV).vi"("Action"=eFGV_States."Read", "error in"=w2418) -> ("error out"=w2414:errorcluster, "UDP Ref"=w2412:refnum<user-event>)  [unwired: 7 in, 1 out]
            n1113 = register-events(error in=w2414, w2412) -> (reference out=w2411:refnum<event-registration>, error out=w2413:errorcluster)  [unwired: 1 in]
            n1114 = Bundle By Name(cluster=T5 {"UDP CMD"={"IP"="", "CMD"=enum."Stop", "Port"="", "Datalog?"=FALSE, "Float"=0.0}, "UDP ref"=refnum, "Unit?"=FALSE, "Read Unit"=[], "Trig?"=FALSE, "UDP Info"=[], "UDP Conn ref"=refnum, "DataLogger"=[], "VISA Ref"=refnum, "Float"=0.0, "Data"={"Test"={"Target Load"=0.0, "Target Disp"=0.0, "Rate"=0.0, "Speed"=0.0}, "Sensor"={"Name"=[], "Unit"=[], "Decimal Point"=[], "Ch Log"=[], "H Alarm"=[], "L Alarm"=[], "H Limit"=[], "L Limit"=[], "Filter"=[], "Gain"=[], "Calib Type"=[]}, "PID"={"SP"=0.0, "PV"=0.0, "kP"=0.0, "kI"=0.0, "kD"=0.0, "FF"=0.0, "Err Band"=0.0, "Max"=0, "Min"=0, "Ts"=0, "Out"=0, "Mode"=0}, "ADC"={"Active Ch"=[], "Filter Type"=0, "Post Filter"=[], "Gain"=[], "FS"=0, "IntOC"=0, "IntFC"=0, "SysOC"=0, "Cofficient"=[], "K"=[], "Max"=0}, "System"={"Out Type"=0, "Inverse"=0, "Monitor"=0, "Reserve"=0, "ACC Time"=0, "Pulse Rev"=0, "Stroke"=0, "Auto Off"=0, "Gear Ratio"=0.0, "Pitch"=0.0, "Max Speed"=0, "Jog Speed"=0, "Disp Coff"=0.0, "Max Load"=0}, "Index"=enum."Ch1", "Datalog"=enum."Empty"}}, "UDP ref"=w2411) -> (w2415:T5)
          }
          frame "Idle" {
            n1115 = Unbundle By Name(w2424) -> ("UDP ref"=w2428:refnum<event-registration>)
            n1116 = event shown="[1] <FDTI ref>: User Event" {
              selector: w2428 -> [_ _]
              dyn-events: _ -> [_ _]
              timeout: _ -> [_ _]
              tunnel: [w2434 w2436] -> w2422
              tunnel: [w2431 _] -> w2427
              tunnel: w2426 -> [w2431 _]
              tunnel: [w2429 w2446] -> w2425
              tunnel: w2424 -> [w2429 w2445]
              event Timeout {
                n1117 = event-data() -> ()  [unwired: 1 in, 1 out]
                n1118 = local read "Stop"() -> (w2433:bool)
                n1119 = Select(t=Communications_-_State."Close", s=w2433, f=Communications_-_State."Idle") -> (s? t:f=w2434:T1)
              }
              event User Event {
                n1120 = event-data() -> ("IP"=w2439:string, "CMD"=w2444:T3, "Data"=w2443:T6)  [unwired: 1 in]
                n1121 = global read "Global - IP Address.vi" "IP"() -> (w2442:string[])
                n1122 = Index Array(array=w2442, index=29) -> (element=w2440:string)
                n1123 = Equal?(x=w2440, y=w2439) -> (x = y?=w2438:bool)
                n1124 = Bundle By Name(cluster=w2445, "UDP CMD.IP"=w2439, "UDP CMD.CMD"=w2444, "Data"=w2443) -> (w2446:T5)
                n1125 = Select(t=Communications_-_State."Command" ("f"), s=w2438, f=Communications_-_State."Idle") -> (s? t:f=w2436:T1)
              }
            }
            n1126 = global read "Global - Hold.vi" "Hold"() -> (w2423:bool)
            n1127 = Select(t=Communications_-_State."Idle", s=w2423, f=w2422) -> (s? t:f=w2421:T1)
          }
          frame "Command" {
            (unwired) UDP_-_Command."Stop" ("Enum")
            (unwired) 20
            n1128 = Unbundle By Name(w2463) -> ("UDP CMD.CMD"=w2460:T3, "Data"=w2462:T6, "UDP CMD.IP"=w2457:string)
            n1129 = global read "Global - Handle.vi" "Handle"() -> (w2452:T7)
            n1130 = global read "Global - IP Address.vi" "IP"() -> (w2450:string[])
            n1131 = Search 1D Array(1D array=w2450, element=w2457) -> (index of element=w2448:i32)  [unwired: 1 in]
            n1132 = Index Array(array=w2452, index=w2448) -> (element=w2456:T8)
            n1133 = call "UDP - Write CMD.vi"("CMD"=w2460, "error in"=w2464, "Data"=w2462, "UDP Info"=w2456) -> ("error out"=w2454:errorcluster, "IP Address"=w2449:string, "Data Out"=w2459:T11, "Success"=w2458:bool)  [unwired: 2 in, 2 out]
            n1134 = Wait (ms)(milliseconds to wait=u32 5) -> ()  [unwired: 1 out]
            n1135 = Search 1D Array(1D array=w2450, element=w2449) -> (index of element=w2447:i32)  [unwired: 1 in]
            n1136 = global read "Global - Done.vi" "Done"() -> (w2455:bool[])
            n1137 = Replace Array Subset(array=w2455, new element=w2458, index=w2447) -> (w2453:bool[])
            n1138 = global write "Global - Done.vi" "Done"(w2453) -> ()
            n1139 = case shown="True" w2458 {
              tunnel: w2454 -> [w2466 w2472]
              tunnel: [w2467 w2471] -> w2461
              tunnel: w2460 -> [_ w2473]
              tunnel: w2459 -> [_ w2470]
              tunnel: w2447 -> [_ w2469]
              frame False {
                n1140 = call "Communication - Trigger Read IP Address(FGV).vi"("Action"=eFGV_States."Write", "error in"=w2466) -> ("error out"=w2467:errorcluster)  [unwired: 7 in, 2 out]
              }
              frame True {
                n1141 = case shown="\"Read Ch Data\"" w2473 {
                  tunnel: w2472 -> [w2474 w2481 w2488 w2494 w2500 w2506 w2512]
                  tunnel: [w2474 w2481 w2488 w2494 w2500 w2506 w2512] -> w2471
                  tunnel: w2470 -> [_ w2479 w2485 w2493 w2499 w2505 w2511]
                  tunnel: w2469 -> [_ w2483 w2489 w2495 w2501 w2507 w2513]
                  frame "Stop", Default {
                  }
                  frame "Read Ch Data" {
                    n1142 = Unbundle By Name(w2479) -> ("Channels"=w2478:T12, "Event"=w2477:T10, "Status"=w2476:T9)
                    n1143 = global read "Global - Channel.vi" "Data"() -> (w2482:T13)
                    n1144 = Bundle("Channels"=w2478, "Event"=w2477, "Status"=w2476) -> (w2475:T14)  [unwired: 1 in]
                    n1145 = Replace Array Subset(array=w2482, new element=w2475, index=w2483) -> (w2480:T13)
                    n1146 = global write "Global - Channel.vi" "Data"(w2480) -> ()
                  }
                  frame "Read Sensor" {
                    n1147 = Unbundle By Name(w2485) -> ("Sensor"=w2484:T15)
                    n1148 = global read "Global - Unit.vi" "Unit"() -> (w2486:T16)
                    n1149 = Replace Array Subset(array=w2486, new element=w2484, index=w2489) -> (w2487:T16)
                    n1150 = global write "Global - Unit.vi" "Unit"(w2487) -> ()
                  }
                  frame "Read ADC" {
                    n1151 = Unbundle By Name(w2493) -> ("ADC"=w2490:T17)
                    n1152 = global read "Global - ADC.vi" "ADC"() -> (w2492:T18)
                    n1153 = Replace Array Subset(array=w2492, new element=w2490, index=w2495) -> (w2491:T18)
                    n1154 = global write "Global - ADC.vi" "ADC"(w2491) -> ()
                  }
                  frame "Read PID" {
                    n1155 = Unbundle By Name(w2499) -> ("PID"=w2496:T19)
                    n1156 = global read "Global - PID.vi" "PID"() -> (w2498:T20)
                    n1157 = Replace Array Subset(array=w2498, new element=w2496, index=w2501) -> (w2497:T20)
                    n1158 = global write "Global - PID.vi" "PID"(w2497) -> ()
                  }
                  frame "Read System" {
                    n1159 = Unbundle By Name(w2505) -> ("System"=w2503:T21)
                    n1160 = global read "Global - System.vi" "System"() -> (w2504:T22)
                    n1161 = Replace Array Subset(array=w2504, new element=w2503, index=w2507) -> (w2502:T22)
                    n1162 = global write "Global - System.vi" "System"(w2502) -> ()
                  }
                  frame "Read Test" {
                    n1163 = Unbundle By Name(w2511) -> ("Test"=w2508:T23)
                    n1164 = global read "Global - Test.vi" "Test"() -> (w2509:T24)
                    n1165 = Replace Array Subset(array=w2509, new element=w2508, index=w2513) -> (w2510:T24)
                    n1166 = global write "Global - Test.vi" "Test"(w2510) -> ()
                  }
                }
              }
            }
          }
          frame "Close" {
          }
        }
      }
      frame Error {
        n1167 = global read "Global - IP Address.vi" "IP"() -> (w2526:string[])
        n1168 = Unbundle By Name(w2527) -> ("source"=w2522:string)
        n1169 = Index Array(array=w2526, index=0) -> (element=w2524:string)
        n1170 = Concatenate Strings(w2524, " - " ("string"), w2522) -> (w2518:string)
        n1171 = call <vilib>:"Clear Errors.vi"("error in (no error)"=w2527) -> ("error out"=w2521:errorcluster)  [unwired: 5 in, 1 out]
        n1172 = call "General - Error Log eFGV.vi"("eFGV States"=eFGV_States."Write", "error in (no error)"=w2521, "Error In"=w2518) -> ("error out"=w2520:errorcluster)  [unwired: 6 in, 2 out]
        n1173 = Wait (ms)(milliseconds to wait=u32 100) -> ()  [unwired: 1 out]
      }
    }
  }
  n1174 = while {
    shift-right: [w2536] -> _
    shift-left: errorcluster {"status"=FALSE, "code"=0, "source"=""} ("error IO") -> [w2537]
    shift-right: [w2534] -> _
    shift-left: Communications_-_State."Init" -> [w2535]
    shift-right: [w2532] -> _
    shift-left: _ -> [w2531]
    stop <- w2533 stop-if-true
    # "Command Processing Loop"
    n1175 = case shown="No Error" w2537 {
      selector: w2537 -> [w2543 w2661]
      tunnel: [w2544 w2654] -> w2536
      tunnel: w2535 -> [w2542 _]
      tunnel: [w2541 Communications_-_State."Idle"] -> w2534
      tunnel: [w2540 _] -> w2533
      tunnel: [w2539 w2663] -> w2532
      tunnel: w2531 -> [w2538 w2663]
      frame No Error {
        n1176 = case shown="\"Idle\"" w2542 {
          tunnel: [w2547 w2561 w2595 w2651] -> w2544
          tunnel: w2543 -> [w2552 w2560 w2598 w2651]
          tunnel: [Communications_-_State."Idle" w2555 Communications_-_State."Idle" Communications_-_State."Close"] -> w2541
          tunnel: [_ _ _ TRUE] -> w2540
          tunnel: [w2549 w2559 w2597 w2648] -> w2539
          tunnel: w2538 -> [_ w2558 w2597 w2648]
          frame "Init", Default {
            n1177 = call "Communication - UDP Command (eFGV).vi"("Action"=eFGV_States."Read", "error in"=w2552) -> ("error out"=w2548:errorcluster, "UDP Ref"=w2546:refnum<user-event>)  [unwired: 7 in, 1 out]
            n1178 = register-events(error in=w2548, w2546) -> (reference out=w2545:refnum<event-registration>, error out=w2547:errorcluster)  [unwired: 1 in]
            n1179 = Bundle By Name(cluster=T5 {"UDP CMD"={"IP"="", "CMD"=enum."Stop", "Port"="", "Datalog?"=FALSE, "Float"=0.0}, "UDP ref"=refnum, "Unit?"=FALSE, "Read Unit"=[], "Trig?"=FALSE, "UDP Info"=[], "UDP Conn ref"=refnum, "DataLogger"=[], "VISA Ref"=refnum, "Float"=0.0, "Data"={"Test"={"Target Load"=0.0, "Target Disp"=0.0, "Rate"=0.0, "Speed"=0.0}, "Sensor"={"Name"=[], "Unit"=[], "Decimal Point"=[], "Ch Log"=[], "H Alarm"=[], "L Alarm"=[], "H Limit"=[], "L Limit"=[], "Filter"=[], "Gain"=[], "Calib Type"=[]}, "PID"={"SP"=0.0, "PV"=0.0, "kP"=0.0, "kI"=0.0, "kD"=0.0, "FF"=0.0, "Err Band"=0.0, "Max"=0, "Min"=0, "Ts"=0, "Out"=0, "Mode"=0}, "ADC"={"Active Ch"=[], "Filter Type"=0, "Post Filter"=[], "Gain"=[], "FS"=0, "IntOC"=0, "IntFC"=0, "SysOC"=0, "Cofficient"=[], "K"=[], "Max"=0}, "System"={"Out Type"=0, "Inverse"=0, "Monitor"=0, "Reserve"=0, "ACC Time"=0, "Pulse Rev"=0, "Stroke"=0, "Auto Off"=0, "Gear Ratio"=0.0, "Pitch"=0.0, "Max Speed"=0, "Jog Speed"=0, "Disp Coff"=0.0, "Max Load"=0}, "Index"=enum."Ch1", "Datalog"=enum."Empty"}}, "UDP ref"=w2545) -> (w2549:T5)
          }
          frame "Idle" {
            n1180 = Unbundle By Name(w2558) -> ("UDP ref"=w2562:refnum<event-registration>)
            n1181 = event shown="[1] <FDTI ref>: User Event" {
              selector: w2562 -> [_ _]
              dyn-events: _ -> [_ _]
              timeout: _ -> [_ _]
              tunnel: [w2568 w2570] -> w2556
              tunnel: [w2565 _] -> w2561
              tunnel: w2560 -> [w2565 _]
              tunnel: [w2563 w2580] -> w2559
              tunnel: w2558 -> [w2563 w2579]
              event Timeout {
                n1182 = event-data() -> ()  [unwired: 1 in, 1 out]
                n1183 = local read "Stop"() -> (w2567:bool)
                n1184 = Select(t=Communications_-_State."Close", s=w2567, f=Communications_-_State."Idle") -> (s? t:f=w2568:T1)
              }
              event User Event {
                n1185 = event-data() -> ("IP"=w2573:string, "CMD"=w2578:T3, "Data"=w2577:T6)  [unwired: 1 in]
                n1186 = global read "Global - IP Address.vi" "IP"() -> (w2576:string[])
                n1187 = Index Array(array=w2576, index=31) -> (element=w2574:string)
                n1188 = Equal?(x=w2574, y=w2573) -> (x = y?=w2572:bool)
                n1189 = Bundle By Name(cluster=w2579, "UDP CMD.IP"=w2573, "UDP CMD.CMD"=w2578, "Data"=w2577) -> (w2580:T5)
                n1190 = Select(t=Communications_-_State."Command" ("f"), s=w2572, f=Communications_-_State."Idle") -> (s? t:f=w2570:T1)
              }
            }
            n1191 = global read "Global - Hold.vi" "Hold"() -> (w2557:bool)
            n1192 = Select(t=Communications_-_State."Idle", s=w2557, f=w2556) -> (s? t:f=w2555:T1)
          }
          frame "Command" {
            (unwired) UDP_-_Command."Stop" ("Enum")
            (unwired) 20
            n1193 = Unbundle By Name(w2597) -> ("UDP CMD.CMD"=w2594:T3, "Data"=w2596:T6, "UDP CMD.IP"=w2591:string)
            n1194 = global read "Global - Handle.vi" "Handle"() -> (w2586:T7)
            n1195 = global read "Global - IP Address.vi" "IP"() -> (w2584:string[])
            n1196 = Search 1D Array(1D array=w2584, element=w2591) -> (index of element=w2582:i32)  [unwired: 1 in]
            n1197 = Index Array(array=w2586, index=w2582) -> (element=w2590:T8)
            n1198 = call "UDP - Write CMD.vi"("CMD"=w2594, "error in"=w2598, "Data"=w2596, "UDP Info"=w2590) -> ("error out"=w2588:errorcluster, "IP Address"=w2583:string, "Data Out"=w2593:T11, "Success"=w2592:bool)  [unwired: 2 in, 2 out]
            n1199 = Wait (ms)(milliseconds to wait=u32 5) -> ()  [unwired: 1 out]
            n1200 = Search 1D Array(1D array=w2584, element=w2583) -> (index of element=w2581:i32)  [unwired: 1 in]
            n1201 = global read "Global - Done.vi" "Done"() -> (w2589:bool[])
            n1202 = Replace Array Subset(array=w2589, new element=w2592, index=w2581) -> (w2587:bool[])
            n1203 = global write "Global - Done.vi" "Done"(w2587) -> ()
            n1204 = case shown="True" w2592 {
              tunnel: w2588 -> [w2600 w2606]
              tunnel: [w2601 w2605] -> w2595
              tunnel: w2594 -> [_ w2607]
              tunnel: w2593 -> [_ w2604]
              tunnel: w2581 -> [_ w2603]
              frame False {
                n1205 = call "Communication - Trigger Read IP Address(FGV).vi"("Action"=eFGV_States."Write", "error in"=w2600) -> ("error out"=w2601:errorcluster)  [unwired: 7 in, 2 out]
              }
              frame True {
                n1206 = case shown="\"Read Ch Data\"" w2607 {
                  tunnel: w2606 -> [w2608 w2615 w2622 w2628 w2634 w2640 w2646]
                  tunnel: [w2608 w2615 w2622 w2628 w2634 w2640 w2646] -> w2605
                  tunnel: w2604 -> [_ w2613 w2619 w2627 w2633 w2639 w2645]
                  tunnel: w2603 -> [_ w2617 w2623 w2629 w2635 w2641 w2647]
                  frame "Stop", Default {
                  }
                  frame "Read Ch Data" {
                    n1207 = Unbundle By Name(w2613) -> ("Channels"=w2612:T12, "Event"=w2611:T10, "Status"=w2610:T9)
                    n1208 = global read "Global - Channel.vi" "Data"() -> (w2616:T13)
                    n1209 = Bundle("Channels"=w2612, "Event"=w2611, "Status"=w2610) -> (w2609:T14)  [unwired: 1 in]
                    n1210 = Replace Array Subset(array=w2616, new element=w2609, index=w2617) -> (w2614:T13)
                    n1211 = global write "Global - Channel.vi" "Data"(w2614) -> ()
                  }
                  frame "Read Sensor" {
                    n1212 = Unbundle By Name(w2619) -> ("Sensor"=w2618:T15)
                    n1213 = global read "Global - Unit.vi" "Unit"() -> (w2620:T16)
                    n1214 = Replace Array Subset(array=w2620, new element=w2618, index=w2623) -> (w2621:T16)
                    n1215 = global write "Global - Unit.vi" "Unit"(w2621) -> ()
                  }
                  frame "Read ADC" {
                    n1216 = Unbundle By Name(w2627) -> ("ADC"=w2624:T17)
                    n1217 = global read "Global - ADC.vi" "ADC"() -> (w2626:T18)
                    n1218 = Replace Array Subset(array=w2626, new element=w2624, index=w2629) -> (w2625:T18)
                    n1219 = global write "Global - ADC.vi" "ADC"(w2625) -> ()
                  }
                  frame "Read PID" {
                    n1220 = Unbundle By Name(w2633) -> ("PID"=w2630:T19)
                    n1221 = global read "Global - PID.vi" "PID"() -> (w2632:T20)
                    n1222 = Replace Array Subset(array=w2632, new element=w2630, index=w2635) -> (w2631:T20)
                    n1223 = global write "Global - PID.vi" "PID"(w2631) -> ()
                  }
                  frame "Read System" {
                    n1224 = Unbundle By Name(w2639) -> ("System"=w2637:T21)
                    n1225 = global read "Global - System.vi" "System"() -> (w2638:T22)
                    n1226 = Replace Array Subset(array=w2638, new element=w2637, index=w2641) -> (w2636:T22)
                    n1227 = global write "Global - System.vi" "System"(w2636) -> ()
                  }
                  frame "Read Test" {
                    n1228 = Unbundle By Name(w2645) -> ("Test"=w2642:T23)
                    n1229 = global read "Global - Test.vi" "Test"() -> (w2643:T24)
                    n1230 = Replace Array Subset(array=w2643, new element=w2642, index=w2647) -> (w2644:T24)
                    n1231 = global write "Global - Test.vi" "Test"(w2644) -> ()
                  }
                }
              }
            }
          }
          frame "Close" {
          }
        }
      }
      frame Error {
        n1232 = global read "Global - IP Address.vi" "IP"() -> (w2660:string[])
        n1233 = Unbundle By Name(w2661) -> ("source"=w2656:string)
        n1234 = Index Array(array=w2660, index=0) -> (element=w2658:string)
        n1235 = Concatenate Strings(w2658, " - " ("string"), w2656) -> (w2652:string)
        n1236 = call <vilib>:"Clear Errors.vi"("error in (no error)"=w2661) -> ("error out"=w2655:errorcluster)  [unwired: 5 in, 1 out]
        n1237 = call "General - Error Log eFGV.vi"("eFGV States"=eFGV_States."Write", "error in (no error)"=w2655, "Error In"=w2652) -> ("error out"=w2654:errorcluster)  [unwired: 6 in, 2 out]
        n1238 = Wait (ms)(milliseconds to wait=u32 100) -> ()  [unwired: 1 out]
      }
    }
  }
  n1239 = while {
    shift-right: [w2670] -> _
    shift-left: errorcluster {"status"=FALSE, "code"=0, "source"=""} ("error IO") -> [w2671]
    shift-right: [w2668] -> _
    shift-left: Communications_-_State."Init" -> [w2669]
    shift-right: [w2666] -> _
    shift-left: _ -> [w2665]
    stop <- w2667 stop-if-true
    # "Command Processing Loop"
    n1240 = case shown="No Error" w2671 {
      selector: w2671 -> [w2677 w2795]
      tunnel: [w2678 w2788] -> w2670
      tunnel: w2669 -> [w2676 _]
      tunnel: [w2675 Communications_-_State."Idle"] -> w2668
      tunnel: [w2674 _] -> w2667
      tunnel: [w2673 w2797] -> w2666
      tunnel: w2665 -> [w2672 w2797]
      frame No Error {
        n1241 = case shown="\"Idle\"" w2676 {
          tunnel: [w2681 w2695 w2729 w2785] -> w2678
          tunnel: w2677 -> [w2686 w2694 w2732 w2785]
          tunnel: [Communications_-_State."Idle" w2689 Communications_-_State."Idle" Communications_-_State."Close"] -> w2675
          tunnel: [_ _ _ TRUE] -> w2674
          tunnel: [w2683 w2693 w2731 w2782] -> w2673
          tunnel: w2672 -> [_ w2692 w2731 w2782]
          frame "Init", Default {
            n1242 = call "Communication - UDP Command (eFGV).vi"("Action"=eFGV_States."Read", "error in"=w2686) -> ("error out"=w2682:errorcluster, "UDP Ref"=w2680:refnum<user-event>)  [unwired: 7 in, 1 out]
            n1243 = register-events(error in=w2682, w2680) -> (reference out=w2679:refnum<event-registration>, error out=w2681:errorcluster)  [unwired: 1 in]
            n1244 = Bundle By Name(cluster=T5 {"UDP CMD"={"IP"="", "CMD"=enum."Stop", "Port"="", "Datalog?"=FALSE, "Float"=0.0}, "UDP ref"=refnum, "Unit?"=FALSE, "Read Unit"=[], "Trig?"=FALSE, "UDP Info"=[], "UDP Conn ref"=refnum, "DataLogger"=[], "VISA Ref"=refnum, "Float"=0.0, "Data"={"Test"={"Target Load"=0.0, "Target Disp"=0.0, "Rate"=0.0, "Speed"=0.0}, "Sensor"={"Name"=[], "Unit"=[], "Decimal Point"=[], "Ch Log"=[], "H Alarm"=[], "L Alarm"=[], "H Limit"=[], "L Limit"=[], "Filter"=[], "Gain"=[], "Calib Type"=[]}, "PID"={"SP"=0.0, "PV"=0.0, "kP"=0.0, "kI"=0.0, "kD"=0.0, "FF"=0.0, "Err Band"=0.0, "Max"=0, "Min"=0, "Ts"=0, "Out"=0, "Mode"=0}, "ADC"={"Active Ch"=[], "Filter Type"=0, "Post Filter"=[], "Gain"=[], "FS"=0, "IntOC"=0, "IntFC"=0, "SysOC"=0, "Cofficient"=[], "K"=[], "Max"=0}, "System"={"Out Type"=0, "Inverse"=0, "Monitor"=0, "Reserve"=0, "ACC Time"=0, "Pulse Rev"=0, "Stroke"=0, "Auto Off"=0, "Gear Ratio"=0.0, "Pitch"=0.0, "Max Speed"=0, "Jog Speed"=0, "Disp Coff"=0.0, "Max Load"=0}, "Index"=enum."Ch1", "Datalog"=enum."Empty"}}, "UDP ref"=w2679) -> (w2683:T5)
          }
          frame "Idle" {
            n1245 = Unbundle By Name(w2692) -> ("UDP ref"=w2696:refnum<event-registration>)
            n1246 = event shown="[1] <FDTI ref>: User Event" {
              selector: w2696 -> [_ _]
              dyn-events: _ -> [_ _]
              timeout: _ -> [_ _]
              tunnel: [w2702 w2704] -> w2690
              tunnel: [w2699 _] -> w2695
              tunnel: w2694 -> [w2699 _]
              tunnel: [w2697 w2714] -> w2693
              tunnel: w2692 -> [w2697 w2713]
              event Timeout {
                n1247 = event-data() -> ()  [unwired: 1 in, 1 out]
                n1248 = local read "Stop"() -> (w2701:bool)
                n1249 = Select(t=Communications_-_State."Close", s=w2701, f=Communications_-_State."Idle") -> (s? t:f=w2702:T1)
              }
              event User Event {
                n1250 = event-data() -> ("IP"=w2707:string, "CMD"=w2712:T3, "Data"=w2711:T6)  [unwired: 1 in]
                n1251 = global read "Global - IP Address.vi" "IP"() -> (w2710:string[])
                n1252 = Index Array(array=w2710, index=25) -> (element=w2708:string)
                n1253 = Equal?(x=w2708, y=w2707) -> (x = y?=w2706:bool)
                n1254 = Bundle By Name(cluster=w2713, "UDP CMD.IP"=w2707, "UDP CMD.CMD"=w2712, "Data"=w2711) -> (w2714:T5)
                n1255 = Select(t=Communications_-_State."Command" ("f"), s=w2706, f=Communications_-_State."Idle") -> (s? t:f=w2704:T1)
              }
            }
            n1256 = global read "Global - Hold.vi" "Hold"() -> (w2691:bool)
            n1257 = Select(t=Communications_-_State."Idle", s=w2691, f=w2690) -> (s? t:f=w2689:T1)
          }
          frame "Command" {
            (unwired) UDP_-_Command."Stop" ("Enum")
            (unwired) 20
            n1258 = Unbundle By Name(w2731) -> ("UDP CMD.CMD"=w2728:T3, "Data"=w2730:T6, "UDP CMD.IP"=w2725:string)
            n1259 = global read "Global - Handle.vi" "Handle"() -> (w2720:T7)
            n1260 = global read "Global - IP Address.vi" "IP"() -> (w2718:string[])
            n1261 = Search 1D Array(1D array=w2718, element=w2725) -> (index of element=w2716:i32)  [unwired: 1 in]
            n1262 = Index Array(array=w2720, index=w2716) -> (element=w2724:T8)
            n1263 = call "UDP - Write CMD.vi"("CMD"=w2728, "error in"=w2732, "Data"=w2730, "UDP Info"=w2724) -> ("error out"=w2722:errorcluster, "IP Address"=w2717:string, "Data Out"=w2727:T11, "Success"=w2726:bool)  [unwired: 2 in, 2 out]
            n1264 = Wait (ms)(milliseconds to wait=u32 5) -> ()  [unwired: 1 out]
            n1265 = Search 1D Array(1D array=w2718, element=w2717) -> (index of element=w2715:i32)  [unwired: 1 in]
            n1266 = global read "Global - Done.vi" "Done"() -> (w2723:bool[])
            n1267 = Replace Array Subset(array=w2723, new element=w2726, index=w2715) -> (w2721:bool[])
            n1268 = global write "Global - Done.vi" "Done"(w2721) -> ()
            n1269 = case shown="True" w2726 {
              tunnel: w2722 -> [w2734 w2740]
              tunnel: [w2735 w2739] -> w2729
              tunnel: w2728 -> [_ w2741]
              tunnel: w2727 -> [_ w2738]
              tunnel: w2715 -> [_ w2737]
              frame False {
                n1270 = call "Communication - Trigger Read IP Address(FGV).vi"("Action"=eFGV_States."Write", "error in"=w2734) -> ("error out"=w2735:errorcluster)  [unwired: 7 in, 2 out]
              }
              frame True {
                n1271 = case shown="\"Read Ch Data\"" w2741 {
                  tunnel: w2740 -> [w2742 w2749 w2756 w2762 w2768 w2774 w2780]
                  tunnel: [w2742 w2749 w2756 w2762 w2768 w2774 w2780] -> w2739
                  tunnel: w2738 -> [_ w2747 w2753 w2761 w2767 w2773 w2779]
                  tunnel: w2737 -> [_ w2751 w2757 w2763 w2769 w2775 w2781]
                  frame "Stop", Default {
                  }
                  frame "Read Ch Data" {
                    n1272 = Unbundle By Name(w2747) -> ("Channels"=w2746:T12, "Event"=w2745:T10, "Status"=w2744:T9)
                    n1273 = global read "Global - Channel.vi" "Data"() -> (w2750:T13)
                    n1274 = Bundle("Channels"=w2746, "Event"=w2745, "Status"=w2744) -> (w2743:T14)  [unwired: 1 in]
                    n1275 = Replace Array Subset(array=w2750, new element=w2743, index=w2751) -> (w2748:T13)
                    n1276 = global write "Global - Channel.vi" "Data"(w2748) -> ()
                  }
                  frame "Read Sensor" {
                    n1277 = Unbundle By Name(w2753) -> ("Sensor"=w2752:T15)
                    n1278 = global read "Global - Unit.vi" "Unit"() -> (w2754:T16)
                    n1279 = Replace Array Subset(array=w2754, new element=w2752, index=w2757) -> (w2755:T16)
                    n1280 = global write "Global - Unit.vi" "Unit"(w2755) -> ()
                  }
                  frame "Read ADC" {
                    n1281 = Unbundle By Name(w2761) -> ("ADC"=w2758:T17)
                    n1282 = global read "Global - ADC.vi" "ADC"() -> (w2760:T18)
                    n1283 = Replace Array Subset(array=w2760, new element=w2758, index=w2763) -> (w2759:T18)
                    n1284 = global write "Global - ADC.vi" "ADC"(w2759) -> ()
                  }
                  frame "Read PID" {
                    n1285 = Unbundle By Name(w2767) -> ("PID"=w2764:T19)
                    n1286 = global read "Global - PID.vi" "PID"() -> (w2766:T20)
                    n1287 = Replace Array Subset(array=w2766, new element=w2764, index=w2769) -> (w2765:T20)
                    n1288 = global write "Global - PID.vi" "PID"(w2765) -> ()
                  }
                  frame "Read System" {
                    n1289 = Unbundle By Name(w2773) -> ("System"=w2771:T21)
                    n1290 = global read "Global - System.vi" "System"() -> (w2772:T22)
                    n1291 = Replace Array Subset(array=w2772, new element=w2771, index=w2775) -> (w2770:T22)
                    n1292 = global write "Global - System.vi" "System"(w2770) -> ()
                  }
                  frame "Read Test" {
                    n1293 = Unbundle By Name(w2779) -> ("Test"=w2776:T23)
                    n1294 = global read "Global - Test.vi" "Test"() -> (w2777:T24)
                    n1295 = Replace Array Subset(array=w2777, new element=w2776, index=w2781) -> (w2778:T24)
                    n1296 = global write "Global - Test.vi" "Test"(w2778) -> ()
                  }
                }
              }
            }
          }
          frame "Close" {
          }
        }
      }
      frame Error {
        n1297 = global read "Global - IP Address.vi" "IP"() -> (w2794:string[])
        n1298 = Unbundle By Name(w2795) -> ("source"=w2790:string)
        n1299 = Index Array(array=w2794, index=0) -> (element=w2792:string)
        n1300 = Concatenate Strings(w2792, " - " ("string"), w2790) -> (w2786:string)
        n1301 = call <vilib>:"Clear Errors.vi"("error in (no error)"=w2795) -> ("error out"=w2789:errorcluster)  [unwired: 5 in, 1 out]
        n1302 = call "General - Error Log eFGV.vi"("eFGV States"=eFGV_States."Write", "error in (no error)"=w2789, "Error In"=w2786) -> ("error out"=w2788:errorcluster)  [unwired: 6 in, 2 out]
        n1303 = Wait (ms)(milliseconds to wait=u32 100) -> ()  [unwired: 1 out]
      }
    }
  }
  n1304 = while {
    shift-right: [w2804] -> _
    shift-left: errorcluster {"status"=FALSE, "code"=0, "source"=""} ("error IO") -> [w2805]
    shift-right: [w2802] -> _
    shift-left: Communications_-_State."Init" -> [w2803]
    shift-right: [w2800] -> _
    shift-left: _ -> [w2799]
    stop <- w2801 stop-if-true
    # "Command Processing Loop"
    n1305 = case shown="No Error" w2805 {
      selector: w2805 -> [w2811 w2929]
      tunnel: [w2812 w2922] -> w2804
      tunnel: w2803 -> [w2810 _]
      tunnel: [w2809 Communications_-_State."Idle"] -> w2802
      tunnel: [w2808 _] -> w2801
      tunnel: [w2807 w2931] -> w2800
      tunnel: w2799 -> [w2806 w2931]
      frame No Error {
        n1306 = case shown="\"Idle\"" w2810 {
          tunnel: [w2815 w2829 w2863 w2919] -> w2812
          tunnel: w2811 -> [w2820 w2828 w2866 w2919]
          tunnel: [Communications_-_State."Idle" w2823 Communications_-_State."Idle" Communications_-_State."Close"] -> w2809
          tunnel: [_ _ _ TRUE] -> w2808
          tunnel: [w2817 w2827 w2865 w2916] -> w2807
          tunnel: w2806 -> [_ w2826 w2865 w2916]
          frame "Init", Default {
            n1307 = call "Communication - UDP Command (eFGV).vi"("Action"=eFGV_States."Read", "error in"=w2820) -> ("error out"=w2816:errorcluster, "UDP Ref"=w2814:refnum<user-event>)  [unwired: 7 in, 1 out]
            n1308 = register-events(error in=w2816, w2814) -> (reference out=w2813:refnum<event-registration>, error out=w2815:errorcluster)  [unwired: 1 in]
            n1309 = Bundle By Name(cluster=T5 {"UDP CMD"={"IP"="", "CMD"=enum."Stop", "Port"="", "Datalog?"=FALSE, "Float"=0.0}, "UDP ref"=refnum, "Unit?"=FALSE, "Read Unit"=[], "Trig?"=FALSE, "UDP Info"=[], "UDP Conn ref"=refnum, "DataLogger"=[], "VISA Ref"=refnum, "Float"=0.0, "Data"={"Test"={"Target Load"=0.0, "Target Disp"=0.0, "Rate"=0.0, "Speed"=0.0}, "Sensor"={"Name"=[], "Unit"=[], "Decimal Point"=[], "Ch Log"=[], "H Alarm"=[], "L Alarm"=[], "H Limit"=[], "L Limit"=[], "Filter"=[], "Gain"=[], "Calib Type"=[]}, "PID"={"SP"=0.0, "PV"=0.0, "kP"=0.0, "kI"=0.0, "kD"=0.0, "FF"=0.0, "Err Band"=0.0, "Max"=0, "Min"=0, "Ts"=0, "Out"=0, "Mode"=0}, "ADC"={"Active Ch"=[], "Filter Type"=0, "Post Filter"=[], "Gain"=[], "FS"=0, "IntOC"=0, "IntFC"=0, "SysOC"=0, "Cofficient"=[], "K"=[], "Max"=0}, "System"={"Out Type"=0, "Inverse"=0, "Monitor"=0, "Reserve"=0, "ACC Time"=0, "Pulse Rev"=0, "Stroke"=0, "Auto Off"=0, "Gear Ratio"=0.0, "Pitch"=0.0, "Max Speed"=0, "Jog Speed"=0, "Disp Coff"=0.0, "Max Load"=0}, "Index"=enum."Ch1", "Datalog"=enum."Empty"}}, "UDP ref"=w2813) -> (w2817:T5)
          }
          frame "Idle" {
            n1310 = Unbundle By Name(w2826) -> ("UDP ref"=w2830:refnum<event-registration>)
            n1311 = event shown="[1] <FDTI ref>: User Event" {
              selector: w2830 -> [_ _]
              dyn-events: _ -> [_ _]
              timeout: _ -> [_ _]
              tunnel: [w2836 w2838] -> w2824
              tunnel: [w2833 _] -> w2829
              tunnel: w2828 -> [w2833 _]
              tunnel: [w2831 w2848] -> w2827
              tunnel: w2826 -> [w2831 w2847]
              event Timeout {
                n1312 = event-data() -> ()  [unwired: 1 in, 1 out]
                n1313 = local read "Stop"() -> (w2835:bool)
                n1314 = Select(t=Communications_-_State."Close", s=w2835, f=Communications_-_State."Idle") -> (s? t:f=w2836:T1)
              }
              event User Event {
                n1315 = event-data() -> ("IP"=w2841:string, "CMD"=w2846:T3, "Data"=w2845:T6)  [unwired: 1 in]
                n1316 = global read "Global - IP Address.vi" "IP"() -> (w2844:string[])
                n1317 = Index Array(array=w2844, index=27) -> (element=w2842:string)
                n1318 = Equal?(x=w2842, y=w2841) -> (x = y?=w2840:bool)
                n1319 = Bundle By Name(cluster=w2847, "UDP CMD.IP"=w2841, "UDP CMD.CMD"=w2846, "Data"=w2845) -> (w2848:T5)
                n1320 = Select(t=Communications_-_State."Command" ("f"), s=w2840, f=Communications_-_State."Idle") -> (s? t:f=w2838:T1)
              }
            }
            n1321 = global read "Global - Hold.vi" "Hold"() -> (w2825:bool)
            n1322 = Select(t=Communications_-_State."Idle", s=w2825, f=w2824) -> (s? t:f=w2823:T1)
          }
          frame "Command" {
            (unwired) UDP_-_Command."Stop" ("Enum")
            (unwired) 20
            n1323 = Unbundle By Name(w2865) -> ("UDP CMD.CMD"=w2862:T3, "Data"=w2864:T6, "UDP CMD.IP"=w2859:string)
            n1324 = global read "Global - Handle.vi" "Handle"() -> (w2854:T7)
            n1325 = global read "Global - IP Address.vi" "IP"() -> (w2852:string[])
            n1326 = Search 1D Array(1D array=w2852, element=w2859) -> (index of element=w2850:i32)  [unwired: 1 in]
            n1327 = Index Array(array=w2854, index=w2850) -> (element=w2858:T8)
            n1328 = call "UDP - Write CMD.vi"("CMD"=w2862, "error in"=w2866, "Data"=w2864, "UDP Info"=w2858) -> ("error out"=w2856:errorcluster, "IP Address"=w2851:string, "Data Out"=w2861:T11, "Success"=w2860:bool)  [unwired: 2 in, 2 out]
            n1329 = Wait (ms)(milliseconds to wait=u32 5) -> ()  [unwired: 1 out]
            n1330 = Search 1D Array(1D array=w2852, element=w2851) -> (index of element=w2849:i32)  [unwired: 1 in]
            n1331 = global read "Global - Done.vi" "Done"() -> (w2857:bool[])
            n1332 = Replace Array Subset(array=w2857, new element=w2860, index=w2849) -> (w2855:bool[])
            n1333 = global write "Global - Done.vi" "Done"(w2855) -> ()
            n1334 = case shown="True" w2860 {
              tunnel: w2856 -> [w2868 w2874]
              tunnel: [w2869 w2873] -> w2863
              tunnel: w2862 -> [_ w2875]
              tunnel: w2861 -> [_ w2872]
              tunnel: w2849 -> [_ w2871]
              frame False {
                n1335 = call "Communication - Trigger Read IP Address(FGV).vi"("Action"=eFGV_States."Write", "error in"=w2868) -> ("error out"=w2869:errorcluster)  [unwired: 7 in, 2 out]
              }
              frame True {
                n1336 = case shown="\"Read Ch Data\"" w2875 {
                  tunnel: w2874 -> [w2876 w2883 w2890 w2896 w2902 w2908 w2914]
                  tunnel: [w2876 w2883 w2890 w2896 w2902 w2908 w2914] -> w2873
                  tunnel: w2872 -> [_ w2881 w2887 w2895 w2901 w2907 w2913]
                  tunnel: w2871 -> [_ w2885 w2891 w2897 w2903 w2909 w2915]
                  frame "Stop", Default {
                  }
                  frame "Read Ch Data" {
                    n1337 = Unbundle By Name(w2881) -> ("Channels"=w2880:T12, "Event"=w2879:T10, "Status"=w2878:T9)
                    n1338 = global read "Global - Channel.vi" "Data"() -> (w2884:T13)
                    n1339 = Bundle("Channels"=w2880, "Event"=w2879, "Status"=w2878) -> (w2877:T14)  [unwired: 1 in]
                    n1340 = Replace Array Subset(array=w2884, new element=w2877, index=w2885) -> (w2882:T13)
                    n1341 = global write "Global - Channel.vi" "Data"(w2882) -> ()
                  }
                  frame "Read Sensor" {
                    n1342 = Unbundle By Name(w2887) -> ("Sensor"=w2886:T15)
                    n1343 = global read "Global - Unit.vi" "Unit"() -> (w2888:T16)
                    n1344 = Replace Array Subset(array=w2888, new element=w2886, index=w2891) -> (w2889:T16)
                    n1345 = global write "Global - Unit.vi" "Unit"(w2889) -> ()
                  }
                  frame "Read ADC" {
                    n1346 = Unbundle By Name(w2895) -> ("ADC"=w2892:T17)
                    n1347 = global read "Global - ADC.vi" "ADC"() -> (w2894:T18)
                    n1348 = Replace Array Subset(array=w2894, new element=w2892, index=w2897) -> (w2893:T18)
                    n1349 = global write "Global - ADC.vi" "ADC"(w2893) -> ()
                  }
                  frame "Read PID" {
                    n1350 = Unbundle By Name(w2901) -> ("PID"=w2898:T19)
                    n1351 = global read "Global - PID.vi" "PID"() -> (w2900:T20)
                    n1352 = Replace Array Subset(array=w2900, new element=w2898, index=w2903) -> (w2899:T20)
                    n1353 = global write "Global - PID.vi" "PID"(w2899) -> ()
                  }
                  frame "Read System" {
                    n1354 = Unbundle By Name(w2907) -> ("System"=w2905:T21)
                    n1355 = global read "Global - System.vi" "System"() -> (w2906:T22)
                    n1356 = Replace Array Subset(array=w2906, new element=w2905, index=w2909) -> (w2904:T22)
                    n1357 = global write "Global - System.vi" "System"(w2904) -> ()
                  }
                  frame "Read Test" {
                    n1358 = Unbundle By Name(w2913) -> ("Test"=w2910:T23)
                    n1359 = global read "Global - Test.vi" "Test"() -> (w2911:T24)
                    n1360 = Replace Array Subset(array=w2911, new element=w2910, index=w2915) -> (w2912:T24)
                    n1361 = global write "Global - Test.vi" "Test"(w2912) -> ()
                  }
                }
              }
            }
          }
          frame "Close" {
          }
        }
      }
      frame Error {
        n1362 = global read "Global - IP Address.vi" "IP"() -> (w2928:string[])
        n1363 = Unbundle By Name(w2929) -> ("source"=w2924:string)
        n1364 = Index Array(array=w2928, index=0) -> (element=w2926:string)
        n1365 = Concatenate Strings(w2926, " - " ("string"), w2924) -> (w2920:string)
        n1366 = call <vilib>:"Clear Errors.vi"("error in (no error)"=w2929) -> ("error out"=w2923:errorcluster)  [unwired: 5 in, 1 out]
        n1367 = call "General - Error Log eFGV.vi"("eFGV States"=eFGV_States."Write", "error in (no error)"=w2923, "Error In"=w2920) -> ("error out"=w2922:errorcluster)  [unwired: 6 in, 2 out]
        n1368 = Wait (ms)(milliseconds to wait=u32 100) -> ()  [unwired: 1 out]
      }
    }
  }
  n1369 = while {
    shift-right: [w2938] -> _
    shift-left: errorcluster {"status"=FALSE, "code"=0, "source"=""} ("error IO") -> [w2939]
    shift-right: [w2936] -> _
    shift-left: Communications_-_State."Init" -> [w2937]
    shift-right: [w2934] -> _
    shift-left: _ -> [w2933]
    stop <- w2935 stop-if-true
    # "Command Processing Loop"
    n1370 = case shown="No Error" w2939 {
      selector: w2939 -> [w2945 w3063]
      tunnel: [w2946 w3056] -> w2938
      tunnel: w2937 -> [w2944 _]
      tunnel: [w2943 Communications_-_State."Idle"] -> w2936
      tunnel: [w2942 _] -> w2935
      tunnel: [w2941 w3065] -> w2934
      tunnel: w2933 -> [w2940 w3065]
      frame No Error {
        n1371 = case shown="\"Idle\"" w2944 {
          tunnel: [w2949 w2963 w2997 w3053] -> w2946
          tunnel: w2945 -> [w2954 w2962 w3000 w3053]
          tunnel: [Communications_-_State."Idle" w2957 Communications_-_State."Idle" Communications_-_State."Close"] -> w2943
          tunnel: [_ _ _ TRUE] -> w2942
          tunnel: [w2951 w2961 w2999 w3050] -> w2941
          tunnel: w2940 -> [_ w2960 w2999 w3050]
          frame "Init", Default {
            n1372 = call "Communication - UDP Command (eFGV).vi"("Action"=eFGV_States."Read", "error in"=w2954) -> ("error out"=w2950:errorcluster, "UDP Ref"=w2948:refnum<user-event>)  [unwired: 7 in, 1 out]
            n1373 = register-events(error in=w2950, w2948) -> (reference out=w2947:refnum<event-registration>, error out=w2949:errorcluster)  [unwired: 1 in]
            n1374 = Bundle By Name(cluster=T5 {"UDP CMD"={"IP"="", "CMD"=enum."Stop", "Port"="", "Datalog?"=FALSE, "Float"=0.0}, "UDP ref"=refnum, "Unit?"=FALSE, "Read Unit"=[], "Trig?"=FALSE, "UDP Info"=[], "UDP Conn ref"=refnum, "DataLogger"=[], "VISA Ref"=refnum, "Float"=0.0, "Data"={"Test"={"Target Load"=0.0, "Target Disp"=0.0, "Rate"=0.0, "Speed"=0.0}, "Sensor"={"Name"=[], "Unit"=[], "Decimal Point"=[], "Ch Log"=[], "H Alarm"=[], "L Alarm"=[], "H Limit"=[], "L Limit"=[], "Filter"=[], "Gain"=[], "Calib Type"=[]}, "PID"={"SP"=0.0, "PV"=0.0, "kP"=0.0, "kI"=0.0, "kD"=0.0, "FF"=0.0, "Err Band"=0.0, "Max"=0, "Min"=0, "Ts"=0, "Out"=0, "Mode"=0}, "ADC"={"Active Ch"=[], "Filter Type"=0, "Post Filter"=[], "Gain"=[], "FS"=0, "IntOC"=0, "IntFC"=0, "SysOC"=0, "Cofficient"=[], "K"=[], "Max"=0}, "System"={"Out Type"=0, "Inverse"=0, "Monitor"=0, "Reserve"=0, "ACC Time"=0, "Pulse Rev"=0, "Stroke"=0, "Auto Off"=0, "Gear Ratio"=0.0, "Pitch"=0.0, "Max Speed"=0, "Jog Speed"=0, "Disp Coff"=0.0, "Max Load"=0}, "Index"=enum."Ch1", "Datalog"=enum."Empty"}}, "UDP ref"=w2947) -> (w2951:T5)
          }
          frame "Idle" {
            n1375 = Unbundle By Name(w2960) -> ("UDP ref"=w2964:refnum<event-registration>)
            n1376 = event shown="[1] <FDTI ref>: User Event" {
              selector: w2964 -> [_ _]
              dyn-events: _ -> [_ _]
              timeout: _ -> [_ _]
              tunnel: [w2970 w2972] -> w2958
              tunnel: [w2967 _] -> w2963
              tunnel: w2962 -> [w2967 _]
              tunnel: [w2965 w2982] -> w2961
              tunnel: w2960 -> [w2965 w2981]
              event Timeout {
                n1377 = event-data() -> ()  [unwired: 1 in, 1 out]
                n1378 = local read "Stop"() -> (w2969:bool)
                n1379 = Select(t=Communications_-_State."Close", s=w2969, f=Communications_-_State."Idle") -> (s? t:f=w2970:T1)
              }
              event User Event {
                n1380 = event-data() -> ("IP"=w2975:string, "CMD"=w2980:T3, "Data"=w2979:T6)  [unwired: 1 in]
                n1381 = global read "Global - IP Address.vi" "IP"() -> (w2978:string[])
                n1382 = Index Array(array=w2978, index=13) -> (element=w2976:string)
                n1383 = Equal?(x=w2976, y=w2975) -> (x = y?=w2974:bool)
                n1384 = Bundle By Name(cluster=w2981, "UDP CMD.IP"=w2975, "UDP CMD.CMD"=w2980, "Data"=w2979) -> (w2982:T5)
                n1385 = Select(t=Communications_-_State."Command" ("f"), s=w2974, f=Communications_-_State."Idle") -> (s? t:f=w2972:T1)
              }
            }
            n1386 = global read "Global - Hold.vi" "Hold"() -> (w2959:bool)
            n1387 = Select(t=Communications_-_State."Idle", s=w2959, f=w2958) -> (s? t:f=w2957:T1)
          }
          frame "Command" {
            (unwired) UDP_-_Command."Stop" ("Enum")
            (unwired) 20
            n1388 = Unbundle By Name(w2999) -> ("UDP CMD.CMD"=w2996:T3, "Data"=w2998:T6, "UDP CMD.IP"=w2993:string)
            n1389 = global read "Global - Handle.vi" "Handle"() -> (w2988:T7)
            n1390 = global read "Global - IP Address.vi" "IP"() -> (w2986:string[])
            n1391 = Search 1D Array(1D array=w2986, element=w2993) -> (index of element=w2984:i32)  [unwired: 1 in]
            n1392 = Index Array(array=w2988, index=w2984) -> (element=w2992:T8)
            n1393 = call "UDP - Write CMD.vi"("CMD"=w2996, "error in"=w3000, "Data"=w2998, "UDP Info"=w2992) -> ("error out"=w2990:errorcluster, "IP Address"=w2985:string, "Data Out"=w2995:T11, "Success"=w2994:bool)  [unwired: 2 in, 2 out]
            n1394 = Wait (ms)(milliseconds to wait=u32 5) -> ()  [unwired: 1 out]
            n1395 = Search 1D Array(1D array=w2986, element=w2985) -> (index of element=w2983:i32)  [unwired: 1 in]
            n1396 = global read "Global - Done.vi" "Done"() -> (w2991:bool[])
            n1397 = Replace Array Subset(array=w2991, new element=w2994, index=w2983) -> (w2989:bool[])
            n1398 = global write "Global - Done.vi" "Done"(w2989) -> ()
            n1399 = case shown="True" w2994 {
              tunnel: w2990 -> [w3002 w3008]
              tunnel: [w3003 w3007] -> w2997
              tunnel: w2996 -> [_ w3009]
              tunnel: w2995 -> [_ w3006]
              tunnel: w2983 -> [_ w3005]
              frame False {
                n1400 = call "Communication - Trigger Read IP Address(FGV).vi"("Action"=eFGV_States."Write", "error in"=w3002) -> ("error out"=w3003:errorcluster)  [unwired: 7 in, 2 out]
              }
              frame True {
                n1401 = case shown="\"Read Ch Data\"" w3009 {
                  tunnel: w3008 -> [w3010 w3017 w3024 w3030 w3036 w3042 w3048]
                  tunnel: [w3010 w3017 w3024 w3030 w3036 w3042 w3048] -> w3007
                  tunnel: w3006 -> [_ w3015 w3021 w3029 w3035 w3041 w3047]
                  tunnel: w3005 -> [_ w3019 w3025 w3031 w3037 w3043 w3049]
                  frame "Stop", Default {
                  }
                  frame "Read Ch Data" {
                    n1402 = Unbundle By Name(w3015) -> ("Channels"=w3014:T12, "Event"=w3013:T10, "Status"=w3012:T9)
                    n1403 = global read "Global - Channel.vi" "Data"() -> (w3018:T13)
                    n1404 = Bundle("Channels"=w3014, "Event"=w3013, "Status"=w3012) -> (w3011:T14)  [unwired: 1 in]
                    n1405 = Replace Array Subset(array=w3018, new element=w3011, index=w3019) -> (w3016:T13)
                    n1406 = global write "Global - Channel.vi" "Data"(w3016) -> ()
                  }
                  frame "Read Sensor" {
                    n1407 = Unbundle By Name(w3021) -> ("Sensor"=w3020:T15)
                    n1408 = global read "Global - Unit.vi" "Unit"() -> (w3022:T16)
                    n1409 = Replace Array Subset(array=w3022, new element=w3020, index=w3025) -> (w3023:T16)
                    n1410 = global write "Global - Unit.vi" "Unit"(w3023) -> ()
                  }
                  frame "Read ADC" {
                    n1411 = Unbundle By Name(w3029) -> ("ADC"=w3026:T17)
                    n1412 = global read "Global - ADC.vi" "ADC"() -> (w3028:T18)
                    n1413 = Replace Array Subset(array=w3028, new element=w3026, index=w3031) -> (w3027:T18)
                    n1414 = global write "Global - ADC.vi" "ADC"(w3027) -> ()
                  }
                  frame "Read PID" {
                    n1415 = Unbundle By Name(w3035) -> ("PID"=w3032:T19)
                    n1416 = global read "Global - PID.vi" "PID"() -> (w3034:T20)
                    n1417 = Replace Array Subset(array=w3034, new element=w3032, index=w3037) -> (w3033:T20)
                    n1418 = global write "Global - PID.vi" "PID"(w3033) -> ()
                  }
                  frame "Read System" {
                    n1419 = Unbundle By Name(w3041) -> ("System"=w3039:T21)
                    n1420 = global read "Global - System.vi" "System"() -> (w3040:T22)
                    n1421 = Replace Array Subset(array=w3040, new element=w3039, index=w3043) -> (w3038:T22)
                    n1422 = global write "Global - System.vi" "System"(w3038) -> ()
                  }
                  frame "Read Test" {
                    n1423 = Unbundle By Name(w3047) -> ("Test"=w3044:T23)
                    n1424 = global read "Global - Test.vi" "Test"() -> (w3045:T24)
                    n1425 = Replace Array Subset(array=w3045, new element=w3044, index=w3049) -> (w3046:T24)
                    n1426 = global write "Global - Test.vi" "Test"(w3046) -> ()
                  }
                }
              }
            }
          }
          frame "Close" {
          }
        }
      }
      frame Error {
        n1427 = global read "Global - IP Address.vi" "IP"() -> (w3062:string[])
        n1428 = Unbundle By Name(w3063) -> ("source"=w3058:string)
        n1429 = Index Array(array=w3062, index=0) -> (element=w3060:string)
        n1430 = Concatenate Strings(w3060, " - " ("string"), w3058) -> (w3054:string)
        n1431 = call <vilib>:"Clear Errors.vi"("error in (no error)"=w3063) -> ("error out"=w3057:errorcluster)  [unwired: 5 in, 1 out]
        n1432 = call "General - Error Log eFGV.vi"("eFGV States"=eFGV_States."Write", "error in (no error)"=w3057, "Error In"=w3054) -> ("error out"=w3056:errorcluster)  [unwired: 6 in, 2 out]
        n1433 = Wait (ms)(milliseconds to wait=u32 100) -> ()  [unwired: 1 out]
      }
    }
  }
  n1434 = while {
    shift-right: [w3072] -> _
    shift-left: errorcluster {"status"=FALSE, "code"=0, "source"=""} ("error IO") -> [w3073]
    shift-right: [w3070] -> _
    shift-left: Communications_-_State."Init" -> [w3071]
    shift-right: [w3068] -> _
    shift-left: _ -> [w3067]
    stop <- w3069 stop-if-true
    # "Command Processing Loop"
    n1435 = case shown="No Error" w3073 {
      selector: w3073 -> [w3079 w3197]
      tunnel: [w3080 w3190] -> w3072
      tunnel: w3071 -> [w3078 _]
      tunnel: [w3077 Communications_-_State."Idle"] -> w3070
      tunnel: [w3076 _] -> w3069
      tunnel: [w3075 w3199] -> w3068
      tunnel: w3067 -> [w3074 w3199]
      frame No Error {
        n1436 = case shown="\"Idle\"" w3078 {
          tunnel: [w3083 w3097 w3131 w3187] -> w3080
          tunnel: w3079 -> [w3088 w3096 w3134 w3187]
          tunnel: [Communications_-_State."Idle" w3091 Communications_-_State."Idle" Communications_-_State."Close"] -> w3077
          tunnel: [_ _ _ TRUE] -> w3076
          tunnel: [w3085 w3095 w3133 w3184] -> w3075
          tunnel: w3074 -> [_ w3094 w3133 w3184]
          frame "Init", Default {
            n1437 = call "Communication - UDP Command (eFGV).vi"("Action"=eFGV_States."Read", "error in"=w3088) -> ("error out"=w3084:errorcluster, "UDP Ref"=w3082:refnum<user-event>)  [unwired: 7 in, 1 out]
            n1438 = register-events(error in=w3084, w3082) -> (reference out=w3081:refnum<event-registration>, error out=w3083:errorcluster)  [unwired: 1 in]
            n1439 = Bundle By Name(cluster=T5 {"UDP CMD"={"IP"="", "CMD"=enum."Stop", "Port"="", "Datalog?"=FALSE, "Float"=0.0}, "UDP ref"=refnum, "Unit?"=FALSE, "Read Unit"=[], "Trig?"=FALSE, "UDP Info"=[], "UDP Conn ref"=refnum, "DataLogger"=[], "VISA Ref"=refnum, "Float"=0.0, "Data"={"Test"={"Target Load"=0.0, "Target Disp"=0.0, "Rate"=0.0, "Speed"=0.0}, "Sensor"={"Name"=[], "Unit"=[], "Decimal Point"=[], "Ch Log"=[], "H Alarm"=[], "L Alarm"=[], "H Limit"=[], "L Limit"=[], "Filter"=[], "Gain"=[], "Calib Type"=[]}, "PID"={"SP"=0.0, "PV"=0.0, "kP"=0.0, "kI"=0.0, "kD"=0.0, "FF"=0.0, "Err Band"=0.0, "Max"=0, "Min"=0, "Ts"=0, "Out"=0, "Mode"=0}, "ADC"={"Active Ch"=[], "Filter Type"=0, "Post Filter"=[], "Gain"=[], "FS"=0, "IntOC"=0, "IntFC"=0, "SysOC"=0, "Cofficient"=[], "K"=[], "Max"=0}, "System"={"Out Type"=0, "Inverse"=0, "Monitor"=0, "Reserve"=0, "ACC Time"=0, "Pulse Rev"=0, "Stroke"=0, "Auto Off"=0, "Gear Ratio"=0.0, "Pitch"=0.0, "Max Speed"=0, "Jog Speed"=0, "Disp Coff"=0.0, "Max Load"=0}, "Index"=enum."Ch1", "Datalog"=enum."Empty"}}, "UDP ref"=w3081) -> (w3085:T5)
          }
          frame "Idle" {
            n1440 = Unbundle By Name(w3094) -> ("UDP ref"=w3098:refnum<event-registration>)
            n1441 = event shown="[1] <FDTI ref>: User Event" {
              selector: w3098 -> [_ _]
              dyn-events: _ -> [_ _]
              timeout: _ -> [_ _]
              tunnel: [w3104 w3106] -> w3092
              tunnel: [w3101 _] -> w3097
              tunnel: w3096 -> [w3101 _]
              tunnel: [w3099 w3116] -> w3095
              tunnel: w3094 -> [w3099 w3115]
              event Timeout {
                n1442 = event-data() -> ()  [unwired: 1 in, 1 out]
                n1443 = local read "Stop"() -> (w3103:bool)
                n1444 = Select(t=Communications_-_State."Close", s=w3103, f=Communications_-_State."Idle") -> (s? t:f=w3104:T1)
              }
              event User Event {
                n1445 = event-data() -> ("IP"=w3109:string, "CMD"=w3114:T3, "Data"=w3113:T6)  [unwired: 1 in]
                n1446 = global read "Global - IP Address.vi" "IP"() -> (w3112:string[])
                n1447 = Index Array(array=w3112, index=15) -> (element=w3110:string)
                n1448 = Equal?(x=w3110, y=w3109) -> (x = y?=w3108:bool)
                n1449 = Bundle By Name(cluster=w3115, "UDP CMD.IP"=w3109, "UDP CMD.CMD"=w3114, "Data"=w3113) -> (w3116:T5)
                n1450 = Select(t=Communications_-_State."Command" ("f"), s=w3108, f=Communications_-_State."Idle") -> (s? t:f=w3106:T1)
              }
            }
            n1451 = global read "Global - Hold.vi" "Hold"() -> (w3093:bool)
            n1452 = Select(t=Communications_-_State."Idle", s=w3093, f=w3092) -> (s? t:f=w3091:T1)
          }
          frame "Command" {
            (unwired) UDP_-_Command."Stop" ("Enum")
            (unwired) 20
            n1453 = Unbundle By Name(w3133) -> ("UDP CMD.CMD"=w3130:T3, "Data"=w3132:T6, "UDP CMD.IP"=w3127:string)
            n1454 = global read "Global - Handle.vi" "Handle"() -> (w3122:T7)
            n1455 = global read "Global - IP Address.vi" "IP"() -> (w3120:string[])
            n1456 = Search 1D Array(1D array=w3120, element=w3127) -> (index of element=w3118:i32)  [unwired: 1 in]
            n1457 = Index Array(array=w3122, index=w3118) -> (element=w3126:T8)
            n1458 = call "UDP - Write CMD.vi"("CMD"=w3130, "error in"=w3134, "Data"=w3132, "UDP Info"=w3126) -> ("error out"=w3124:errorcluster, "IP Address"=w3119:string, "Data Out"=w3129:T11, "Success"=w3128:bool)  [unwired: 2 in, 2 out]
            n1459 = Wait (ms)(milliseconds to wait=u32 5) -> ()  [unwired: 1 out]
            n1460 = Search 1D Array(1D array=w3120, element=w3119) -> (index of element=w3117:i32)  [unwired: 1 in]
            n1461 = global read "Global - Done.vi" "Done"() -> (w3125:bool[])
            n1462 = Replace Array Subset(array=w3125, new element=w3128, index=w3117) -> (w3123:bool[])
            n1463 = global write "Global - Done.vi" "Done"(w3123) -> ()
            n1464 = case shown="True" w3128 {
              tunnel: w3124 -> [w3136 w3142]
              tunnel: [w3137 w3141] -> w3131
              tunnel: w3130 -> [_ w3143]
              tunnel: w3129 -> [_ w3140]
              tunnel: w3117 -> [_ w3139]
              frame False {
                n1465 = call "Communication - Trigger Read IP Address(FGV).vi"("Action"=eFGV_States."Write", "error in"=w3136) -> ("error out"=w3137:errorcluster)  [unwired: 7 in, 2 out]
              }
              frame True {
                n1466 = case shown="\"Read Ch Data\"" w3143 {
                  tunnel: w3142 -> [w3144 w3151 w3158 w3164 w3170 w3176 w3182]
                  tunnel: [w3144 w3151 w3158 w3164 w3170 w3176 w3182] -> w3141
                  tunnel: w3140 -> [_ w3149 w3155 w3163 w3169 w3175 w3181]
                  tunnel: w3139 -> [_ w3153 w3159 w3165 w3171 w3177 w3183]
                  frame "Stop", Default {
                  }
                  frame "Read Ch Data" {
                    n1467 = Unbundle By Name(w3149) -> ("Channels"=w3148:T12, "Event"=w3147:T10, "Status"=w3146:T9)
                    n1468 = global read "Global - Channel.vi" "Data"() -> (w3152:T13)
                    n1469 = Bundle("Channels"=w3148, "Event"=w3147, "Status"=w3146) -> (w3145:T14)  [unwired: 1 in]
                    n1470 = Replace Array Subset(array=w3152, new element=w3145, index=w3153) -> (w3150:T13)
                    n1471 = global write "Global - Channel.vi" "Data"(w3150) -> ()
                  }
                  frame "Read Sensor" {
                    n1472 = Unbundle By Name(w3155) -> ("Sensor"=w3154:T15)
                    n1473 = global read "Global - Unit.vi" "Unit"() -> (w3156:T16)
                    n1474 = Replace Array Subset(array=w3156, new element=w3154, index=w3159) -> (w3157:T16)
                    n1475 = global write "Global - Unit.vi" "Unit"(w3157) -> ()
                  }
                  frame "Read ADC" {
                    n1476 = Unbundle By Name(w3163) -> ("ADC"=w3160:T17)
                    n1477 = global read "Global - ADC.vi" "ADC"() -> (w3162:T18)
                    n1478 = Replace Array Subset(array=w3162, new element=w3160, index=w3165) -> (w3161:T18)
                    n1479 = global write "Global - ADC.vi" "ADC"(w3161) -> ()
                  }
                  frame "Read PID" {
                    n1480 = Unbundle By Name(w3169) -> ("PID"=w3166:T19)
                    n1481 = global read "Global - PID.vi" "PID"() -> (w3168:T20)
                    n1482 = Replace Array Subset(array=w3168, new element=w3166, index=w3171) -> (w3167:T20)
                    n1483 = global write "Global - PID.vi" "PID"(w3167) -> ()
                  }
                  frame "Read System" {
                    n1484 = Unbundle By Name(w3175) -> ("System"=w3173:T21)
                    n1485 = global read "Global - System.vi" "System"() -> (w3174:T22)
                    n1486 = Replace Array Subset(array=w3174, new element=w3173, index=w3177) -> (w3172:T22)
                    n1487 = global write "Global - System.vi" "System"(w3172) -> ()
                  }
                  frame "Read Test" {
                    n1488 = Unbundle By Name(w3181) -> ("Test"=w3178:T23)
                    n1489 = global read "Global - Test.vi" "Test"() -> (w3179:T24)
                    n1490 = Replace Array Subset(array=w3179, new element=w3178, index=w3183) -> (w3180:T24)
                    n1491 = global write "Global - Test.vi" "Test"(w3180) -> ()
                  }
                }
              }
            }
          }
          frame "Close" {
          }
        }
      }
      frame Error {
        n1492 = global read "Global - IP Address.vi" "IP"() -> (w3196:string[])
        n1493 = Unbundle By Name(w3197) -> ("source"=w3192:string)
        n1494 = Index Array(array=w3196, index=0) -> (element=w3194:string)
        n1495 = Concatenate Strings(w3194, " - " ("string"), w3192) -> (w3188:string)
        n1496 = call <vilib>:"Clear Errors.vi"("error in (no error)"=w3197) -> ("error out"=w3191:errorcluster)  [unwired: 5 in, 1 out]
        n1497 = call "General - Error Log eFGV.vi"("eFGV States"=eFGV_States."Write", "error in (no error)"=w3191, "Error In"=w3188) -> ("error out"=w3190:errorcluster)  [unwired: 6 in, 2 out]
        n1498 = Wait (ms)(milliseconds to wait=u32 100) -> ()  [unwired: 1 out]
      }
    }
  }
  n1499 = while {
    shift-right: [w3206] -> _
    shift-left: errorcluster {"status"=FALSE, "code"=0, "source"=""} ("error IO") -> [w3207]
    shift-right: [w3204] -> _
    shift-left: Communications_-_State."Init" -> [w3205]
    shift-right: [w3202] -> _
    shift-left: _ -> [w3201]
    stop <- w3203 stop-if-true
    # "Command Processing Loop"
    n1500 = case shown="No Error" w3207 {
      selector: w3207 -> [w3213 w3331]
      tunnel: [w3214 w3324] -> w3206
      tunnel: w3205 -> [w3212 _]
      tunnel: [w3211 Communications_-_State."Idle"] -> w3204
      tunnel: [w3210 _] -> w3203
      tunnel: [w3209 w3333] -> w3202
      tunnel: w3201 -> [w3208 w3333]
      frame No Error {
        n1501 = case shown="\"Idle\"" w3212 {
          tunnel: [w3217 w3231 w3265 w3321] -> w3214
          tunnel: w3213 -> [w3222 w3230 w3268 w3321]
          tunnel: [Communications_-_State."Idle" w3225 Communications_-_State."Idle" Communications_-_State."Close"] -> w3211
          tunnel: [_ _ _ TRUE] -> w3210
          tunnel: [w3219 w3229 w3267 w3318] -> w3209
          tunnel: w3208 -> [_ w3228 w3267 w3318]
          frame "Init", Default {
            n1502 = call "Communication - UDP Command (eFGV).vi"("Action"=eFGV_States."Read", "error in"=w3222) -> ("error out"=w3218:errorcluster, "UDP Ref"=w3216:refnum<user-event>)  [unwired: 7 in, 1 out]
            n1503 = register-events(error in=w3218, w3216) -> (reference out=w3215:refnum<event-registration>, error out=w3217:errorcluster)  [unwired: 1 in]
            n1504 = Bundle By Name(cluster=T5 {"UDP CMD"={"IP"="", "CMD"=enum."Stop", "Port"="", "Datalog?"=FALSE, "Float"=0.0}, "UDP ref"=refnum, "Unit?"=FALSE, "Read Unit"=[], "Trig?"=FALSE, "UDP Info"=[], "UDP Conn ref"=refnum, "DataLogger"=[], "VISA Ref"=refnum, "Float"=0.0, "Data"={"Test"={"Target Load"=0.0, "Target Disp"=0.0, "Rate"=0.0, "Speed"=0.0}, "Sensor"={"Name"=[], "Unit"=[], "Decimal Point"=[], "Ch Log"=[], "H Alarm"=[], "L Alarm"=[], "H Limit"=[], "L Limit"=[], "Filter"=[], "Gain"=[], "Calib Type"=[]}, "PID"={"SP"=0.0, "PV"=0.0, "kP"=0.0, "kI"=0.0, "kD"=0.0, "FF"=0.0, "Err Band"=0.0, "Max"=0, "Min"=0, "Ts"=0, "Out"=0, "Mode"=0}, "ADC"={"Active Ch"=[], "Filter Type"=0, "Post Filter"=[], "Gain"=[], "FS"=0, "IntOC"=0, "IntFC"=0, "SysOC"=0, "Cofficient"=[], "K"=[], "Max"=0}, "System"={"Out Type"=0, "Inverse"=0, "Monitor"=0, "Reserve"=0, "ACC Time"=0, "Pulse Rev"=0, "Stroke"=0, "Auto Off"=0, "Gear Ratio"=0.0, "Pitch"=0.0, "Max Speed"=0, "Jog Speed"=0, "Disp Coff"=0.0, "Max Load"=0}, "Index"=enum."Ch1", "Datalog"=enum."Empty"}}, "UDP ref"=w3215) -> (w3219:T5)
          }
          frame "Idle" {
            n1505 = Unbundle By Name(w3228) -> ("UDP ref"=w3232:refnum<event-registration>)
            n1506 = event shown="[1] <FDTI ref>: User Event" {
              selector: w3232 -> [_ _]
              dyn-events: _ -> [_ _]
              timeout: _ -> [_ _]
              tunnel: [w3238 w3240] -> w3226
              tunnel: [w3235 _] -> w3231
              tunnel: w3230 -> [w3235 _]
              tunnel: [w3233 w3250] -> w3229
              tunnel: w3228 -> [w3233 w3249]
              event Timeout {
                n1507 = event-data() -> ()  [unwired: 1 in, 1 out]
                n1508 = local read "Stop"() -> (w3237:bool)
                n1509 = Select(t=Communications_-_State."Close", s=w3237, f=Communications_-_State."Idle") -> (s? t:f=w3238:T1)
              }
              event User Event {
                n1510 = event-data() -> ("IP"=w3243:string, "CMD"=w3248:T3, "Data"=w3247:T6)  [unwired: 1 in]
                n1511 = global read "Global - IP Address.vi" "IP"() -> (w3246:string[])
                n1512 = Index Array(array=w3246, index=21) -> (element=w3244:string)
                n1513 = Equal?(x=w3244, y=w3243) -> (x = y?=w3242:bool)
                n1514 = Bundle By Name(cluster=w3249, "UDP CMD.IP"=w3243, "UDP CMD.CMD"=w3248, "Data"=w3247) -> (w3250:T5)
                n1515 = Select(t=Communications_-_State."Command" ("f"), s=w3242, f=Communications_-_State."Idle") -> (s? t:f=w3240:T1)
              }
            }
            n1516 = global read "Global - Hold.vi" "Hold"() -> (w3227:bool)
            n1517 = Select(t=Communications_-_State."Idle", s=w3227, f=w3226) -> (s? t:f=w3225:T1)
          }
          frame "Command" {
            (unwired) UDP_-_Command."Stop" ("Enum")
            (unwired) 20
            n1518 = Unbundle By Name(w3267) -> ("UDP CMD.CMD"=w3264:T3, "Data"=w3266:T6, "UDP CMD.IP"=w3261:string)
            n1519 = global read "Global - Handle.vi" "Handle"() -> (w3256:T7)
            n1520 = global read "Global - IP Address.vi" "IP"() -> (w3254:string[])
            n1521 = Search 1D Array(1D array=w3254, element=w3261) -> (index of element=w3252:i32)  [unwired: 1 in]
            n1522 = Index Array(array=w3256, index=w3252) -> (element=w3260:T8)
            n1523 = call "UDP - Write CMD.vi"("CMD"=w3264, "error in"=w3268, "Data"=w3266, "UDP Info"=w3260) -> ("error out"=w3258:errorcluster, "IP Address"=w3253:string, "Data Out"=w3263:T11, "Success"=w3262:bool)  [unwired: 2 in, 2 out]
            n1524 = Wait (ms)(milliseconds to wait=u32 5) -> ()  [unwired: 1 out]
            n1525 = Search 1D Array(1D array=w3254, element=w3253) -> (index of element=w3251:i32)  [unwired: 1 in]
            n1526 = global read "Global - Done.vi" "Done"() -> (w3259:bool[])
            n1527 = Replace Array Subset(array=w3259, new element=w3262, index=w3251) -> (w3257:bool[])
            n1528 = global write "Global - Done.vi" "Done"(w3257) -> ()
            n1529 = case shown="True" w3262 {
              tunnel: w3258 -> [w3270 w3276]
              tunnel: [w3271 w3275] -> w3265
              tunnel: w3264 -> [_ w3277]
              tunnel: w3263 -> [_ w3274]
              tunnel: w3251 -> [_ w3273]
              frame False {
                n1530 = call "Communication - Trigger Read IP Address(FGV).vi"("Action"=eFGV_States."Write", "error in"=w3270) -> ("error out"=w3271:errorcluster)  [unwired: 7 in, 2 out]
              }
              frame True {
                n1531 = case shown="\"Read Ch Data\"" w3277 {
                  tunnel: w3276 -> [w3278 w3285 w3292 w3298 w3304 w3310 w3316]
                  tunnel: [w3278 w3285 w3292 w3298 w3304 w3310 w3316] -> w3275
                  tunnel: w3274 -> [_ w3283 w3289 w3297 w3303 w3309 w3315]
                  tunnel: w3273 -> [_ w3287 w3293 w3299 w3305 w3311 w3317]
                  frame "Stop", Default {
                  }
                  frame "Read Ch Data" {
                    n1532 = Unbundle By Name(w3283) -> ("Channels"=w3282:T12, "Event"=w3281:T10, "Status"=w3280:T9)
                    n1533 = global read "Global - Channel.vi" "Data"() -> (w3286:T13)
                    n1534 = Bundle("Channels"=w3282, "Event"=w3281, "Status"=w3280) -> (w3279:T14)  [unwired: 1 in]
                    n1535 = Replace Array Subset(array=w3286, new element=w3279, index=w3287) -> (w3284:T13)
                    n1536 = global write "Global - Channel.vi" "Data"(w3284) -> ()
                  }
                  frame "Read Sensor" {
                    n1537 = Unbundle By Name(w3289) -> ("Sensor"=w3288:T15)
                    n1538 = global read "Global - Unit.vi" "Unit"() -> (w3290:T16)
                    n1539 = Replace Array Subset(array=w3290, new element=w3288, index=w3293) -> (w3291:T16)
                    n1540 = global write "Global - Unit.vi" "Unit"(w3291) -> ()
                  }
                  frame "Read ADC" {
                    n1541 = Unbundle By Name(w3297) -> ("ADC"=w3294:T17)
                    n1542 = global read "Global - ADC.vi" "ADC"() -> (w3296:T18)
                    n1543 = Replace Array Subset(array=w3296, new element=w3294, index=w3299) -> (w3295:T18)
                    n1544 = global write "Global - ADC.vi" "ADC"(w3295) -> ()
                  }
                  frame "Read PID" {
                    n1545 = Unbundle By Name(w3303) -> ("PID"=w3300:T19)
                    n1546 = global read "Global - PID.vi" "PID"() -> (w3302:T20)
                    n1547 = Replace Array Subset(array=w3302, new element=w3300, index=w3305) -> (w3301:T20)
                    n1548 = global write "Global - PID.vi" "PID"(w3301) -> ()
                  }
                  frame "Read System" {
                    n1549 = Unbundle By Name(w3309) -> ("System"=w3307:T21)
                    n1550 = global read "Global - System.vi" "System"() -> (w3308:T22)
                    n1551 = Replace Array Subset(array=w3308, new element=w3307, index=w3311) -> (w3306:T22)
                    n1552 = global write "Global - System.vi" "System"(w3306) -> ()
                  }
                  frame "Read Test" {
                    n1553 = Unbundle By Name(w3315) -> ("Test"=w3312:T23)
                    n1554 = global read "Global - Test.vi" "Test"() -> (w3313:T24)
                    n1555 = Replace Array Subset(array=w3313, new element=w3312, index=w3317) -> (w3314:T24)
                    n1556 = global write "Global - Test.vi" "Test"(w3314) -> ()
                  }
                }
              }
            }
          }
          frame "Close" {
          }
        }
      }
      frame Error {
        n1557 = global read "Global - IP Address.vi" "IP"() -> (w3330:string[])
        n1558 = Unbundle By Name(w3331) -> ("source"=w3326:string)
        n1559 = Index Array(array=w3330, index=0) -> (element=w3328:string)
        n1560 = Concatenate Strings(w3328, " - " ("string"), w3326) -> (w3322:string)
        n1561 = call <vilib>:"Clear Errors.vi"("error in (no error)"=w3331) -> ("error out"=w3325:errorcluster)  [unwired: 5 in, 1 out]
        n1562 = call "General - Error Log eFGV.vi"("eFGV States"=eFGV_States."Write", "error in (no error)"=w3325, "Error In"=w3322) -> ("error out"=w3324:errorcluster)  [unwired: 6 in, 2 out]
        n1563 = Wait (ms)(milliseconds to wait=u32 100) -> ()  [unwired: 1 out]
      }
    }
  }
  n1564 = while {
    shift-right: [w3340] -> _
    shift-left: errorcluster {"status"=FALSE, "code"=0, "source"=""} ("error IO") -> [w3341]
    shift-right: [w3338] -> _
    shift-left: Communications_-_State."Init" -> [w3339]
    shift-right: [w3336] -> _
    shift-left: _ -> [w3335]
    stop <- w3337 stop-if-true
    # "Command Processing Loop"
    n1565 = case shown="No Error" w3341 {
      selector: w3341 -> [w3347 w3465]
      tunnel: [w3348 w3458] -> w3340
      tunnel: w3339 -> [w3346 _]
      tunnel: [w3345 Communications_-_State."Idle"] -> w3338
      tunnel: [w3344 _] -> w3337
      tunnel: [w3343 w3467] -> w3336
      tunnel: w3335 -> [w3342 w3467]
      frame No Error {
        n1566 = case shown="\"Idle\"" w3346 {
          tunnel: [w3351 w3365 w3399 w3455] -> w3348
          tunnel: w3347 -> [w3356 w3364 w3402 w3455]
          tunnel: [Communications_-_State."Idle" w3359 Communications_-_State."Idle" Communications_-_State."Close"] -> w3345
          tunnel: [_ _ _ TRUE] -> w3344
          tunnel: [w3353 w3363 w3401 w3452] -> w3343
          tunnel: w3342 -> [_ w3362 w3401 w3452]
          frame "Init", Default {
            n1567 = call "Communication - UDP Command (eFGV).vi"("Action"=eFGV_States."Read", "error in"=w3356) -> ("error out"=w3352:errorcluster, "UDP Ref"=w3350:refnum<user-event>)  [unwired: 7 in, 1 out]
            n1568 = register-events(error in=w3352, w3350) -> (reference out=w3349:refnum<event-registration>, error out=w3351:errorcluster)  [unwired: 1 in]
            n1569 = Bundle By Name(cluster=T5 {"UDP CMD"={"IP"="", "CMD"=enum."Stop", "Port"="", "Datalog?"=FALSE, "Float"=0.0}, "UDP ref"=refnum, "Unit?"=FALSE, "Read Unit"=[], "Trig?"=FALSE, "UDP Info"=[], "UDP Conn ref"=refnum, "DataLogger"=[], "VISA Ref"=refnum, "Float"=0.0, "Data"={"Test"={"Target Load"=0.0, "Target Disp"=0.0, "Rate"=0.0, "Speed"=0.0}, "Sensor"={"Name"=[], "Unit"=[], "Decimal Point"=[], "Ch Log"=[], "H Alarm"=[], "L Alarm"=[], "H Limit"=[], "L Limit"=[], "Filter"=[], "Gain"=[], "Calib Type"=[]}, "PID"={"SP"=0.0, "PV"=0.0, "kP"=0.0, "kI"=0.0, "kD"=0.0, "FF"=0.0, "Err Band"=0.0, "Max"=0, "Min"=0, "Ts"=0, "Out"=0, "Mode"=0}, "ADC"={"Active Ch"=[], "Filter Type"=0, "Post Filter"=[], "Gain"=[], "FS"=0, "IntOC"=0, "IntFC"=0, "SysOC"=0, "Cofficient"=[], "K"=[], "Max"=0}, "System"={"Out Type"=0, "Inverse"=0, "Monitor"=0, "Reserve"=0, "ACC Time"=0, "Pulse Rev"=0, "Stroke"=0, "Auto Off"=0, "Gear Ratio"=0.0, "Pitch"=0.0, "Max Speed"=0, "Jog Speed"=0, "Disp Coff"=0.0, "Max Load"=0}, "Index"=enum."Ch1", "Datalog"=enum."Empty"}}, "UDP ref"=w3349) -> (w3353:T5)
          }
          frame "Idle" {
            n1570 = Unbundle By Name(w3362) -> ("UDP ref"=w3366:refnum<event-registration>)
            n1571 = event shown="[1] <FDTI ref>: User Event" {
              selector: w3366 -> [_ _]
              dyn-events: _ -> [_ _]
              timeout: _ -> [_ _]
              tunnel: [w3372 w3374] -> w3360
              tunnel: [w3369 _] -> w3365
              tunnel: w3364 -> [w3369 _]
              tunnel: [w3367 w3384] -> w3363
              tunnel: w3362 -> [w3367 w3383]
              event Timeout {
                n1572 = event-data() -> ()  [unwired: 1 in, 1 out]
                n1573 = local read "Stop"() -> (w3371:bool)
                n1574 = Select(t=Communications_-_State."Close", s=w3371, f=Communications_-_State."Idle") -> (s? t:f=w3372:T1)
              }
              event User Event {
                n1575 = event-data() -> ("IP"=w3377:string, "CMD"=w3382:T3, "Data"=w3381:T6)  [unwired: 1 in]
                n1576 = global read "Global - IP Address.vi" "IP"() -> (w3380:string[])
                n1577 = Index Array(array=w3380, index=23) -> (element=w3378:string)
                n1578 = Equal?(x=w3378, y=w3377) -> (x = y?=w3376:bool)
                n1579 = Bundle By Name(cluster=w3383, "UDP CMD.IP"=w3377, "UDP CMD.CMD"=w3382, "Data"=w3381) -> (w3384:T5)
                n1580 = Select(t=Communications_-_State."Command" ("f"), s=w3376, f=Communications_-_State."Idle") -> (s? t:f=w3374:T1)
              }
            }
            n1581 = global read "Global - Hold.vi" "Hold"() -> (w3361:bool)
            n1582 = Select(t=Communications_-_State."Idle", s=w3361, f=w3360) -> (s? t:f=w3359:T1)
          }
          frame "Command" {
            (unwired) UDP_-_Command."Stop" ("Enum")
            (unwired) 20
            n1583 = Unbundle By Name(w3401) -> ("UDP CMD.CMD"=w3398:T3, "Data"=w3400:T6, "UDP CMD.IP"=w3395:string)
            n1584 = global read "Global - Handle.vi" "Handle"() -> (w3390:T7)
            n1585 = global read "Global - IP Address.vi" "IP"() -> (w3388:string[])
            n1586 = Search 1D Array(1D array=w3388, element=w3395) -> (index of element=w3386:i32)  [unwired: 1 in]
            n1587 = Index Array(array=w3390, index=w3386) -> (element=w3394:T8)
            n1588 = call "UDP - Write CMD.vi"("CMD"=w3398, "error in"=w3402, "Data"=w3400, "UDP Info"=w3394) -> ("error out"=w3392:errorcluster, "IP Address"=w3387:string, "Data Out"=w3397:T11, "Success"=w3396:bool)  [unwired: 2 in, 2 out]
            n1589 = Wait (ms)(milliseconds to wait=u32 5) -> ()  [unwired: 1 out]
            n1590 = Search 1D Array(1D array=w3388, element=w3387) -> (index of element=w3385:i32)  [unwired: 1 in]
            n1591 = global read "Global - Done.vi" "Done"() -> (w3393:bool[])
            n1592 = Replace Array Subset(array=w3393, new element=w3396, index=w3385) -> (w3391:bool[])
            n1593 = global write "Global - Done.vi" "Done"(w3391) -> ()
            n1594 = case shown="True" w3396 {
              tunnel: w3392 -> [w3404 w3410]
              tunnel: [w3405 w3409] -> w3399
              tunnel: w3398 -> [_ w3411]
              tunnel: w3397 -> [_ w3408]
              tunnel: w3385 -> [_ w3407]
              frame False {
                n1595 = call "Communication - Trigger Read IP Address(FGV).vi"("Action"=eFGV_States."Write", "error in"=w3404) -> ("error out"=w3405:errorcluster)  [unwired: 7 in, 2 out]
              }
              frame True {
                n1596 = case shown="\"Read Ch Data\"" w3411 {
                  tunnel: w3410 -> [w3412 w3419 w3426 w3432 w3438 w3444 w3450]
                  tunnel: [w3412 w3419 w3426 w3432 w3438 w3444 w3450] -> w3409
                  tunnel: w3408 -> [_ w3417 w3423 w3431 w3437 w3443 w3449]
                  tunnel: w3407 -> [_ w3421 w3427 w3433 w3439 w3445 w3451]
                  frame "Stop", Default {
                  }
                  frame "Read Ch Data" {
                    n1597 = Unbundle By Name(w3417) -> ("Channels"=w3416:T12, "Event"=w3415:T10, "Status"=w3414:T9)
                    n1598 = global read "Global - Channel.vi" "Data"() -> (w3420:T13)
                    n1599 = Bundle("Channels"=w3416, "Event"=w3415, "Status"=w3414) -> (w3413:T14)  [unwired: 1 in]
                    n1600 = Replace Array Subset(array=w3420, new element=w3413, index=w3421) -> (w3418:T13)
                    n1601 = global write "Global - Channel.vi" "Data"(w3418) -> ()
                  }
                  frame "Read Sensor" {
                    n1602 = Unbundle By Name(w3423) -> ("Sensor"=w3422:T15)
                    n1603 = global read "Global - Unit.vi" "Unit"() -> (w3424:T16)
                    n1604 = Replace Array Subset(array=w3424, new element=w3422, index=w3427) -> (w3425:T16)
                    n1605 = global write "Global - Unit.vi" "Unit"(w3425) -> ()
                  }
                  frame "Read ADC" {
                    n1606 = Unbundle By Name(w3431) -> ("ADC"=w3428:T17)
                    n1607 = global read "Global - ADC.vi" "ADC"() -> (w3430:T18)
                    n1608 = Replace Array Subset(array=w3430, new element=w3428, index=w3433) -> (w3429:T18)
                    n1609 = global write "Global - ADC.vi" "ADC"(w3429) -> ()
                  }
                  frame "Read PID" {
                    n1610 = Unbundle By Name(w3437) -> ("PID"=w3434:T19)
                    n1611 = global read "Global - PID.vi" "PID"() -> (w3436:T20)
                    n1612 = Replace Array Subset(array=w3436, new element=w3434, index=w3439) -> (w3435:T20)
                    n1613 = global write "Global - PID.vi" "PID"(w3435) -> ()
                  }
                  frame "Read System" {
                    n1614 = Unbundle By Name(w3443) -> ("System"=w3441:T21)
                    n1615 = global read "Global - System.vi" "System"() -> (w3442:T22)
                    n1616 = Replace Array Subset(array=w3442, new element=w3441, index=w3445) -> (w3440:T22)
                    n1617 = global write "Global - System.vi" "System"(w3440) -> ()
                  }
                  frame "Read Test" {
                    n1618 = Unbundle By Name(w3449) -> ("Test"=w3446:T23)
                    n1619 = global read "Global - Test.vi" "Test"() -> (w3447:T24)
                    n1620 = Replace Array Subset(array=w3447, new element=w3446, index=w3451) -> (w3448:T24)
                    n1621 = global write "Global - Test.vi" "Test"(w3448) -> ()
                  }
                }
              }
            }
          }
          frame "Close" {
          }
        }
      }
      frame Error {
        n1622 = global read "Global - IP Address.vi" "IP"() -> (w3464:string[])
        n1623 = Unbundle By Name(w3465) -> ("source"=w3460:string)
        n1624 = Index Array(array=w3464, index=0) -> (element=w3462:string)
        n1625 = Concatenate Strings(w3462, " - " ("string"), w3460) -> (w3456:string)
        n1626 = call <vilib>:"Clear Errors.vi"("error in (no error)"=w3465) -> ("error out"=w3459:errorcluster)  [unwired: 5 in, 1 out]
        n1627 = call "General - Error Log eFGV.vi"("eFGV States"=eFGV_States."Write", "error in (no error)"=w3459, "Error In"=w3456) -> ("error out"=w3458:errorcluster)  [unwired: 6 in, 2 out]
        n1628 = Wait (ms)(milliseconds to wait=u32 100) -> ()  [unwired: 1 out]
      }
    }
  }
  n1629 = while {
    shift-right: [w3474] -> _
    shift-left: errorcluster {"status"=FALSE, "code"=0, "source"=""} ("error IO") -> [w3475]
    shift-right: [w3472] -> _
    shift-left: Communications_-_State."Init" -> [w3473]
    shift-right: [w3470] -> _
    shift-left: _ -> [w3469]
    stop <- w3471 stop-if-true
    # "Command Processing Loop"
    n1630 = case shown="No Error" w3475 {
      selector: w3475 -> [w3481 w3599]
      tunnel: [w3482 w3592] -> w3474
      tunnel: w3473 -> [w3480 _]
      tunnel: [w3479 Communications_-_State."Idle"] -> w3472
      tunnel: [w3478 _] -> w3471
      tunnel: [w3477 w3601] -> w3470
      tunnel: w3469 -> [w3476 w3601]
      frame No Error {
        n1631 = case shown="\"Idle\"" w3480 {
          tunnel: [w3485 w3499 w3533 w3589] -> w3482
          tunnel: w3481 -> [w3490 w3498 w3536 w3589]
          tunnel: [Communications_-_State."Idle" w3493 Communications_-_State."Idle" Communications_-_State."Close"] -> w3479
          tunnel: [_ _ _ TRUE] -> w3478
          tunnel: [w3487 w3497 w3535 w3586] -> w3477
          tunnel: w3476 -> [_ w3496 w3535 w3586]
          frame "Init", Default {
            n1632 = call "Communication - UDP Command (eFGV).vi"("Action"=eFGV_States."Read", "error in"=w3490) -> ("error out"=w3486:errorcluster, "UDP Ref"=w3484:refnum<user-event>)  [unwired: 7 in, 1 out]
            n1633 = register-events(error in=w3486, w3484) -> (reference out=w3483:refnum<event-registration>, error out=w3485:errorcluster)  [unwired: 1 in]
            n1634 = Bundle By Name(cluster=T5 {"UDP CMD"={"IP"="", "CMD"=enum."Stop", "Port"="", "Datalog?"=FALSE, "Float"=0.0}, "UDP ref"=refnum, "Unit?"=FALSE, "Read Unit"=[], "Trig?"=FALSE, "UDP Info"=[], "UDP Conn ref"=refnum, "DataLogger"=[], "VISA Ref"=refnum, "Float"=0.0, "Data"={"Test"={"Target Load"=0.0, "Target Disp"=0.0, "Rate"=0.0, "Speed"=0.0}, "Sensor"={"Name"=[], "Unit"=[], "Decimal Point"=[], "Ch Log"=[], "H Alarm"=[], "L Alarm"=[], "H Limit"=[], "L Limit"=[], "Filter"=[], "Gain"=[], "Calib Type"=[]}, "PID"={"SP"=0.0, "PV"=0.0, "kP"=0.0, "kI"=0.0, "kD"=0.0, "FF"=0.0, "Err Band"=0.0, "Max"=0, "Min"=0, "Ts"=0, "Out"=0, "Mode"=0}, "ADC"={"Active Ch"=[], "Filter Type"=0, "Post Filter"=[], "Gain"=[], "FS"=0, "IntOC"=0, "IntFC"=0, "SysOC"=0, "Cofficient"=[], "K"=[], "Max"=0}, "System"={"Out Type"=0, "Inverse"=0, "Monitor"=0, "Reserve"=0, "ACC Time"=0, "Pulse Rev"=0, "Stroke"=0, "Auto Off"=0, "Gear Ratio"=0.0, "Pitch"=0.0, "Max Speed"=0, "Jog Speed"=0, "Disp Coff"=0.0, "Max Load"=0}, "Index"=enum."Ch1", "Datalog"=enum."Empty"}}, "UDP ref"=w3483) -> (w3487:T5)
          }
          frame "Idle" {
            n1635 = Unbundle By Name(w3496) -> ("UDP ref"=w3500:refnum<event-registration>)
            n1636 = event shown="[1] <FDTI ref>: User Event" {
              selector: w3500 -> [_ _]
              dyn-events: _ -> [_ _]
              timeout: _ -> [_ _]
              tunnel: [w3506 w3508] -> w3494
              tunnel: [w3503 _] -> w3499
              tunnel: w3498 -> [w3503 _]
              tunnel: [w3501 w3518] -> w3497
              tunnel: w3496 -> [w3501 w3517]
              event Timeout {
                n1637 = event-data() -> ()  [unwired: 1 in, 1 out]
                n1638 = local read "Stop"() -> (w3505:bool)
                n1639 = Select(t=Communications_-_State."Close", s=w3505, f=Communications_-_State."Idle") -> (s? t:f=w3506:T1)
              }
              event User Event {
                n1640 = event-data() -> ("IP"=w3511:string, "CMD"=w3516:T3, "Data"=w3515:T6)  [unwired: 1 in]
                n1641 = global read "Global - IP Address.vi" "IP"() -> (w3514:string[])
                n1642 = Index Array(array=w3514, index=9) -> (element=w3512:string)
                n1643 = Equal?(x=w3512, y=w3511) -> (x = y?=w3510:bool)
                n1644 = Bundle By Name(cluster=w3517, "UDP CMD.IP"=w3511, "UDP CMD.CMD"=w3516, "Data"=w3515) -> (w3518:T5)
                n1645 = Select(t=Communications_-_State."Command" ("f"), s=w3510, f=Communications_-_State."Idle") -> (s? t:f=w3508:T1)
              }
            }
            n1646 = global read "Global - Hold.vi" "Hold"() -> (w3495:bool)
            n1647 = Select(t=Communications_-_State."Idle", s=w3495, f=w3494) -> (s? t:f=w3493:T1)
          }
          frame "Command" {
            (unwired) UDP_-_Command."Stop" ("Enum")
            (unwired) 20
            n1648 = Unbundle By Name(w3535) -> ("UDP CMD.CMD"=w3532:T3, "Data"=w3534:T6, "UDP CMD.IP"=w3529:string)
            n1649 = global read "Global - Handle.vi" "Handle"() -> (w3524:T7)
            n1650 = global read "Global - IP Address.vi" "IP"() -> (w3522:string[])
            n1651 = Search 1D Array(1D array=w3522, element=w3529) -> (index of element=w3520:i32)  [unwired: 1 in]
            n1652 = Index Array(array=w3524, index=w3520) -> (element=w3528:T8)
            n1653 = call "UDP - Write CMD.vi"("CMD"=w3532, "error in"=w3536, "Data"=w3534, "UDP Info"=w3528) -> ("error out"=w3526:errorcluster, "IP Address"=w3521:string, "Data Out"=w3531:T11, "Success"=w3530:bool)  [unwired: 2 in, 2 out]
            n1654 = Wait (ms)(milliseconds to wait=u32 5) -> ()  [unwired: 1 out]
            n1655 = Search 1D Array(1D array=w3522, element=w3521) -> (index of element=w3519:i32)  [unwired: 1 in]
            n1656 = global read "Global - Done.vi" "Done"() -> (w3527:bool[])
            n1657 = Replace Array Subset(array=w3527, new element=w3530, index=w3519) -> (w3525:bool[])
            n1658 = global write "Global - Done.vi" "Done"(w3525) -> ()
            n1659 = case shown="True" w3530 {
              tunnel: w3526 -> [w3538 w3544]
              tunnel: [w3539 w3543] -> w3533
              tunnel: w3532 -> [_ w3545]
              tunnel: w3531 -> [_ w3542]
              tunnel: w3519 -> [_ w3541]
              frame False {
                n1660 = call "Communication - Trigger Read IP Address(FGV).vi"("Action"=eFGV_States."Write", "error in"=w3538) -> ("error out"=w3539:errorcluster)  [unwired: 7 in, 2 out]
              }
              frame True {
                n1661 = case shown="\"Read Ch Data\"" w3545 {
                  tunnel: w3544 -> [w3546 w3553 w3560 w3566 w3572 w3578 w3584]
                  tunnel: [w3546 w3553 w3560 w3566 w3572 w3578 w3584] -> w3543
                  tunnel: w3542 -> [_ w3551 w3557 w3565 w3571 w3577 w3583]
                  tunnel: w3541 -> [_ w3555 w3561 w3567 w3573 w3579 w3585]
                  frame "Stop", Default {
                  }
                  frame "Read Ch Data" {
                    n1662 = Unbundle By Name(w3551) -> ("Channels"=w3550:T12, "Event"=w3549:T10, "Status"=w3548:T9)
                    n1663 = global read "Global - Channel.vi" "Data"() -> (w3554:T13)
                    n1664 = Bundle("Channels"=w3550, "Event"=w3549, "Status"=w3548) -> (w3547:T14)  [unwired: 1 in]
                    n1665 = Replace Array Subset(array=w3554, new element=w3547, index=w3555) -> (w3552:T13)
                    n1666 = global write "Global - Channel.vi" "Data"(w3552) -> ()
                  }
                  frame "Read Sensor" {
                    n1667 = Unbundle By Name(w3557) -> ("Sensor"=w3556:T15)
                    n1668 = global read "Global - Unit.vi" "Unit"() -> (w3558:T16)
                    n1669 = Replace Array Subset(array=w3558, new element=w3556, index=w3561) -> (w3559:T16)
                    n1670 = global write "Global - Unit.vi" "Unit"(w3559) -> ()
                  }
                  frame "Read ADC" {
                    n1671 = Unbundle By Name(w3565) -> ("ADC"=w3562:T17)
                    n1672 = global read "Global - ADC.vi" "ADC"() -> (w3564:T18)
                    n1673 = Replace Array Subset(array=w3564, new element=w3562, index=w3567) -> (w3563:T18)
                    n1674 = global write "Global - ADC.vi" "ADC"(w3563) -> ()
                  }
                  frame "Read PID" {
                    n1675 = Unbundle By Name(w3571) -> ("PID"=w3568:T19)
                    n1676 = global read "Global - PID.vi" "PID"() -> (w3570:T20)
                    n1677 = Replace Array Subset(array=w3570, new element=w3568, index=w3573) -> (w3569:T20)
                    n1678 = global write "Global - PID.vi" "PID"(w3569) -> ()
                  }
                  frame "Read System" {
                    n1679 = Unbundle By Name(w3577) -> ("System"=w3575:T21)
                    n1680 = global read "Global - System.vi" "System"() -> (w3576:T22)
                    n1681 = Replace Array Subset(array=w3576, new element=w3575, index=w3579) -> (w3574:T22)
                    n1682 = global write "Global - System.vi" "System"(w3574) -> ()
                  }
                  frame "Read Test" {
                    n1683 = Unbundle By Name(w3583) -> ("Test"=w3580:T23)
                    n1684 = global read "Global - Test.vi" "Test"() -> (w3581:T24)
                    n1685 = Replace Array Subset(array=w3581, new element=w3580, index=w3585) -> (w3582:T24)
                    n1686 = global write "Global - Test.vi" "Test"(w3582) -> ()
                  }
                }
              }
            }
          }
          frame "Close" {
          }
        }
      }
      frame Error {
        n1687 = global read "Global - IP Address.vi" "IP"() -> (w3598:string[])
        n1688 = Unbundle By Name(w3599) -> ("source"=w3594:string)
        n1689 = Index Array(array=w3598, index=0) -> (element=w3596:string)
        n1690 = Concatenate Strings(w3596, " - " ("string"), w3594) -> (w3590:string)
        n1691 = call <vilib>:"Clear Errors.vi"("error in (no error)"=w3599) -> ("error out"=w3593:errorcluster)  [unwired: 5 in, 1 out]
        n1692 = call "General - Error Log eFGV.vi"("eFGV States"=eFGV_States."Write", "error in (no error)"=w3593, "Error In"=w3590) -> ("error out"=w3592:errorcluster)  [unwired: 6 in, 2 out]
        n1693 = Wait (ms)(milliseconds to wait=u32 100) -> ()  [unwired: 1 out]
      }
    }
  }
  n1694 = while {
    shift-right: [w3608] -> _
    shift-left: errorcluster {"status"=FALSE, "code"=0, "source"=""} ("error IO") -> [w3609]
    shift-right: [w3606] -> _
    shift-left: Communications_-_State."Init" -> [w3607]
    shift-right: [w3604] -> _
    shift-left: _ -> [w3603]
    stop <- w3605 stop-if-true
    # "Command Processing Loop"
    n1695 = case shown="No Error" w3609 {
      selector: w3609 -> [w3615 w3733]
      tunnel: [w3616 w3726] -> w3608
      tunnel: w3607 -> [w3614 _]
      tunnel: [w3613 Communications_-_State."Idle"] -> w3606
      tunnel: [w3612 _] -> w3605
      tunnel: [w3611 w3735] -> w3604
      tunnel: w3603 -> [w3610 w3735]
      frame No Error {
        n1696 = case shown="\"Idle\"" w3614 {
          tunnel: [w3619 w3633 w3667 w3723] -> w3616
          tunnel: w3615 -> [w3624 w3632 w3670 w3723]
          tunnel: [Communications_-_State."Idle" w3627 Communications_-_State."Idle" Communications_-_State."Close"] -> w3613
          tunnel: [_ _ _ TRUE] -> w3612
          tunnel: [w3621 w3631 w3669 w3720] -> w3611
          tunnel: w3610 -> [_ w3630 w3669 w3720]
          frame "Init", Default {
            n1697 = call "Communication - UDP Command (eFGV).vi"("Action"=eFGV_States."Read", "error in"=w3624) -> ("error out"=w3620:errorcluster, "UDP Ref"=w3618:refnum<user-event>)  [unwired: 7 in, 1 out]
            n1698 = register-events(error in=w3620, w3618) -> (reference out=w3617:refnum<event-registration>, error out=w3619:errorcluster)  [unwired: 1 in]
            n1699 = Bundle By Name(cluster=T5 {"UDP CMD"={"IP"="", "CMD"=enum."Stop", "Port"="", "Datalog?"=FALSE, "Float"=0.0}, "UDP ref"=refnum, "Unit?"=FALSE, "Read Unit"=[], "Trig?"=FALSE, "UDP Info"=[], "UDP Conn ref"=refnum, "DataLogger"=[], "VISA Ref"=refnum, "Float"=0.0, "Data"={"Test"={"Target Load"=0.0, "Target Disp"=0.0, "Rate"=0.0, "Speed"=0.0}, "Sensor"={"Name"=[], "Unit"=[], "Decimal Point"=[], "Ch Log"=[], "H Alarm"=[], "L Alarm"=[], "H Limit"=[], "L Limit"=[], "Filter"=[], "Gain"=[], "Calib Type"=[]}, "PID"={"SP"=0.0, "PV"=0.0, "kP"=0.0, "kI"=0.0, "kD"=0.0, "FF"=0.0, "Err Band"=0.0, "Max"=0, "Min"=0, "Ts"=0, "Out"=0, "Mode"=0}, "ADC"={"Active Ch"=[], "Filter Type"=0, "Post Filter"=[], "Gain"=[], "FS"=0, "IntOC"=0, "IntFC"=0, "SysOC"=0, "Cofficient"=[], "K"=[], "Max"=0}, "System"={"Out Type"=0, "Inverse"=0, "Monitor"=0, "Reserve"=0, "ACC Time"=0, "Pulse Rev"=0, "Stroke"=0, "Auto Off"=0, "Gear Ratio"=0.0, "Pitch"=0.0, "Max Speed"=0, "Jog Speed"=0, "Disp Coff"=0.0, "Max Load"=0}, "Index"=enum."Ch1", "Datalog"=enum."Empty"}}, "UDP ref"=w3617) -> (w3621:T5)
          }
          frame "Idle" {
            n1700 = Unbundle By Name(w3630) -> ("UDP ref"=w3634:refnum<event-registration>)
            n1701 = event shown="[1] <FDTI ref>: User Event" {
              selector: w3634 -> [_ _]
              dyn-events: _ -> [_ _]
              timeout: _ -> [_ _]
              tunnel: [w3640 w3642] -> w3628
              tunnel: [w3637 _] -> w3633
              tunnel: w3632 -> [w3637 _]
              tunnel: [w3635 w3652] -> w3631
              tunnel: w3630 -> [w3635 w3651]
              event Timeout {
                n1702 = event-data() -> ()  [unwired: 1 in, 1 out]
                n1703 = local read "Stop"() -> (w3639:bool)
                n1704 = Select(t=Communications_-_State."Close", s=w3639, f=Communications_-_State."Idle") -> (s? t:f=w3640:T1)
              }
              event User Event {
                n1705 = event-data() -> ("IP"=w3645:string, "CMD"=w3650:T3, "Data"=w3649:T6)  [unwired: 1 in]
                n1706 = global read "Global - IP Address.vi" "IP"() -> (w3648:string[])
                n1707 = Index Array(array=w3648, index=11) -> (element=w3646:string)
                n1708 = Equal?(x=w3646, y=w3645) -> (x = y?=w3644:bool)
                n1709 = Bundle By Name(cluster=w3651, "UDP CMD.IP"=w3645, "UDP CMD.CMD"=w3650, "Data"=w3649) -> (w3652:T5)
                n1710 = Select(t=Communications_-_State."Command" ("f"), s=w3644, f=Communications_-_State."Idle") -> (s? t:f=w3642:T1)
              }
            }
            n1711 = global read "Global - Hold.vi" "Hold"() -> (w3629:bool)
            n1712 = Select(t=Communications_-_State."Idle", s=w3629, f=w3628) -> (s? t:f=w3627:T1)
          }
          frame "Command" {
            (unwired) UDP_-_Command."Stop" ("Enum")
            (unwired) 20
            n1713 = Unbundle By Name(w3669) -> ("UDP CMD.CMD"=w3666:T3, "Data"=w3668:T6, "UDP CMD.IP"=w3663:string)
            n1714 = global read "Global - Handle.vi" "Handle"() -> (w3658:T7)
            n1715 = global read "Global - IP Address.vi" "IP"() -> (w3656:string[])
            n1716 = Search 1D Array(1D array=w3656, element=w3663) -> (index of element=w3654:i32)  [unwired: 1 in]
            n1717 = Index Array(array=w3658, index=w3654) -> (element=w3662:T8)
            n1718 = call "UDP - Write CMD.vi"("CMD"=w3666, "error in"=w3670, "Data"=w3668, "UDP Info"=w3662) -> ("error out"=w3660:errorcluster, "IP Address"=w3655:string, "Data Out"=w3665:T11, "Success"=w3664:bool)  [unwired: 2 in, 2 out]
            n1719 = Wait (ms)(milliseconds to wait=u32 5) -> ()  [unwired: 1 out]
            n1720 = Search 1D Array(1D array=w3656, element=w3655) -> (index of element=w3653:i32)  [unwired: 1 in]
            n1721 = global read "Global - Done.vi" "Done"() -> (w3661:bool[])
            n1722 = Replace Array Subset(array=w3661, new element=w3664, index=w3653) -> (w3659:bool[])
            n1723 = global write "Global - Done.vi" "Done"(w3659) -> ()
            n1724 = case shown="True" w3664 {
              tunnel: w3660 -> [w3672 w3678]
              tunnel: [w3673 w3677] -> w3667
              tunnel: w3666 -> [_ w3679]
              tunnel: w3665 -> [_ w3676]
              tunnel: w3653 -> [_ w3675]
              frame False {
                n1725 = call "Communication - Trigger Read IP Address(FGV).vi"("Action"=eFGV_States."Write", "error in"=w3672) -> ("error out"=w3673:errorcluster)  [unwired: 7 in, 2 out]
              }
              frame True {
                n1726 = case shown="\"Read Ch Data\"" w3679 {
                  tunnel: w3678 -> [w3680 w3687 w3694 w3700 w3706 w3712 w3718]
                  tunnel: [w3680 w3687 w3694 w3700 w3706 w3712 w3718] -> w3677
                  tunnel: w3676 -> [_ w3685 w3691 w3699 w3705 w3711 w3717]
                  tunnel: w3675 -> [_ w3689 w3695 w3701 w3707 w3713 w3719]
                  frame "Stop", Default {
                  }
                  frame "Read Ch Data" {
                    n1727 = Unbundle By Name(w3685) -> ("Channels"=w3684:T12, "Event"=w3683:T10, "Status"=w3682:T9)
                    n1728 = global read "Global - Channel.vi" "Data"() -> (w3688:T13)
                    n1729 = Bundle("Channels"=w3684, "Event"=w3683, "Status"=w3682) -> (w3681:T14)  [unwired: 1 in]
                    n1730 = Replace Array Subset(array=w3688, new element=w3681, index=w3689) -> (w3686:T13)
                    n1731 = global write "Global - Channel.vi" "Data"(w3686) -> ()
                  }
                  frame "Read Sensor" {
                    n1732 = Unbundle By Name(w3691) -> ("Sensor"=w3690:T15)
                    n1733 = global read "Global - Unit.vi" "Unit"() -> (w3692:T16)
                    n1734 = Replace Array Subset(array=w3692, new element=w3690, index=w3695) -> (w3693:T16)
                    n1735 = global write "Global - Unit.vi" "Unit"(w3693) -> ()
                  }
                  frame "Read ADC" {
                    n1736 = Unbundle By Name(w3699) -> ("ADC"=w3696:T17)
                    n1737 = global read "Global - ADC.vi" "ADC"() -> (w3698:T18)
                    n1738 = Replace Array Subset(array=w3698, new element=w3696, index=w3701) -> (w3697:T18)
                    n1739 = global write "Global - ADC.vi" "ADC"(w3697) -> ()
                  }
                  frame "Read PID" {
                    n1740 = Unbundle By Name(w3705) -> ("PID"=w3702:T19)
                    n1741 = global read "Global - PID.vi" "PID"() -> (w3704:T20)
                    n1742 = Replace Array Subset(array=w3704, new element=w3702, index=w3707) -> (w3703:T20)
                    n1743 = global write "Global - PID.vi" "PID"(w3703) -> ()
                  }
                  frame "Read System" {
                    n1744 = Unbundle By Name(w3711) -> ("System"=w3709:T21)
                    n1745 = global read "Global - System.vi" "System"() -> (w3710:T22)
                    n1746 = Replace Array Subset(array=w3710, new element=w3709, index=w3713) -> (w3708:T22)
                    n1747 = global write "Global - System.vi" "System"(w3708) -> ()
                  }
                  frame "Read Test" {
                    n1748 = Unbundle By Name(w3717) -> ("Test"=w3714:T23)
                    n1749 = global read "Global - Test.vi" "Test"() -> (w3715:T24)
                    n1750 = Replace Array Subset(array=w3715, new element=w3714, index=w3719) -> (w3716:T24)
                    n1751 = global write "Global - Test.vi" "Test"(w3716) -> ()
                  }
                }
              }
            }
          }
          frame "Close" {
          }
        }
      }
      frame Error {
        n1752 = global read "Global - IP Address.vi" "IP"() -> (w3732:string[])
        n1753 = Unbundle By Name(w3733) -> ("source"=w3728:string)
        n1754 = Index Array(array=w3732, index=0) -> (element=w3730:string)
        n1755 = Concatenate Strings(w3730, " - " ("string"), w3728) -> (w3724:string)
        n1756 = call <vilib>:"Clear Errors.vi"("error in (no error)"=w3733) -> ("error out"=w3727:errorcluster)  [unwired: 5 in, 1 out]
        n1757 = call "General - Error Log eFGV.vi"("eFGV States"=eFGV_States."Write", "error in (no error)"=w3727, "Error In"=w3724) -> ("error out"=w3726:errorcluster)  [unwired: 6 in, 2 out]
        n1758 = Wait (ms)(milliseconds to wait=u32 100) -> ()  [unwired: 1 out]
      }
    }
  }
  n1759 = while {
    shift-right: [w3742] -> _
    shift-left: errorcluster {"status"=FALSE, "code"=0, "source"=""} ("error IO") -> [w3743]
    shift-right: [w3740] -> _
    shift-left: Communications_-_State."Init" -> [w3741]
    shift-right: [w3738] -> _
    shift-left: _ -> [w3737]
    stop <- w3739 stop-if-true
    # "Command Processing Loop"
    n1760 = case shown="No Error" w3743 {
      selector: w3743 -> [w3749 w3867]
      tunnel: [w3750 w3860] -> w3742
      tunnel: w3741 -> [w3748 _]
      tunnel: [w3747 Communications_-_State."Idle"] -> w3740
      tunnel: [w3746 _] -> w3739
      tunnel: [w3745 w3869] -> w3738
      tunnel: w3737 -> [w3744 w3869]
      frame No Error {
        n1761 = case shown="\"Idle\"" w3748 {
          tunnel: [w3753 w3767 w3801 w3857] -> w3750
          tunnel: w3749 -> [w3758 w3766 w3804 w3857]
          tunnel: [Communications_-_State."Idle" w3761 Communications_-_State."Idle" Communications_-_State."Close"] -> w3747
          tunnel: [_ _ _ TRUE] -> w3746
          tunnel: [w3755 w3765 w3803 w3854] -> w3745
          tunnel: w3744 -> [_ w3764 w3803 w3854]
          frame "Init", Default {
            n1762 = call "Communication - UDP Command (eFGV).vi"("Action"=eFGV_States."Read", "error in"=w3758) -> ("error out"=w3754:errorcluster, "UDP Ref"=w3752:refnum<user-event>)  [unwired: 7 in, 1 out]
            n1763 = register-events(error in=w3754, w3752) -> (reference out=w3751:refnum<event-registration>, error out=w3753:errorcluster)  [unwired: 1 in]
            n1764 = Bundle By Name(cluster=T5 {"UDP CMD"={"IP"="", "CMD"=enum."Stop", "Port"="", "Datalog?"=FALSE, "Float"=0.0}, "UDP ref"=refnum, "Unit?"=FALSE, "Read Unit"=[], "Trig?"=FALSE, "UDP Info"=[], "UDP Conn ref"=refnum, "DataLogger"=[], "VISA Ref"=refnum, "Float"=0.0, "Data"={"Test"={"Target Load"=0.0, "Target Disp"=0.0, "Rate"=0.0, "Speed"=0.0}, "Sensor"={"Name"=[], "Unit"=[], "Decimal Point"=[], "Ch Log"=[], "H Alarm"=[], "L Alarm"=[], "H Limit"=[], "L Limit"=[], "Filter"=[], "Gain"=[], "Calib Type"=[]}, "PID"={"SP"=0.0, "PV"=0.0, "kP"=0.0, "kI"=0.0, "kD"=0.0, "FF"=0.0, "Err Band"=0.0, "Max"=0, "Min"=0, "Ts"=0, "Out"=0, "Mode"=0}, "ADC"={"Active Ch"=[], "Filter Type"=0, "Post Filter"=[], "Gain"=[], "FS"=0, "IntOC"=0, "IntFC"=0, "SysOC"=0, "Cofficient"=[], "K"=[], "Max"=0}, "System"={"Out Type"=0, "Inverse"=0, "Monitor"=0, "Reserve"=0, "ACC Time"=0, "Pulse Rev"=0, "Stroke"=0, "Auto Off"=0, "Gear Ratio"=0.0, "Pitch"=0.0, "Max Speed"=0, "Jog Speed"=0, "Disp Coff"=0.0, "Max Load"=0}, "Index"=enum."Ch1", "Datalog"=enum."Empty"}}, "UDP ref"=w3751) -> (w3755:T5)
          }
          frame "Idle" {
            n1765 = Unbundle By Name(w3764) -> ("UDP ref"=w3768:refnum<event-registration>)
            n1766 = event shown="[1] <FDTI ref>: User Event" {
              selector: w3768 -> [_ _]
              dyn-events: _ -> [_ _]
              timeout: _ -> [_ _]
              tunnel: [w3774 w3776] -> w3762
              tunnel: [w3771 _] -> w3767
              tunnel: w3766 -> [w3771 _]
              tunnel: [w3769 w3786] -> w3765
              tunnel: w3764 -> [w3769 w3785]
              event Timeout {
                n1767 = event-data() -> ()  [unwired: 1 in, 1 out]
                n1768 = local read "Stop"() -> (w3773:bool)
                n1769 = Select(t=Communications_-_State."Close", s=w3773, f=Communications_-_State."Idle") -> (s? t:f=w3774:T1)
              }
              event User Event {
                n1770 = event-data() -> ("IP"=w3779:string, "CMD"=w3784:T3, "Data"=w3783:T6)  [unwired: 1 in]
                n1771 = global read "Global - IP Address.vi" "IP"() -> (w3782:string[])
                n1772 = Index Array(array=w3782, index=17) -> (element=w3780:string)
                n1773 = Equal?(x=w3780, y=w3779) -> (x = y?=w3778:bool)
                n1774 = Bundle By Name(cluster=w3785, "UDP CMD.IP"=w3779, "UDP CMD.CMD"=w3784, "Data"=w3783) -> (w3786:T5)
                n1775 = Select(t=Communications_-_State."Command" ("f"), s=w3778, f=Communications_-_State."Idle") -> (s? t:f=w3776:T1)
              }
            }
            n1776 = global read "Global - Hold.vi" "Hold"() -> (w3763:bool)
            n1777 = Select(t=Communications_-_State."Idle", s=w3763, f=w3762) -> (s? t:f=w3761:T1)
          }
          frame "Command" {
            (unwired) UDP_-_Command."Stop" ("Enum")
            (unwired) 20
            n1778 = Unbundle By Name(w3803) -> ("UDP CMD.CMD"=w3800:T3, "Data"=w3802:T6, "UDP CMD.IP"=w3797:string)
            n1779 = global read "Global - Handle.vi" "Handle"() -> (w3792:T7)
            n1780 = global read "Global - IP Address.vi" "IP"() -> (w3790:string[])
            n1781 = Search 1D Array(1D array=w3790, element=w3797) -> (index of element=w3788:i32)  [unwired: 1 in]
            n1782 = Index Array(array=w3792, index=w3788) -> (element=w3796:T8)
            n1783 = call "UDP - Write CMD.vi"("CMD"=w3800, "error in"=w3804, "Data"=w3802, "UDP Info"=w3796) -> ("error out"=w3794:errorcluster, "IP Address"=w3789:string, "Data Out"=w3799:T11, "Success"=w3798:bool)  [unwired: 2 in, 2 out]
            n1784 = Wait (ms)(milliseconds to wait=u32 5) -> ()  [unwired: 1 out]
            n1785 = Search 1D Array(1D array=w3790, element=w3789) -> (index of element=w3787:i32)  [unwired: 1 in]
            n1786 = global read "Global - Done.vi" "Done"() -> (w3795:bool[])
            n1787 = Replace Array Subset(array=w3795, new element=w3798, index=w3787) -> (w3793:bool[])
            n1788 = global write "Global - Done.vi" "Done"(w3793) -> ()
            n1789 = case shown="True" w3798 {
              tunnel: w3794 -> [w3806 w3812]
              tunnel: [w3807 w3811] -> w3801
              tunnel: w3800 -> [_ w3813]
              tunnel: w3799 -> [_ w3810]
              tunnel: w3787 -> [_ w3809]
              frame False {
                n1790 = call "Communication - Trigger Read IP Address(FGV).vi"("Action"=eFGV_States."Write", "error in"=w3806) -> ("error out"=w3807:errorcluster)  [unwired: 7 in, 2 out]
              }
              frame True {
                n1791 = case shown="\"Read Ch Data\"" w3813 {
                  tunnel: w3812 -> [w3814 w3821 w3828 w3834 w3840 w3846 w3852]
                  tunnel: [w3814 w3821 w3828 w3834 w3840 w3846 w3852] -> w3811
                  tunnel: w3810 -> [_ w3819 w3825 w3833 w3839 w3845 w3851]
                  tunnel: w3809 -> [_ w3823 w3829 w3835 w3841 w3847 w3853]
                  frame "Stop", Default {
                  }
                  frame "Read Ch Data" {
                    n1792 = Unbundle By Name(w3819) -> ("Channels"=w3818:T12, "Event"=w3817:T10, "Status"=w3816:T9)
                    n1793 = global read "Global - Channel.vi" "Data"() -> (w3822:T13)
                    n1794 = Bundle("Channels"=w3818, "Event"=w3817, "Status"=w3816) -> (w3815:T14)  [unwired: 1 in]
                    n1795 = Replace Array Subset(array=w3822, new element=w3815, index=w3823) -> (w3820:T13)
                    n1796 = global write "Global - Channel.vi" "Data"(w3820) -> ()
                  }
                  frame "Read Sensor" {
                    n1797 = Unbundle By Name(w3825) -> ("Sensor"=w3824:T15)
                    n1798 = global read "Global - Unit.vi" "Unit"() -> (w3826:T16)
                    n1799 = Replace Array Subset(array=w3826, new element=w3824, index=w3829) -> (w3827:T16)
                    n1800 = global write "Global - Unit.vi" "Unit"(w3827) -> ()
                  }
                  frame "Read ADC" {
                    n1801 = Unbundle By Name(w3833) -> ("ADC"=w3830:T17)
                    n1802 = global read "Global - ADC.vi" "ADC"() -> (w3832:T18)
                    n1803 = Replace Array Subset(array=w3832, new element=w3830, index=w3835) -> (w3831:T18)
                    n1804 = global write "Global - ADC.vi" "ADC"(w3831) -> ()
                  }
                  frame "Read PID" {
                    n1805 = Unbundle By Name(w3839) -> ("PID"=w3836:T19)
                    n1806 = global read "Global - PID.vi" "PID"() -> (w3838:T20)
                    n1807 = Replace Array Subset(array=w3838, new element=w3836, index=w3841) -> (w3837:T20)
                    n1808 = global write "Global - PID.vi" "PID"(w3837) -> ()
                  }
                  frame "Read System" {
                    n1809 = Unbundle By Name(w3845) -> ("System"=w3843:T21)
                    n1810 = global read "Global - System.vi" "System"() -> (w3844:T22)
                    n1811 = Replace Array Subset(array=w3844, new element=w3843, index=w3847) -> (w3842:T22)
                    n1812 = global write "Global - System.vi" "System"(w3842) -> ()
                  }
                  frame "Read Test" {
                    n1813 = Unbundle By Name(w3851) -> ("Test"=w3848:T23)
                    n1814 = global read "Global - Test.vi" "Test"() -> (w3849:T24)
                    n1815 = Replace Array Subset(array=w3849, new element=w3848, index=w3853) -> (w3850:T24)
                    n1816 = global write "Global - Test.vi" "Test"(w3850) -> ()
                  }
                }
              }
            }
          }
          frame "Close" {
          }
        }
      }
      frame Error {
        n1817 = global read "Global - IP Address.vi" "IP"() -> (w3866:string[])
        n1818 = Unbundle By Name(w3867) -> ("source"=w3862:string)
        n1819 = Index Array(array=w3866, index=0) -> (element=w3864:string)
        n1820 = Concatenate Strings(w3864, " - " ("string"), w3862) -> (w3858:string)
        n1821 = call <vilib>:"Clear Errors.vi"("error in (no error)"=w3867) -> ("error out"=w3861:errorcluster)  [unwired: 5 in, 1 out]
        n1822 = call "General - Error Log eFGV.vi"("eFGV States"=eFGV_States."Write", "error in (no error)"=w3861, "Error In"=w3858) -> ("error out"=w3860:errorcluster)  [unwired: 6 in, 2 out]
        n1823 = Wait (ms)(milliseconds to wait=u32 100) -> ()  [unwired: 1 out]
      }
    }
  }
  n1824 = while {
    shift-right: [w3876] -> _
    shift-left: errorcluster {"status"=FALSE, "code"=0, "source"=""} ("error IO") -> [w3877]
    shift-right: [w3874] -> _
    shift-left: Communications_-_State."Init" -> [w3875]
    shift-right: [w3872] -> _
    shift-left: _ -> [w3871]
    stop <- w3873 stop-if-true
    # "Command Processing Loop"
    n1825 = case shown="No Error" w3877 {
      selector: w3877 -> [w3883 w4001]
      tunnel: [w3884 w3994] -> w3876
      tunnel: w3875 -> [w3882 _]
      tunnel: [w3881 Communications_-_State."Idle"] -> w3874
      tunnel: [w3880 _] -> w3873
      tunnel: [w3879 w4003] -> w3872
      tunnel: w3871 -> [w3878 w4003]
      frame No Error {
        n1826 = case shown="\"Idle\"" w3882 {
          tunnel: [w3887 w3901 w3935 w3991] -> w3884
          tunnel: w3883 -> [w3892 w3900 w3938 w3991]
          tunnel: [Communications_-_State."Idle" w3895 Communications_-_State."Idle" Communications_-_State."Close"] -> w3881
          tunnel: [_ _ _ TRUE] -> w3880
          tunnel: [w3889 w3899 w3937 w3988] -> w3879
          tunnel: w3878 -> [_ w3898 w3937 w3988]
          frame "Init", Default {
            n1827 = call "Communication - UDP Command (eFGV).vi"("Action"=eFGV_States."Read", "error in"=w3892) -> ("error out"=w3888:errorcluster, "UDP Ref"=w3886:refnum<user-event>)  [unwired: 7 in, 1 out]
            n1828 = register-events(error in=w3888, w3886) -> (reference out=w3885:refnum<event-registration>, error out=w3887:errorcluster)  [unwired: 1 in]
            n1829 = Bundle By Name(cluster=T5 {"UDP CMD"={"IP"="", "CMD"=enum."Stop", "Port"="", "Datalog?"=FALSE, "Float"=0.0}, "UDP ref"=refnum, "Unit?"=FALSE, "Read Unit"=[], "Trig?"=FALSE, "UDP Info"=[], "UDP Conn ref"=refnum, "DataLogger"=[], "VISA Ref"=refnum, "Float"=0.0, "Data"={"Test"={"Target Load"=0.0, "Target Disp"=0.0, "Rate"=0.0, "Speed"=0.0}, "Sensor"={"Name"=[], "Unit"=[], "Decimal Point"=[], "Ch Log"=[], "H Alarm"=[], "L Alarm"=[], "H Limit"=[], "L Limit"=[], "Filter"=[], "Gain"=[], "Calib Type"=[]}, "PID"={"SP"=0.0, "PV"=0.0, "kP"=0.0, "kI"=0.0, "kD"=0.0, "FF"=0.0, "Err Band"=0.0, "Max"=0, "Min"=0, "Ts"=0, "Out"=0, "Mode"=0}, "ADC"={"Active Ch"=[], "Filter Type"=0, "Post Filter"=[], "Gain"=[], "FS"=0, "IntOC"=0, "IntFC"=0, "SysOC"=0, "Cofficient"=[], "K"=[], "Max"=0}, "System"={"Out Type"=0, "Inverse"=0, "Monitor"=0, "Reserve"=0, "ACC Time"=0, "Pulse Rev"=0, "Stroke"=0, "Auto Off"=0, "Gear Ratio"=0.0, "Pitch"=0.0, "Max Speed"=0, "Jog Speed"=0, "Disp Coff"=0.0, "Max Load"=0}, "Index"=enum."Ch1", "Datalog"=enum."Empty"}}, "UDP ref"=w3885) -> (w3889:T5)
          }
          frame "Idle" {
            n1830 = Unbundle By Name(w3898) -> ("UDP ref"=w3902:refnum<event-registration>)
            n1831 = event shown="[1] <FDTI ref>: User Event" {
              selector: w3902 -> [_ _]
              dyn-events: _ -> [_ _]
              timeout: _ -> [_ _]
              tunnel: [w3908 w3910] -> w3896
              tunnel: [w3905 _] -> w3901
              tunnel: w3900 -> [w3905 _]
              tunnel: [w3903 w3920] -> w3899
              tunnel: w3898 -> [w3903 w3919]
              event Timeout {
                n1832 = event-data() -> ()  [unwired: 1 in, 1 out]
                n1833 = local read "Stop"() -> (w3907:bool)
                n1834 = Select(t=Communications_-_State."Close", s=w3907, f=Communications_-_State."Idle") -> (s? t:f=w3908:T1)
              }
              event User Event {
                n1835 = event-data() -> ("IP"=w3913:string, "CMD"=w3918:T3, "Data"=w3917:T6)  [unwired: 1 in]
                n1836 = global read "Global - IP Address.vi" "IP"() -> (w3916:string[])
                n1837 = Index Array(array=w3916, index=19) -> (element=w3914:string)
                n1838 = Equal?(x=w3914, y=w3913) -> (x = y?=w3912:bool)
                n1839 = Bundle By Name(cluster=w3919, "UDP CMD.IP"=w3913, "UDP CMD.CMD"=w3918, "Data"=w3917) -> (w3920:T5)
                n1840 = Select(t=Communications_-_State."Command" ("f"), s=w3912, f=Communications_-_State."Idle") -> (s? t:f=w3910:T1)
              }
            }
            n1841 = global read "Global - Hold.vi" "Hold"() -> (w3897:bool)
            n1842 = Select(t=Communications_-_State."Idle", s=w3897, f=w3896) -> (s? t:f=w3895:T1)
          }
          frame "Command" {
            (unwired) UDP_-_Command."Stop" ("Enum")
            (unwired) 20
            n1843 = Unbundle By Name(w3937) -> ("UDP CMD.CMD"=w3934:T3, "Data"=w3936:T6, "UDP CMD.IP"=w3931:string)
            n1844 = global read "Global - Handle.vi" "Handle"() -> (w3926:T7)
            n1845 = global read "Global - IP Address.vi" "IP"() -> (w3924:string[])
            n1846 = Search 1D Array(1D array=w3924, element=w3931) -> (index of element=w3922:i32)  [unwired: 1 in]
            n1847 = Index Array(array=w3926, index=w3922) -> (element=w3930:T8)
            n1848 = call "UDP - Write CMD.vi"("CMD"=w3934, "error in"=w3938, "Data"=w3936, "UDP Info"=w3930) -> ("error out"=w3928:errorcluster, "IP Address"=w3923:string, "Data Out"=w3933:T11, "Success"=w3932:bool)  [unwired: 2 in, 2 out]
            n1849 = Wait (ms)(milliseconds to wait=u32 5) -> ()  [unwired: 1 out]
            n1850 = Search 1D Array(1D array=w3924, element=w3923) -> (index of element=w3921:i32)  [unwired: 1 in]
            n1851 = global read "Global - Done.vi" "Done"() -> (w3929:bool[])
            n1852 = Replace Array Subset(array=w3929, new element=w3932, index=w3921) -> (w3927:bool[])
            n1853 = global write "Global - Done.vi" "Done"(w3927) -> ()
            n1854 = case shown="True" w3932 {
              tunnel: w3928 -> [w3940 w3946]
              tunnel: [w3941 w3945] -> w3935
              tunnel: w3934 -> [_ w3947]
              tunnel: w3933 -> [_ w3944]
              tunnel: w3921 -> [_ w3943]
              frame False {
                n1855 = call "Communication - Trigger Read IP Address(FGV).vi"("Action"=eFGV_States."Write", "error in"=w3940) -> ("error out"=w3941:errorcluster)  [unwired: 7 in, 2 out]
              }
              frame True {
                n1856 = case shown="\"Read Ch Data\"" w3947 {
                  tunnel: w3946 -> [w3948 w3955 w3962 w3968 w3974 w3980 w3986]
                  tunnel: [w3948 w3955 w3962 w3968 w3974 w3980 w3986] -> w3945
                  tunnel: w3944 -> [_ w3953 w3959 w3967 w3973 w3979 w3985]
                  tunnel: w3943 -> [_ w3957 w3963 w3969 w3975 w3981 w3987]
                  frame "Stop", Default {
                  }
                  frame "Read Ch Data" {
                    n1857 = Unbundle By Name(w3953) -> ("Channels"=w3952:T12, "Event"=w3951:T10, "Status"=w3950:T9)
                    n1858 = global read "Global - Channel.vi" "Data"() -> (w3956:T13)
                    n1859 = Bundle("Channels"=w3952, "Event"=w3951, "Status"=w3950) -> (w3949:T14)  [unwired: 1 in]
                    n1860 = Replace Array Subset(array=w3956, new element=w3949, index=w3957) -> (w3954:T13)
                    n1861 = global write "Global - Channel.vi" "Data"(w3954) -> ()
                  }
                  frame "Read Sensor" {
                    n1862 = Unbundle By Name(w3959) -> ("Sensor"=w3958:T15)
                    n1863 = global read "Global - Unit.vi" "Unit"() -> (w3960:T16)
                    n1864 = Replace Array Subset(array=w3960, new element=w3958, index=w3963) -> (w3961:T16)
                    n1865 = global write "Global - Unit.vi" "Unit"(w3961) -> ()
                  }
                  frame "Read ADC" {
                    n1866 = Unbundle By Name(w3967) -> ("ADC"=w3964:T17)
                    n1867 = global read "Global - ADC.vi" "ADC"() -> (w3966:T18)
                    n1868 = Replace Array Subset(array=w3966, new element=w3964, index=w3969) -> (w3965:T18)
                    n1869 = global write "Global - ADC.vi" "ADC"(w3965) -> ()
                  }
                  frame "Read PID" {
                    n1870 = Unbundle By Name(w3973) -> ("PID"=w3970:T19)
                    n1871 = global read "Global - PID.vi" "PID"() -> (w3972:T20)
                    n1872 = Replace Array Subset(array=w3972, new element=w3970, index=w3975) -> (w3971:T20)
                    n1873 = global write "Global - PID.vi" "PID"(w3971) -> ()
                  }
                  frame "Read System" {
                    n1874 = Unbundle By Name(w3979) -> ("System"=w3977:T21)
                    n1875 = global read "Global - System.vi" "System"() -> (w3978:T22)
                    n1876 = Replace Array Subset(array=w3978, new element=w3977, index=w3981) -> (w3976:T22)
                    n1877 = global write "Global - System.vi" "System"(w3976) -> ()
                  }
                  frame "Read Test" {
                    n1878 = Unbundle By Name(w3985) -> ("Test"=w3982:T23)
                    n1879 = global read "Global - Test.vi" "Test"() -> (w3983:T24)
                    n1880 = Replace Array Subset(array=w3983, new element=w3982, index=w3987) -> (w3984:T24)
                    n1881 = global write "Global - Test.vi" "Test"(w3984) -> ()
                  }
                }
              }
            }
          }
          frame "Close" {
          }
        }
      }
      frame Error {
        n1882 = global read "Global - IP Address.vi" "IP"() -> (w4000:string[])
        n1883 = Unbundle By Name(w4001) -> ("source"=w3996:string)
        n1884 = Index Array(array=w4000, index=0) -> (element=w3998:string)
        n1885 = Concatenate Strings(w3998, " - " ("string"), w3996) -> (w3992:string)
        n1886 = call <vilib>:"Clear Errors.vi"("error in (no error)"=w4001) -> ("error out"=w3995:errorcluster)  [unwired: 5 in, 1 out]
        n1887 = call "General - Error Log eFGV.vi"("eFGV States"=eFGV_States."Write", "error in (no error)"=w3995, "Error In"=w3992) -> ("error out"=w3994:errorcluster)  [unwired: 6 in, 2 out]
        n1888 = Wait (ms)(milliseconds to wait=u32 100) -> ()  [unwired: 1 out]
      }
    }
  }
  n1889 = while {
    shift-right: [w4010] -> _
    shift-left: errorcluster {"status"=FALSE, "code"=0, "source"=""} ("error IO") -> [w4011]
    shift-right: [w4008] -> _
    shift-left: Communications_-_State."Init" -> [w4009]
    shift-right: [w4006] -> _
    shift-left: _ -> [w4005]
    stop <- w4007 stop-if-true
    # "Command Processing Loop"
    n1890 = case shown="No Error" w4011 {
      selector: w4011 -> [w4017 w4135]
      tunnel: [w4018 w4128] -> w4010
      tunnel: w4009 -> [w4016 _]
      tunnel: [w4015 Communications_-_State."Idle"] -> w4008
      tunnel: [w4014 _] -> w4007
      tunnel: [w4013 w4137] -> w4006
      tunnel: w4005 -> [w4012 w4137]
      frame No Error {
        n1891 = case shown="\"Idle\"" w4016 {
          tunnel: [w4021 w4035 w4069 w4125] -> w4018
          tunnel: w4017 -> [w4026 w4034 w4072 w4125]
          tunnel: [Communications_-_State."Idle" w4029 Communications_-_State."Idle" Communications_-_State."Close"] -> w4015
          tunnel: [_ _ _ TRUE] -> w4014
          tunnel: [w4023 w4033 w4071 w4122] -> w4013
          tunnel: w4012 -> [_ w4032 w4071 w4122]
          frame "Init", Default {
            n1892 = call "Communication - UDP Command (eFGV).vi"("Action"=eFGV_States."Read", "error in"=w4026) -> ("error out"=w4022:errorcluster, "UDP Ref"=w4020:refnum<user-event>)  [unwired: 7 in, 1 out]
            n1893 = register-events(error in=w4022, w4020) -> (reference out=w4019:refnum<event-registration>, error out=w4021:errorcluster)  [unwired: 1 in]
            n1894 = Bundle By Name(cluster=T5 {"UDP CMD"={"IP"="", "CMD"=enum."Stop", "Port"="", "Datalog?"=FALSE, "Float"=0.0}, "UDP ref"=refnum, "Unit?"=FALSE, "Read Unit"=[], "Trig?"=FALSE, "UDP Info"=[], "UDP Conn ref"=refnum, "DataLogger"=[], "VISA Ref"=refnum, "Float"=0.0, "Data"={"Test"={"Target Load"=0.0, "Target Disp"=0.0, "Rate"=0.0, "Speed"=0.0}, "Sensor"={"Name"=[], "Unit"=[], "Decimal Point"=[], "Ch Log"=[], "H Alarm"=[], "L Alarm"=[], "H Limit"=[], "L Limit"=[], "Filter"=[], "Gain"=[], "Calib Type"=[]}, "PID"={"SP"=0.0, "PV"=0.0, "kP"=0.0, "kI"=0.0, "kD"=0.0, "FF"=0.0, "Err Band"=0.0, "Max"=0, "Min"=0, "Ts"=0, "Out"=0, "Mode"=0}, "ADC"={"Active Ch"=[], "Filter Type"=0, "Post Filter"=[], "Gain"=[], "FS"=0, "IntOC"=0, "IntFC"=0, "SysOC"=0, "Cofficient"=[], "K"=[], "Max"=0}, "System"={"Out Type"=0, "Inverse"=0, "Monitor"=0, "Reserve"=0, "ACC Time"=0, "Pulse Rev"=0, "Stroke"=0, "Auto Off"=0, "Gear Ratio"=0.0, "Pitch"=0.0, "Max Speed"=0, "Jog Speed"=0, "Disp Coff"=0.0, "Max Load"=0}, "Index"=enum."Ch1", "Datalog"=enum."Empty"}}, "UDP ref"=w4019) -> (w4023:T5)
          }
          frame "Idle" {
            n1895 = Unbundle By Name(w4032) -> ("UDP ref"=w4036:refnum<event-registration>)
            n1896 = event shown="[1] <FDTI ref>: User Event" {
              selector: w4036 -> [_ _]
              dyn-events: _ -> [_ _]
              timeout: _ -> [_ _]
              tunnel: [w4042 w4044] -> w4030
              tunnel: [w4039 _] -> w4035
              tunnel: w4034 -> [w4039 _]
              tunnel: [w4037 w4054] -> w4033
              tunnel: w4032 -> [w4037 w4053]
              event Timeout {
                n1897 = event-data() -> ()  [unwired: 1 in, 1 out]
                n1898 = local read "Stop"() -> (w4041:bool)
                n1899 = Select(t=Communications_-_State."Close", s=w4041, f=Communications_-_State."Idle") -> (s? t:f=w4042:T1)
              }
              event User Event {
                n1900 = event-data() -> ("IP"=w4047:string, "CMD"=w4052:T3, "Data"=w4051:T6)  [unwired: 1 in]
                n1901 = global read "Global - IP Address.vi" "IP"() -> (w4050:string[])
                n1902 = Index Array(array=w4050, index=5) -> (element=w4048:string)
                n1903 = Equal?(x=w4048, y=w4047) -> (x = y?=w4046:bool)
                n1904 = Bundle By Name(cluster=w4053, "UDP CMD.IP"=w4047, "UDP CMD.CMD"=w4052, "Data"=w4051) -> (w4054:T5)
                n1905 = Select(t=Communications_-_State."Command" ("f"), s=w4046, f=Communications_-_State."Idle") -> (s? t:f=w4044:T1)
              }
            }
            n1906 = global read "Global - Hold.vi" "Hold"() -> (w4031:bool)
            n1907 = Select(t=Communications_-_State."Idle", s=w4031, f=w4030) -> (s? t:f=w4029:T1)
          }
          frame "Command" {
            (unwired) UDP_-_Command."Stop" ("Enum")
            (unwired) 20
            n1908 = Unbundle By Name(w4071) -> ("UDP CMD.CMD"=w4068:T3, "Data"=w4070:T6, "UDP CMD.IP"=w4065:string)
            n1909 = global read "Global - Handle.vi" "Handle"() -> (w4060:T7)
            n1910 = global read "Global - IP Address.vi" "IP"() -> (w4058:string[])
            n1911 = Search 1D Array(1D array=w4058, element=w4065) -> (index of element=w4056:i32)  [unwired: 1 in]
            n1912 = Index Array(array=w4060, index=w4056) -> (element=w4064:T8)
            n1913 = call "UDP - Write CMD.vi"("CMD"=w4068, "error in"=w4072, "Data"=w4070, "UDP Info"=w4064) -> ("error out"=w4062:errorcluster, "IP Address"=w4057:string, "Data Out"=w4067:T11, "Success"=w4066:bool)  [unwired: 2 in, 2 out]
            n1914 = Wait (ms)(milliseconds to wait=u32 5) -> ()  [unwired: 1 out]
            n1915 = Search 1D Array(1D array=w4058, element=w4057) -> (index of element=w4055:i32)  [unwired: 1 in]
            n1916 = global read "Global - Done.vi" "Done"() -> (w4063:bool[])
            n1917 = Replace Array Subset(array=w4063, new element=w4066, index=w4055) -> (w4061:bool[])
            n1918 = global write "Global - Done.vi" "Done"(w4061) -> ()
            n1919 = case shown="True" w4066 {
              tunnel: w4062 -> [w4074 w4080]
              tunnel: [w4075 w4079] -> w4069
              tunnel: w4068 -> [_ w4081]
              tunnel: w4067 -> [_ w4078]
              tunnel: w4055 -> [_ w4077]
              frame False {
                n1920 = call "Communication - Trigger Read IP Address(FGV).vi"("Action"=eFGV_States."Write", "error in"=w4074) -> ("error out"=w4075:errorcluster)  [unwired: 7 in, 2 out]
              }
              frame True {
                n1921 = case shown="\"Read Ch Data\"" w4081 {
                  tunnel: w4080 -> [w4082 w4089 w4096 w4102 w4108 w4114 w4120]
                  tunnel: [w4082 w4089 w4096 w4102 w4108 w4114 w4120] -> w4079
                  tunnel: w4078 -> [_ w4087 w4093 w4101 w4107 w4113 w4119]
                  tunnel: w4077 -> [_ w4091 w4097 w4103 w4109 w4115 w4121]
                  frame "Stop", Default {
                  }
                  frame "Read Ch Data" {
                    n1922 = Unbundle By Name(w4087) -> ("Channels"=w4086:T12, "Event"=w4085:T10, "Status"=w4084:T9)
                    n1923 = global read "Global - Channel.vi" "Data"() -> (w4090:T13)
                    n1924 = Bundle("Channels"=w4086, "Event"=w4085, "Status"=w4084) -> (w4083:T14)  [unwired: 1 in]
                    n1925 = Replace Array Subset(array=w4090, new element=w4083, index=w4091) -> (w4088:T13)
                    n1926 = global write "Global - Channel.vi" "Data"(w4088) -> ()
                  }
                  frame "Read Sensor" {
                    n1927 = Unbundle By Name(w4093) -> ("Sensor"=w4092:T15)
                    n1928 = global read "Global - Unit.vi" "Unit"() -> (w4094:T16)
                    n1929 = Replace Array Subset(array=w4094, new element=w4092, index=w4097) -> (w4095:T16)
                    n1930 = global write "Global - Unit.vi" "Unit"(w4095) -> ()
                  }
                  frame "Read ADC" {
                    n1931 = Unbundle By Name(w4101) -> ("ADC"=w4098:T17)
                    n1932 = global read "Global - ADC.vi" "ADC"() -> (w4100:T18)
                    n1933 = Replace Array Subset(array=w4100, new element=w4098, index=w4103) -> (w4099:T18)
                    n1934 = global write "Global - ADC.vi" "ADC"(w4099) -> ()
                  }
                  frame "Read PID" {
                    n1935 = Unbundle By Name(w4107) -> ("PID"=w4104:T19)
                    n1936 = global read "Global - PID.vi" "PID"() -> (w4106:T20)
                    n1937 = Replace Array Subset(array=w4106, new element=w4104, index=w4109) -> (w4105:T20)
                    n1938 = global write "Global - PID.vi" "PID"(w4105) -> ()
                  }
                  frame "Read System" {
                    n1939 = Unbundle By Name(w4113) -> ("System"=w4111:T21)
                    n1940 = global read "Global - System.vi" "System"() -> (w4112:T22)
                    n1941 = Replace Array Subset(array=w4112, new element=w4111, index=w4115) -> (w4110:T22)
                    n1942 = global write "Global - System.vi" "System"(w4110) -> ()
                  }
                  frame "Read Test" {
                    n1943 = Unbundle By Name(w4119) -> ("Test"=w4116:T23)
                    n1944 = global read "Global - Test.vi" "Test"() -> (w4117:T24)
                    n1945 = Replace Array Subset(array=w4117, new element=w4116, index=w4121) -> (w4118:T24)
                    n1946 = global write "Global - Test.vi" "Test"(w4118) -> ()
                  }
                }
              }
            }
          }
          frame "Close" {
          }
        }
      }
      frame Error {
        n1947 = global read "Global - IP Address.vi" "IP"() -> (w4134:string[])
        n1948 = Unbundle By Name(w4135) -> ("source"=w4130:string)
        n1949 = Index Array(array=w4134, index=0) -> (element=w4132:string)
        n1950 = Concatenate Strings(w4132, " - " ("string"), w4130) -> (w4126:string)
        n1951 = call <vilib>:"Clear Errors.vi"("error in (no error)"=w4135) -> ("error out"=w4129:errorcluster)  [unwired: 5 in, 1 out]
        n1952 = call "General - Error Log eFGV.vi"("eFGV States"=eFGV_States."Write", "error in (no error)"=w4129, "Error In"=w4126) -> ("error out"=w4128:errorcluster)  [unwired: 6 in, 2 out]
        n1953 = Wait (ms)(milliseconds to wait=u32 100) -> ()  [unwired: 1 out]
      }
    }
  }
  n1954 = while {
    shift-right: [w4144] -> _
    shift-left: errorcluster {"status"=FALSE, "code"=0, "source"=""} ("error IO") -> [w4145]
    shift-right: [w4142] -> _
    shift-left: Communications_-_State."Init" -> [w4143]
    shift-right: [w4140] -> _
    shift-left: _ -> [w4139]
    stop <- w4141 stop-if-true
    # "Command Processing Loop"
    n1955 = case shown="No Error" w4145 {
      selector: w4145 -> [w4151 w4269]
      tunnel: [w4152 w4262] -> w4144
      tunnel: w4143 -> [w4150 _]
      tunnel: [w4149 Communications_-_State."Idle"] -> w4142
      tunnel: [w4148 _] -> w4141
      tunnel: [w4147 w4271] -> w4140
      tunnel: w4139 -> [w4146 w4271]
      frame No Error {
        n1956 = case shown="\"Idle\"" w4150 {
          tunnel: [w4155 w4169 w4203 w4259] -> w4152
          tunnel: w4151 -> [w4160 w4168 w4206 w4259]
          tunnel: [Communications_-_State."Idle" w4163 Communications_-_State."Idle" Communications_-_State."Close"] -> w4149
          tunnel: [_ _ _ TRUE] -> w4148
          tunnel: [w4157 w4167 w4205 w4256] -> w4147
          tunnel: w4146 -> [_ w4166 w4205 w4256]
          frame "Init", Default {
            n1957 = call "Communication - UDP Command (eFGV).vi"("Action"=eFGV_States."Read", "error in"=w4160) -> ("error out"=w4156:errorcluster, "UDP Ref"=w4154:refnum<user-event>)  [unwired: 7 in, 1 out]
            n1958 = register-events(error in=w4156, w4154) -> (reference out=w4153:refnum<event-registration>, error out=w4155:errorcluster)  [unwired: 1 in]
            n1959 = Bundle By Name(cluster=T5 {"UDP CMD"={"IP"="", "CMD"=enum."Stop", "Port"="", "Datalog?"=FALSE, "Float"=0.0}, "UDP ref"=refnum, "Unit?"=FALSE, "Read Unit"=[], "Trig?"=FALSE, "UDP Info"=[], "UDP Conn ref"=refnum, "DataLogger"=[], "VISA Ref"=refnum, "Float"=0.0, "Data"={"Test"={"Target Load"=0.0, "Target Disp"=0.0, "Rate"=0.0, "Speed"=0.0}, "Sensor"={"Name"=[], "Unit"=[], "Decimal Point"=[], "Ch Log"=[], "H Alarm"=[], "L Alarm"=[], "H Limit"=[], "L Limit"=[], "Filter"=[], "Gain"=[], "Calib Type"=[]}, "PID"={"SP"=0.0, "PV"=0.0, "kP"=0.0, "kI"=0.0, "kD"=0.0, "FF"=0.0, "Err Band"=0.0, "Max"=0, "Min"=0, "Ts"=0, "Out"=0, "Mode"=0}, "ADC"={"Active Ch"=[], "Filter Type"=0, "Post Filter"=[], "Gain"=[], "FS"=0, "IntOC"=0, "IntFC"=0, "SysOC"=0, "Cofficient"=[], "K"=[], "Max"=0}, "System"={"Out Type"=0, "Inverse"=0, "Monitor"=0, "Reserve"=0, "ACC Time"=0, "Pulse Rev"=0, "Stroke"=0, "Auto Off"=0, "Gear Ratio"=0.0, "Pitch"=0.0, "Max Speed"=0, "Jog Speed"=0, "Disp Coff"=0.0, "Max Load"=0}, "Index"=enum."Ch1", "Datalog"=enum."Empty"}}, "UDP ref"=w4153) -> (w4157:T5)
          }
          frame "Idle" {
            n1960 = Unbundle By Name(w4166) -> ("UDP ref"=w4170:refnum<event-registration>)
            n1961 = event shown="[1] <FDTI ref>: User Event" {
              selector: w4170 -> [_ _]
              dyn-events: _ -> [_ _]
              timeout: _ -> [_ _]
              tunnel: [w4176 w4178] -> w4164
              tunnel: [w4173 _] -> w4169
              tunnel: w4168 -> [w4173 _]
              tunnel: [w4171 w4188] -> w4167
              tunnel: w4166 -> [w4171 w4187]
              event Timeout {
                n1962 = event-data() -> ()  [unwired: 1 in, 1 out]
                n1963 = local read "Stop"() -> (w4175:bool)
                n1964 = Select(t=Communications_-_State."Close", s=w4175, f=Communications_-_State."Idle") -> (s? t:f=w4176:T1)
              }
              event User Event {
                n1965 = event-data() -> ("IP"=w4181:string, "CMD"=w4186:T3, "Data"=w4185:T6)  [unwired: 1 in]
                n1966 = global read "Global - IP Address.vi" "IP"() -> (w4184:string[])
                n1967 = Index Array(array=w4184, index=7) -> (element=w4182:string)
                n1968 = Equal?(x=w4182, y=w4181) -> (x = y?=w4180:bool)
                n1969 = Bundle By Name(cluster=w4187, "UDP CMD.IP"=w4181, "UDP CMD.CMD"=w4186, "Data"=w4185) -> (w4188:T5)
                n1970 = Select(t=Communications_-_State."Command" ("f"), s=w4180, f=Communications_-_State."Idle") -> (s? t:f=w4178:T1)
              }
            }
            n1971 = global read "Global - Hold.vi" "Hold"() -> (w4165:bool)
            n1972 = Select(t=Communications_-_State."Idle", s=w4165, f=w4164) -> (s? t:f=w4163:T1)
          }
          frame "Command" {
            (unwired) UDP_-_Command."Stop" ("Enum")
            (unwired) 20
            n1973 = Unbundle By Name(w4205) -> ("UDP CMD.CMD"=w4202:T3, "Data"=w4204:T6, "UDP CMD.IP"=w4199:string)
            n1974 = global read "Global - Handle.vi" "Handle"() -> (w4194:T7)
            n1975 = global read "Global - IP Address.vi" "IP"() -> (w4192:string[])
            n1976 = Search 1D Array(1D array=w4192, element=w4199) -> (index of element=w4190:i32)  [unwired: 1 in]
            n1977 = Index Array(array=w4194, index=w4190) -> (element=w4198:T8)
            n1978 = call "UDP - Write CMD.vi"("CMD"=w4202, "error in"=w4206, "Data"=w4204, "UDP Info"=w4198) -> ("error out"=w4196:errorcluster, "IP Address"=w4191:string, "Data Out"=w4201:T11, "Success"=w4200:bool)  [unwired: 2 in, 2 out]
            n1979 = Wait (ms)(milliseconds to wait=u32 5) -> ()  [unwired: 1 out]
            n1980 = Search 1D Array(1D array=w4192, element=w4191) -> (index of element=w4189:i32)  [unwired: 1 in]
            n1981 = global read "Global - Done.vi" "Done"() -> (w4197:bool[])
            n1982 = Replace Array Subset(array=w4197, new element=w4200, index=w4189) -> (w4195:bool[])
            n1983 = global write "Global - Done.vi" "Done"(w4195) -> ()
            n1984 = case shown="True" w4200 {
              tunnel: w4196 -> [w4208 w4214]
              tunnel: [w4209 w4213] -> w4203
              tunnel: w4202 -> [_ w4215]
              tunnel: w4201 -> [_ w4212]
              tunnel: w4189 -> [_ w4211]
              frame False {
                n1985 = call "Communication - Trigger Read IP Address(FGV).vi"("Action"=eFGV_States."Write", "error in"=w4208) -> ("error out"=w4209:errorcluster)  [unwired: 7 in, 2 out]
              }
              frame True {
                n1986 = case shown="\"Read Ch Data\"" w4215 {
                  tunnel: w4214 -> [w4216 w4223 w4230 w4236 w4242 w4248 w4254]
                  tunnel: [w4216 w4223 w4230 w4236 w4242 w4248 w4254] -> w4213
                  tunnel: w4212 -> [_ w4221 w4227 w4235 w4241 w4247 w4253]
                  tunnel: w4211 -> [_ w4225 w4231 w4237 w4243 w4249 w4255]
                  frame "Stop", Default {
                  }
                  frame "Read Ch Data" {
                    n1987 = Unbundle By Name(w4221) -> ("Channels"=w4220:T12, "Event"=w4219:T10, "Status"=w4218:T9)
                    n1988 = global read "Global - Channel.vi" "Data"() -> (w4224:T13)
                    n1989 = Bundle("Channels"=w4220, "Event"=w4219, "Status"=w4218) -> (w4217:T14)  [unwired: 1 in]
                    n1990 = Replace Array Subset(array=w4224, new element=w4217, index=w4225) -> (w4222:T13)
                    n1991 = global write "Global - Channel.vi" "Data"(w4222) -> ()
                  }
                  frame "Read Sensor" {
                    n1992 = Unbundle By Name(w4227) -> ("Sensor"=w4226:T15)
                    n1993 = global read "Global - Unit.vi" "Unit"() -> (w4228:T16)
                    n1994 = Replace Array Subset(array=w4228, new element=w4226, index=w4231) -> (w4229:T16)
                    n1995 = global write "Global - Unit.vi" "Unit"(w4229) -> ()
                  }
                  frame "Read ADC" {
                    n1996 = Unbundle By Name(w4235) -> ("ADC"=w4232:T17)
                    n1997 = global read "Global - ADC.vi" "ADC"() -> (w4234:T18)
                    n1998 = Replace Array Subset(array=w4234, new element=w4232, index=w4237) -> (w4233:T18)
                    n1999 = global write "Global - ADC.vi" "ADC"(w4233) -> ()
                  }
                  frame "Read PID" {
                    n2000 = Unbundle By Name(w4241) -> ("PID"=w4238:T19)
                    n2001 = global read "Global - PID.vi" "PID"() -> (w4240:T20)
                    n2002 = Replace Array Subset(array=w4240, new element=w4238, index=w4243) -> (w4239:T20)
                    n2003 = global write "Global - PID.vi" "PID"(w4239) -> ()
                  }
                  frame "Read System" {
                    n2004 = Unbundle By Name(w4247) -> ("System"=w4245:T21)
                    n2005 = global read "Global - System.vi" "System"() -> (w4246:T22)
                    n2006 = Replace Array Subset(array=w4246, new element=w4245, index=w4249) -> (w4244:T22)
                    n2007 = global write "Global - System.vi" "System"(w4244) -> ()
                  }
                  frame "Read Test" {
                    n2008 = Unbundle By Name(w4253) -> ("Test"=w4250:T23)
                    n2009 = global read "Global - Test.vi" "Test"() -> (w4251:T24)
                    n2010 = Replace Array Subset(array=w4251, new element=w4250, index=w4255) -> (w4252:T24)
                    n2011 = global write "Global - Test.vi" "Test"(w4252) -> ()
                  }
                }
              }
            }
          }
          frame "Close" {
          }
        }
      }
      frame Error {
        n2012 = global read "Global - IP Address.vi" "IP"() -> (w4268:string[])
        n2013 = Unbundle By Name(w4269) -> ("source"=w4264:string)
        n2014 = Index Array(array=w4268, index=0) -> (element=w4266:string)
        n2015 = Concatenate Strings(w4266, " - " ("string"), w4264) -> (w4260:string)
        n2016 = call <vilib>:"Clear Errors.vi"("error in (no error)"=w4269) -> ("error out"=w4263:errorcluster)  [unwired: 5 in, 1 out]
        n2017 = call "General - Error Log eFGV.vi"("eFGV States"=eFGV_States."Write", "error in (no error)"=w4263, "Error In"=w4260) -> ("error out"=w4262:errorcluster)  [unwired: 6 in, 2 out]
        n2018 = Wait (ms)(milliseconds to wait=u32 100) -> ()  [unwired: 1 out]
      }
    }
  }
  n2019 = while {
    shift-right: [w4278] -> _
    shift-left: errorcluster {"status"=FALSE, "code"=0, "source"=""} ("error IO") -> [w4279]
    shift-right: [w4276] -> _
    shift-left: Communications_-_State."Init" -> [w4277]
    shift-right: [w4274] -> _
    shift-left: _ -> [w4273]
    stop <- w4275 stop-if-true
    # "Command Processing Loop"
    n2020 = case shown="No Error" w4279 {
      selector: w4279 -> [w4285 w4403]
      tunnel: [w4286 w4396] -> w4278
      tunnel: w4277 -> [w4284 _]
      tunnel: [w4283 Communications_-_State."Idle"] -> w4276
      tunnel: [w4282 _] -> w4275
      tunnel: [w4281 w4405] -> w4274
      tunnel: w4273 -> [w4280 w4405]
      frame No Error {
        n2021 = case shown="\"Idle\"" w4284 {
          tunnel: [w4289 w4303 w4337 w4393] -> w4286
          tunnel: w4285 -> [w4294 w4302 w4340 w4393]
          tunnel: [Communications_-_State."Idle" w4297 Communications_-_State."Idle" Communications_-_State."Close"] -> w4283
          tunnel: [_ _ _ TRUE] -> w4282
          tunnel: [w4291 w4301 w4339 w4390] -> w4281
          tunnel: w4280 -> [_ w4300 w4339 w4390]
          frame "Init", Default {
            n2022 = call "Communication - UDP Command (eFGV).vi"("Action"=eFGV_States."Read", "error in"=w4294) -> ("error out"=w4290:errorcluster, "UDP Ref"=w4288:refnum<user-event>)  [unwired: 7 in, 1 out]
            n2023 = register-events(error in=w4290, w4288) -> (reference out=w4287:refnum<event-registration>, error out=w4289:errorcluster)  [unwired: 1 in]
            n2024 = Bundle By Name(cluster=T5 {"UDP CMD"={"IP"="", "CMD"=enum."Stop", "Port"="", "Datalog?"=FALSE, "Float"=0.0}, "UDP ref"=refnum, "Unit?"=FALSE, "Read Unit"=[], "Trig?"=FALSE, "UDP Info"=[], "UDP Conn ref"=refnum, "DataLogger"=[], "VISA Ref"=refnum, "Float"=0.0, "Data"={"Test"={"Target Load"=0.0, "Target Disp"=0.0, "Rate"=0.0, "Speed"=0.0}, "Sensor"={"Name"=[], "Unit"=[], "Decimal Point"=[], "Ch Log"=[], "H Alarm"=[], "L Alarm"=[], "H Limit"=[], "L Limit"=[], "Filter"=[], "Gain"=[], "Calib Type"=[]}, "PID"={"SP"=0.0, "PV"=0.0, "kP"=0.0, "kI"=0.0, "kD"=0.0, "FF"=0.0, "Err Band"=0.0, "Max"=0, "Min"=0, "Ts"=0, "Out"=0, "Mode"=0}, "ADC"={"Active Ch"=[], "Filter Type"=0, "Post Filter"=[], "Gain"=[], "FS"=0, "IntOC"=0, "IntFC"=0, "SysOC"=0, "Cofficient"=[], "K"=[], "Max"=0}, "System"={"Out Type"=0, "Inverse"=0, "Monitor"=0, "Reserve"=0, "ACC Time"=0, "Pulse Rev"=0, "Stroke"=0, "Auto Off"=0, "Gear Ratio"=0.0, "Pitch"=0.0, "Max Speed"=0, "Jog Speed"=0, "Disp Coff"=0.0, "Max Load"=0}, "Index"=enum."Ch1", "Datalog"=enum."Empty"}}, "UDP ref"=w4287) -> (w4291:T5)
          }
          frame "Idle" {
            n2025 = Unbundle By Name(w4300) -> ("UDP ref"=w4304:refnum<event-registration>)
            n2026 = event shown="[1] <FDTI ref>: User Event" {
              selector: w4304 -> [_ _]
              dyn-events: _ -> [_ _]
              timeout: _ -> [_ _]
              tunnel: [w4310 w4312] -> w4298
              tunnel: [w4307 _] -> w4303
              tunnel: w4302 -> [w4307 _]
              tunnel: [w4305 w4322] -> w4301
              tunnel: w4300 -> [w4305 w4321]
              event Timeout {
                n2027 = event-data() -> ()  [unwired: 1 in, 1 out]
                n2028 = local read "Stop"() -> (w4309:bool)
                n2029 = Select(t=Communications_-_State."Close", s=w4309, f=Communications_-_State."Idle") -> (s? t:f=w4310:T1)
              }
              event User Event {
                n2030 = event-data() -> ("IP"=w4315:string, "CMD"=w4320:T3, "Data"=w4319:T6)  [unwired: 1 in]
                n2031 = global read "Global - IP Address.vi" "IP"() -> (w4318:string[])
                n2032 = Index Array(array=w4318, index=1) -> (element=w4316:string)
                n2033 = Equal?(x=w4316, y=w4315) -> (x = y?=w4314:bool)
                n2034 = Bundle By Name(cluster=w4321, "UDP CMD.IP"=w4315, "UDP CMD.CMD"=w4320, "Data"=w4319) -> (w4322:T5)
                n2035 = Select(t=Communications_-_State."Command" ("f"), s=w4314, f=Communications_-_State."Idle") -> (s? t:f=w4312:T1)
              }
            }
            n2036 = global read "Global - Hold.vi" "Hold"() -> (w4299:bool)
            n2037 = Select(t=Communications_-_State."Idle", s=w4299, f=w4298) -> (s? t:f=w4297:T1)
          }
          frame "Command" {
            (unwired) UDP_-_Command."Stop" ("Enum")
            (unwired) 20
            n2038 = Unbundle By Name(w4339) -> ("UDP CMD.CMD"=w4336:T3, "Data"=w4338:T6, "UDP CMD.IP"=w4333:string)
            n2039 = global read "Global - Handle.vi" "Handle"() -> (w4328:T7)
            n2040 = global read "Global - IP Address.vi" "IP"() -> (w4326:string[])
            n2041 = Search 1D Array(1D array=w4326, element=w4333) -> (index of element=w4324:i32)  [unwired: 1 in]
            n2042 = Index Array(array=w4328, index=w4324) -> (element=w4332:T8)
            n2043 = call "UDP - Write CMD.vi"("CMD"=w4336, "error in"=w4340, "Data"=w4338, "UDP Info"=w4332) -> ("error out"=w4330:errorcluster, "IP Address"=w4325:string, "Data Out"=w4335:T11, "Success"=w4334:bool)  [unwired: 2 in, 2 out]
            n2044 = Wait (ms)(milliseconds to wait=u32 5) -> ()  [unwired: 1 out]
            n2045 = Search 1D Array(1D array=w4326, element=w4325) -> (index of element=w4323:i32)  [unwired: 1 in]
            n2046 = global read "Global - Done.vi" "Done"() -> (w4331:bool[])
            n2047 = Replace Array Subset(array=w4331, new element=w4334, index=w4323) -> (w4329:bool[])
            n2048 = global write "Global - Done.vi" "Done"(w4329) -> ()
            n2049 = case shown="True" w4334 {
              tunnel: w4330 -> [w4342 w4348]
              tunnel: [w4343 w4347] -> w4337
              tunnel: w4336 -> [_ w4349]
              tunnel: w4335 -> [_ w4346]
              tunnel: w4323 -> [_ w4345]
              frame False {
                n2050 = call "Communication - Trigger Read IP Address(FGV).vi"("Action"=eFGV_States."Write", "error in"=w4342) -> ("error out"=w4343:errorcluster)  [unwired: 7 in, 2 out]
              }
              frame True {
                n2051 = case shown="\"Read Ch Data\"" w4349 {
                  tunnel: w4348 -> [w4350 w4357 w4364 w4370 w4376 w4382 w4388]
                  tunnel: [w4350 w4357 w4364 w4370 w4376 w4382 w4388] -> w4347
                  tunnel: w4346 -> [_ w4355 w4361 w4369 w4375 w4381 w4387]
                  tunnel: w4345 -> [_ w4359 w4365 w4371 w4377 w4383 w4389]
                  frame "Stop", Default {
                  }
                  frame "Read Ch Data" {
                    n2052 = Unbundle By Name(w4355) -> ("Channels"=w4354:T12, "Event"=w4353:T10, "Status"=w4352:T9)
                    n2053 = global read "Global - Channel.vi" "Data"() -> (w4358:T13)
                    n2054 = Bundle("Channels"=w4354, "Event"=w4353, "Status"=w4352) -> (w4351:T14)  [unwired: 1 in]
                    n2055 = Replace Array Subset(array=w4358, new element=w4351, index=w4359) -> (w4356:T13)
                    n2056 = global write "Global - Channel.vi" "Data"(w4356) -> ()
                  }
                  frame "Read Sensor" {
                    n2057 = Unbundle By Name(w4361) -> ("Sensor"=w4360:T15)
                    n2058 = global read "Global - Unit.vi" "Unit"() -> (w4362:T16)
                    n2059 = Replace Array Subset(array=w4362, new element=w4360, index=w4365) -> (w4363:T16)
                    n2060 = global write "Global - Unit.vi" "Unit"(w4363) -> ()
                  }
                  frame "Read ADC" {
                    n2061 = Unbundle By Name(w4369) -> ("ADC"=w4366:T17)
                    n2062 = global read "Global - ADC.vi" "ADC"() -> (w4368:T18)
                    n2063 = Replace Array Subset(array=w4368, new element=w4366, index=w4371) -> (w4367:T18)
                    n2064 = global write "Global - ADC.vi" "ADC"(w4367) -> ()
                  }
                  frame "Read PID" {
                    n2065 = Unbundle By Name(w4375) -> ("PID"=w4372:T19)
                    n2066 = global read "Global - PID.vi" "PID"() -> (w4374:T20)
                    n2067 = Replace Array Subset(array=w4374, new element=w4372, index=w4377) -> (w4373:T20)
                    n2068 = global write "Global - PID.vi" "PID"(w4373) -> ()
                  }
                  frame "Read System" {
                    n2069 = Unbundle By Name(w4381) -> ("System"=w4379:T21)
                    n2070 = global read "Global - System.vi" "System"() -> (w4380:T22)
                    n2071 = Replace Array Subset(array=w4380, new element=w4379, index=w4383) -> (w4378:T22)
                    n2072 = global write "Global - System.vi" "System"(w4378) -> ()
                  }
                  frame "Read Test" {
                    n2073 = Unbundle By Name(w4387) -> ("Test"=w4384:T23)
                    n2074 = global read "Global - Test.vi" "Test"() -> (w4385:T24)
                    n2075 = Replace Array Subset(array=w4385, new element=w4384, index=w4389) -> (w4386:T24)
                    n2076 = global write "Global - Test.vi" "Test"(w4386) -> ()
                  }
                }
              }
            }
          }
          frame "Close" {
          }
        }
      }
      frame Error {
        n2077 = global read "Global - IP Address.vi" "IP"() -> (w4402:string[])
        n2078 = Unbundle By Name(w4403) -> ("source"=w4398:string)
        n2079 = Index Array(array=w4402, index=0) -> (element=w4400:string)
        n2080 = Concatenate Strings(w4400, " - " ("string"), w4398) -> (w4394:string)
        n2081 = call <vilib>:"Clear Errors.vi"("error in (no error)"=w4403) -> ("error out"=w4397:errorcluster)  [unwired: 5 in, 1 out]
        n2082 = call "General - Error Log eFGV.vi"("eFGV States"=eFGV_States."Write", "error in (no error)"=w4397, "Error In"=w4394) -> ("error out"=w4396:errorcluster)  [unwired: 6 in, 2 out]
        n2083 = Wait (ms)(milliseconds to wait=u32 100) -> ()  [unwired: 1 out]
      }
    }
  }
  n2084 = while {
    shift-right: [w4412] -> _
    shift-left: errorcluster {"status"=FALSE, "code"=0, "source"=""} ("error IO") -> [w4413]
    shift-right: [w4410] -> _
    shift-left: Communications_-_State."Init" -> [w4411]
    shift-right: [w4408] -> _
    shift-left: _ -> [w4407]
    stop <- w4409 stop-if-true
    # "Command Processing Loop"
    n2085 = case shown="No Error" w4413 {
      selector: w4413 -> [w4419 w4537]
      tunnel: [w4420 w4530] -> w4412
      tunnel: w4411 -> [w4418 _]
      tunnel: [w4417 Communications_-_State."Idle"] -> w4410
      tunnel: [w4416 _] -> w4409
      tunnel: [w4415 w4539] -> w4408
      tunnel: w4407 -> [w4414 w4539]
      frame No Error {
        n2086 = case shown="\"Idle\"" w4418 {
          tunnel: [w4423 w4437 w4471 w4527] -> w4420
          tunnel: w4419 -> [w4428 w4436 w4474 w4527]
          tunnel: [Communications_-_State."Idle" w4431 Communications_-_State."Idle" Communications_-_State."Close"] -> w4417
          tunnel: [_ _ _ TRUE] -> w4416
          tunnel: [w4425 w4435 w4473 w4524] -> w4415
          tunnel: w4414 -> [_ w4434 w4473 w4524]
          frame "Init", Default {
            n2087 = call "Communication - UDP Command (eFGV).vi"("Action"=eFGV_States."Read", "error in"=w4428) -> ("error out"=w4424:errorcluster, "UDP Ref"=w4422:refnum<user-event>)  [unwired: 7 in, 1 out]
            n2088 = register-events(error in=w4424, w4422) -> (reference out=w4421:refnum<event-registration>, error out=w4423:errorcluster)  [unwired: 1 in]
            n2089 = Bundle By Name(cluster=T5 {"UDP CMD"={"IP"="", "CMD"=enum."Stop", "Port"="", "Datalog?"=FALSE, "Float"=0.0}, "UDP ref"=refnum, "Unit?"=FALSE, "Read Unit"=[], "Trig?"=FALSE, "UDP Info"=[], "UDP Conn ref"=refnum, "DataLogger"=[], "VISA Ref"=refnum, "Float"=0.0, "Data"={"Test"={"Target Load"=0.0, "Target Disp"=0.0, "Rate"=0.0, "Speed"=0.0}, "Sensor"={"Name"=[], "Unit"=[], "Decimal Point"=[], "Ch Log"=[], "H Alarm"=[], "L Alarm"=[], "H Limit"=[], "L Limit"=[], "Filter"=[], "Gain"=[], "Calib Type"=[]}, "PID"={"SP"=0.0, "PV"=0.0, "kP"=0.0, "kI"=0.0, "kD"=0.0, "FF"=0.0, "Err Band"=0.0, "Max"=0, "Min"=0, "Ts"=0, "Out"=0, "Mode"=0}, "ADC"={"Active Ch"=[], "Filter Type"=0, "Post Filter"=[], "Gain"=[], "FS"=0, "IntOC"=0, "IntFC"=0, "SysOC"=0, "Cofficient"=[], "K"=[], "Max"=0}, "System"={"Out Type"=0, "Inverse"=0, "Monitor"=0, "Reserve"=0, "ACC Time"=0, "Pulse Rev"=0, "Stroke"=0, "Auto Off"=0, "Gear Ratio"=0.0, "Pitch"=0.0, "Max Speed"=0, "Jog Speed"=0, "Disp Coff"=0.0, "Max Load"=0}, "Index"=enum."Ch1", "Datalog"=enum."Empty"}}, "UDP ref"=w4421) -> (w4425:T5)
          }
          frame "Idle" {
            n2090 = Unbundle By Name(w4434) -> ("UDP ref"=w4438:refnum<event-registration>)
            n2091 = event shown="[1] <FDTI ref>: User Event" {
              selector: w4438 -> [_ _]
              dyn-events: _ -> [_ _]
              timeout: _ -> [_ _]
              tunnel: [w4444 w4446] -> w4432
              tunnel: [w4441 _] -> w4437
              tunnel: w4436 -> [w4441 _]
              tunnel: [w4439 w4456] -> w4435
              tunnel: w4434 -> [w4439 w4455]
              event Timeout {
                n2092 = event-data() -> ()  [unwired: 1 in, 1 out]
                n2093 = local read "Stop"() -> (w4443:bool)
                n2094 = Select(t=Communications_-_State."Close", s=w4443, f=Communications_-_State."Idle") -> (s? t:f=w4444:T1)
              }
              event User Event {
                n2095 = event-data() -> ("IP"=w4449:string, "CMD"=w4454:T3, "Data"=w4453:T6)  [unwired: 1 in]
                n2096 = global read "Global - IP Address.vi" "IP"() -> (w4452:string[])
                n2097 = Index Array(array=w4452, index=3) -> (element=w4450:string)
                n2098 = Equal?(x=w4450, y=w4449) -> (x = y?=w4448:bool)
                n2099 = Bundle By Name(cluster=w4455, "UDP CMD.IP"=w4449, "UDP CMD.CMD"=w4454, "Data"=w4453) -> (w4456:T5)
                n2100 = Select(t=Communications_-_State."Command" ("f"), s=w4448, f=Communications_-_State."Idle") -> (s? t:f=w4446:T1)
              }
            }
            n2101 = global read "Global - Hold.vi" "Hold"() -> (w4433:bool)
            n2102 = Select(t=Communications_-_State."Idle", s=w4433, f=w4432) -> (s? t:f=w4431:T1)
          }
          frame "Command" {
            (unwired) UDP_-_Command."Stop" ("Enum")
            (unwired) 20
            n2103 = Unbundle By Name(w4473) -> ("UDP CMD.CMD"=w4470:T3, "Data"=w4472:T6, "UDP CMD.IP"=w4467:string)
            n2104 = global read "Global - Handle.vi" "Handle"() -> (w4462:T7)
            n2105 = global read "Global - IP Address.vi" "IP"() -> (w4460:string[])
            n2106 = Search 1D Array(1D array=w4460, element=w4467) -> (index of element=w4458:i32)  [unwired: 1 in]
            n2107 = Index Array(array=w4462, index=w4458) -> (element=w4466:T8)
            n2108 = call "UDP - Write CMD.vi"("CMD"=w4470, "error in"=w4474, "Data"=w4472, "UDP Info"=w4466) -> ("error out"=w4464:errorcluster, "IP Address"=w4459:string, "Data Out"=w4469:T11, "Success"=w4468:bool)  [unwired: 2 in, 2 out]
            n2109 = Wait (ms)(milliseconds to wait=u32 5) -> ()  [unwired: 1 out]
            n2110 = Search 1D Array(1D array=w4460, element=w4459) -> (index of element=w4457:i32)  [unwired: 1 in]
            n2111 = global read "Global - Done.vi" "Done"() -> (w4465:bool[])
            n2112 = Replace Array Subset(array=w4465, new element=w4468, index=w4457) -> (w4463:bool[])
            n2113 = global write "Global - Done.vi" "Done"(w4463) -> ()
            n2114 = case shown="True" w4468 {
              tunnel: w4464 -> [w4476 w4482]
              tunnel: [w4477 w4481] -> w4471
              tunnel: w4470 -> [_ w4483]
              tunnel: w4469 -> [_ w4480]
              tunnel: w4457 -> [_ w4479]
              frame False {
                n2115 = call "Communication - Trigger Read IP Address(FGV).vi"("Action"=eFGV_States."Write", "error in"=w4476) -> ("error out"=w4477:errorcluster)  [unwired: 7 in, 2 out]
              }
              frame True {
                n2116 = case shown="\"Read Ch Data\"" w4483 {
                  tunnel: w4482 -> [w4484 w4491 w4498 w4504 w4510 w4516 w4522]
                  tunnel: [w4484 w4491 w4498 w4504 w4510 w4516 w4522] -> w4481
                  tunnel: w4480 -> [_ w4489 w4495 w4503 w4509 w4515 w4521]
                  tunnel: w4479 -> [_ w4493 w4499 w4505 w4511 w4517 w4523]
                  frame "Stop", Default {
                  }
                  frame "Read Ch Data" {
                    n2117 = Unbundle By Name(w4489) -> ("Channels"=w4488:T12, "Event"=w4487:T10, "Status"=w4486:T9)
                    n2118 = global read "Global - Channel.vi" "Data"() -> (w4492:T13)
                    n2119 = Bundle("Channels"=w4488, "Event"=w4487, "Status"=w4486) -> (w4485:T14)  [unwired: 1 in]
                    n2120 = Replace Array Subset(array=w4492, new element=w4485, index=w4493) -> (w4490:T13)
                    n2121 = global write "Global - Channel.vi" "Data"(w4490) -> ()
                  }
                  frame "Read Sensor" {
                    n2122 = Unbundle By Name(w4495) -> ("Sensor"=w4494:T15)
                    n2123 = global read "Global - Unit.vi" "Unit"() -> (w4496:T16)
                    n2124 = Replace Array Subset(array=w4496, new element=w4494, index=w4499) -> (w4497:T16)
                    n2125 = global write "Global - Unit.vi" "Unit"(w4497) -> ()
                  }
                  frame "Read ADC" {
                    n2126 = Unbundle By Name(w4503) -> ("ADC"=w4500:T17)
                    n2127 = global read "Global - ADC.vi" "ADC"() -> (w4502:T18)
                    n2128 = Replace Array Subset(array=w4502, new element=w4500, index=w4505) -> (w4501:T18)
                    n2129 = global write "Global - ADC.vi" "ADC"(w4501) -> ()
                  }
                  frame "Read PID" {
                    n2130 = Unbundle By Name(w4509) -> ("PID"=w4506:T19)
                    n2131 = global read "Global - PID.vi" "PID"() -> (w4508:T20)
                    n2132 = Replace Array Subset(array=w4508, new element=w4506, index=w4511) -> (w4507:T20)
                    n2133 = global write "Global - PID.vi" "PID"(w4507) -> ()
                  }
                  frame "Read System" {
                    n2134 = Unbundle By Name(w4515) -> ("System"=w4513:T21)
                    n2135 = global read "Global - System.vi" "System"() -> (w4514:T22)
                    n2136 = Replace Array Subset(array=w4514, new element=w4513, index=w4517) -> (w4512:T22)
                    n2137 = global write "Global - System.vi" "System"(w4512) -> ()
                  }
                  frame "Read Test" {
                    n2138 = Unbundle By Name(w4521) -> ("Test"=w4518:T23)
                    n2139 = global read "Global - Test.vi" "Test"() -> (w4519:T24)
                    n2140 = Replace Array Subset(array=w4519, new element=w4518, index=w4523) -> (w4520:T24)
                    n2141 = global write "Global - Test.vi" "Test"(w4520) -> ()
                  }
                }
              }
            }
          }
          frame "Close" {
          }
        }
      }
      frame Error {
        n2142 = global read "Global - IP Address.vi" "IP"() -> (w4536:string[])
        n2143 = Unbundle By Name(w4537) -> ("source"=w4532:string)
        n2144 = Index Array(array=w4536, index=0) -> (element=w4534:string)
        n2145 = Concatenate Strings(w4534, " - " ("string"), w4532) -> (w4528:string)
        n2146 = call <vilib>:"Clear Errors.vi"("error in (no error)"=w4537) -> ("error out"=w4531:errorcluster)  [unwired: 5 in, 1 out]
        n2147 = call "General - Error Log eFGV.vi"("eFGV States"=eFGV_States."Write", "error in (no error)"=w4531, "Error In"=w4528) -> ("error out"=w4530:errorcluster)  [unwired: 6 in, 2 out]
        n2148 = Wait (ms)(milliseconds to wait=u32 100) -> ()  [unwired: 1 out]
      }
    }
  }
